vi "BIMS_Collector (2015_06).vi"() -> ()   [LabVIEW 2015]
doc: "This program is currently beta software. It is designed to address the data requirements defined primarily by the DHB Ballistic Test Report.\n\nThe general operation of this program is based on the Ballistics Version 2005 application developed internally by DuPont as a research tool for the Spruance Plant Ballistics Lab in Richmond, VA.\n\nPlease note that the original trigger control logic was modified and no longer depends on a safety interlock system to enable operation of a ballistic test.\n\nDuPont makes no warranties and assumes no liabilities in connection with any use of this program."
uses:
  DataSource.ctl
  shotsArr.ctl
  Shot Record.ctl
  Collector State.ctl
  <vilib>/Utility/error.llb/DialogType.ctl
  <vilib>/registry/registry.llb/Registry RtKey.ctl
  <vilib>/DAQmx/read.llb/DAQmx Read (Counter DBL 1Chan 1Samp).vi
  BIMS_Collector Globals.vi
  <vilib>/Utility/config.llb/Write Key (String).vi
  <vilib>/addons/database/Connection.llb/DB Tools Open Connec (Path).vi
  <vilib>/addons/database/Connection.llb/Conn Execute.vi
  <vilib>/addons/database/Recordset.llb/Rec Destroy - Connection.vi
  <vilib>/DAQmx/miscellaneous.llb/DAQmx Fill In Error Info.vi
  <vilib>/addons/database/NI_Database_API.lvlib
  <vilib>/Utility/config.llb/NI_LVConfig.lvlib
  <vilib>/Utility/file.llb/Write To Spreadsheet File (string).vi
panel:
  in  "diagPageVisible":bool
  in  "runtimeMenusVisible":bool=TRUE
  out "loadStatus":string
  out "Loading":u16(ring)
  in  "RESET All":bool
  out "ConfigName":string
  out "TimeNow":string
  in  "EXIT":bool
  in  "mainTabCntrl":enum32{"Setup", "Measure", "History", "System"}(tab)=enum."System"
  in  "SampleEntryTabCntrl":enum32{"Environment", "Sample"}(tab)
  in  "ThreatDetails":u16(ring) caption="Detail"
  in  "ThreatGroups":u16(ring) caption="Group"
  in  "PowderTypes":u16(ring) caption="Type"
  in  "Ballisticians":u16(ring) caption="Laboratorists"
  in  "Recorders":u16(ring) caption="Recorder"
  in  "Shooters":u16(ring) caption="Shooter"
  in  "Methods":u16(ring) caption="Method"
  in  "RoomT":sgl caption="Temperature (° C)" format="%.1f"
  in  "RoomHum":sgl caption="Humidity (%)" min=0 max=100 format="%.1f"
  in  "SampleBackings":u16(ring)=3 caption="Type"
  in  "clayCalArray":i16[](array[numeric])=[0, 0, 0, 0, 0] caption="Calibration (mm)" min=0 max=99 format="%02.0f"
  out "clayAverage":sgl caption="Clay Average (mm)" format="%#.1f"
  in  "clayTemp":sgl caption="Clay Temp (° F)" format="%.1f"
  out "threatDetails":T1 caption="Description"
  in  "SampleClamping":u16(ring) caption="Clamping"
  in  "Sample SubTabCntrl":T2(tab)
  in  "SampleID":string caption="Sample ID"
  in  "SampleDimensions":u16(ring) caption="Dimensions"
  in  "ModelMfrs":u16(ring) caption="Manufacturer"
  in  "SampleTypes":u16(ring) caption="Sample Type"
  in  "Submitters":u16(ring) caption="Submitter"
  in  "ProjectID":string caption="Project ID"
  in  "BackLayers":i32 caption="# of Layers" min=0 max=99 step=5
  in  "FrontLayers":i32 caption="# of Layers" min=0 max=99 step=5
  in  "BackLayer":u16(ring) caption="Back Layer"
  in  "FrontLayer":u16(ring) caption="Front Layer"
  out "totalNumLayers":i32 caption="Total # of Layers" min=0 max=100 step=5
  out "totalBAW":sgl caption="Total BAW (psf)" format="%.2f"
  in  "LayerTabControl":enum32{"1", "2", "3", "4", "5", "6"}(tab) caption="Inner Layers"
  out "fab1_totalWt":sgl caption="Fab1 Wt" min=0 max=99 step=5 format="%.2f"
  out "SampleAttribs_1":T3 caption="fabricAttribs_1"
  in  "Layer_1":T4 caption="Fabric #1" {"plyNum" min=0}
  in  "SampleStyle_1":u16(ring)
  in  "Mfr_1":u16(ring) caption="vendor" items=["", "3M", "A&P Technology", "Absecon Mills", "ABT Sciences", "Aermet", "ArmorStruxx", "Artec", "Axiom", "BAE Advanced Ceramics", "Barrday", "BGF", "Citterio", "Coors-Tek", "DSM", "DuPont", "DuPont (JPS-SUBC)", "FTC", "Gentex", "Gurit", "Hexcel", "Honeywell", "JD Lincoln", "JPS-Alexium", "JPS-Apjet", "JPS-DuPont", "JPS-Huntsman", "JPS-Old Hickory", "JPS-TSG", "Kamenskvolokno", "Loctite", "Lord", "LTC", "Marcus Materials", "McMaster-Carr", "Nanocomp", "Neva", "Nolax", "OConnell", "Patriot 3", "PATZ", "PBO", "Polystrand", "Pro-Systems", "ProTech", "Rusar", "Saati", "Saint Gobain", "S-Bond", "SEAL", "Sioux", "SPDW", "TechFiber", "Teijin", "Tencate", "Tensylon", "TexTech", "Toray", "TWARON", "UNKNOWN", "VonWeiss", "Xymid", "Z11"]
  in  "layerStitch_1":u16(ring) caption="Stitch"
  out "fab2_totalWt":sgl caption="Fab2 Wt" min=0 max=99 step=5 format="%.2f"
  out "SampleAttribs_2":T3 caption="fabricAttribs_2"
  in  "Layer_2":T4 caption="Fabric #2" {"plyNum" min=0}
  in  "SampleStyle_2":u16(ring)
  in  "Mfr_2":u16(ring) caption="vendor" items=["", "3M", "A&P Technology", "Absecon Mills", "ABT Sciences", "Aermet", "ArmorStruxx", "Artec", "Axiom", "BAE Advanced Ceramics", "Barrday", "BGF", "Citterio", "Coors-Tek", "DSM", "DuPont", "DuPont (JPS-SUBC)", "FTC", "Gentex", "Gurit", "Hexcel", "Honeywell", "JD Lincoln", "JPS-Alexium", "JPS-Apjet", "JPS-DuPont", "JPS-Huntsman", "JPS-Old Hickory", "JPS-TSG", "Kamenskvolokno", "Loctite", "Lord", "LTC", "Marcus Materials", "McMaster-Carr", "Nanocomp", "Neva", "Nolax", "OConnell", "Patriot 3", "PATZ", "PBO", "Polystrand", "Pro-Systems", "ProTech", "Rusar", "Saati", "Saint Gobain", "S-Bond", "SEAL", "Sioux", "SPDW", "TechFiber", "Teijin", "Tencate", "Tensylon", "TexTech", "Toray", "TWARON", "UNKNOWN", "VonWeiss", "Xymid", "Z11"]
  in  "layerStitch_2":u16(ring) caption="Stitch"
  out "fab3_totalWt":sgl caption="Fab3 Wt" min=0 max=99 step=5 format="%.2f"
  out "SampleAttribs_3":T3 caption="fabricAttribs_3"
  in  "Layer_3":T4 caption="Fabric #3" {"plyNum" min=0}
  in  "SampleStyle_3":u16(ring)
  in  "Mfr_3":u16(ring) caption="vendor" items=["", "3M", "A&P Technology", "Absecon Mills", "ABT Sciences", "Aermet", "ArmorStruxx", "Artec", "Axiom", "BAE Advanced Ceramics", "Barrday", "BGF", "Citterio", "Coors-Tek", "DSM", "DuPont", "DuPont (JPS-SUBC)", "FTC", "Gentex", "Gurit", "Hexcel", "Honeywell", "JD Lincoln", "JPS-Alexium", "JPS-Apjet", "JPS-DuPont", "JPS-Huntsman", "JPS-Old Hickory", "JPS-TSG", "Kamenskvolokno", "Loctite", "Lord", "LTC", "Marcus Materials", "McMaster-Carr", "Nanocomp", "Neva", "Nolax", "OConnell", "Patriot 3", "PATZ", "PBO", "Polystrand", "Pro-Systems", "ProTech", "Rusar", "Saati", "Saint Gobain", "S-Bond", "SEAL", "Sioux", "SPDW", "TechFiber", "Teijin", "Tencate", "Tensylon", "TexTech", "Toray", "TWARON", "UNKNOWN", "VonWeiss", "Xymid", "Z11"]
  in  "layerStitch_3":u16(ring) caption="Stitch"
  out "fab4_totalWt":sgl caption="Fab4 Wt" min=0 max=99 step=5 format="%.2f"
  out "SampleAttribs_4":T3 caption="fabricAttribs_4"
  in  "Layer_4":T4 caption="Fabric #4" {"plyNum" min=0}
  in  "SampleStyle_4":u16(ring)
  in  "Mfr_4":u16(ring) caption="vendor" items=["", "3M", "A&P Technology", "Absecon Mills", "ABT Sciences", "Aermet", "ArmorStruxx", "Artec", "Axiom", "BAE Advanced Ceramics", "Barrday", "BGF", "Citterio", "Coors-Tek", "DSM", "DuPont", "DuPont (JPS-SUBC)", "FTC", "Gentex", "Gurit", "Hexcel", "Honeywell", "JD Lincoln", "JPS-Alexium", "JPS-Apjet", "JPS-DuPont", "JPS-Huntsman", "JPS-Old Hickory", "JPS-TSG", "Kamenskvolokno", "Loctite", "Lord", "LTC", "Marcus Materials", "McMaster-Carr", "Nanocomp", "Neva", "Nolax", "OConnell", "Patriot 3", "PATZ", "PBO", "Polystrand", "Pro-Systems", "ProTech", "Rusar", "Saati", "Saint Gobain", "S-Bond", "SEAL", "Sioux", "SPDW", "TechFiber", "Teijin", "Tencate", "Tensylon", "TexTech", "Toray", "TWARON", "UNKNOWN", "VonWeiss", "Xymid", "Z11"]
  in  "layerStitch_4":u16(ring) caption="Stitch"
  out "fab5_totalWt":sgl caption="Fab5 Wt" min=0 max=99 step=5 format="%.2f"
  out "SampleAttribs_5":T3 caption="fabricAttribs_5"
  in  "Layer_5":T4 caption="Fabric #5" {"plyNum" min=0}
  in  "SampleStyle_5":u16(ring)
  in  "Mfr_5":u16(ring) caption="vendor" items=["", "3M", "A&P Technology", "Absecon Mills", "ABT Sciences", "Aermet", "ArmorStruxx", "Artec", "Axiom", "BAE Advanced Ceramics", "Barrday", "BGF", "Citterio", "Coors-Tek", "DSM", "DuPont", "DuPont (JPS-SUBC)", "FTC", "Gentex", "Gurit", "Hexcel", "Honeywell", "JD Lincoln", "JPS-Alexium", "JPS-Apjet", "JPS-DuPont", "JPS-Huntsman", "JPS-Old Hickory", "JPS-TSG", "Kamenskvolokno", "Loctite", "Lord", "LTC", "Marcus Materials", "McMaster-Carr", "Nanocomp", "Neva", "Nolax", "OConnell", "Patriot 3", "PATZ", "PBO", "Polystrand", "Pro-Systems", "ProTech", "Rusar", "Saati", "Saint Gobain", "S-Bond", "SEAL", "Sioux", "SPDW", "TechFiber", "Teijin", "Tencate", "Tensylon", "TexTech", "Toray", "TWARON", "UNKNOWN", "VonWeiss", "Xymid", "Z11"]
  in  "layerStitch_5":u16(ring) caption="Stitch"
  out "fab6_totalWt":sgl caption="Fab6 Wt" min=0 max=99 step=5 format="%.2f"
  out "SampleAttribs_6":T3 caption="fabricAttribs_6"
  in  "Layer_6":T4 caption="Fabric #6" {"plyNum" min=0}
  in  "SampleStyle_6":u16(ring)
  in  "Mfr_6":u16(ring) caption="vendor" items=["", "3M", "A&P Technology", "Absecon Mills", "ABT Sciences", "Aermet", "ArmorStruxx", "Artec", "Axiom", "BAE Advanced Ceramics", "Barrday", "BGF", "Citterio", "Coors-Tek", "DSM", "DuPont", "DuPont (JPS-SUBC)", "FTC", "Gentex", "Gurit", "Hexcel", "Honeywell", "JD Lincoln", "JPS-Alexium", "JPS-Apjet", "JPS-DuPont", "JPS-Huntsman", "JPS-Old Hickory", "JPS-TSG", "Kamenskvolokno", "Loctite", "Lord", "LTC", "Marcus Materials", "McMaster-Carr", "Nanocomp", "Neva", "Nolax", "OConnell", "Patriot 3", "PATZ", "PBO", "Polystrand", "Pro-Systems", "ProTech", "Rusar", "Saati", "Saint Gobain", "S-Bond", "SEAL", "Sioux", "SPDW", "TechFiber", "Teijin", "Tencate", "Tensylon", "TexTech", "Toray", "TWARON", "UNKNOWN", "VonWeiss", "Xymid", "Z11"]
  in  "layerStitch_6":u16(ring) caption="Stitch"
  in  "SampleCoverings":u16(ring) caption="Sample Covering" items=["None", "RipStop", "Plastic bag", "Other"]
  in  "Assemblers":u16(ring) caption="Technician"
  in  "Thickness":dbl caption="Thickness (mm)" format="%.3f"
  in  "totalSampleWt":sgl caption="Total Weight (g)" format="%.3f"
  in  "Comments":string caption="Remarks (optional):"
  in  "TestConditions":u16(ring) caption="Sample Condition"
  in  "shotsTabCntrl":T5(tab)
  in  "2ndScreen":bool=TRUE caption="Enabled"
  out "cntDn":i32
  in  "Frag Rod":sgl format="%.1f"
  in  "Drag Corrected":bool=TRUE
  out "Impact/speed":sgl caption="Chronograph 1" min=0 max=10000 step=0.1 format="%.1f"
  out "residual/speed":sgl caption="Residual" min=0 max=10000 step=0.1 format="%.1f"
  in  "MeasVelScrnSet1":sgl caption="Set #1" min=0 max=10000 step=0.1 format="%.1f"
  in  "Current/shotstatus":u16(ring) caption="Penetration" items=["Partial", "Complete"]
  in  "Current/residual/speed":sgl caption="Residual Set" min=0 max=10000 step=0.1 format="%.1f"
  in  "shotTimestamp":string caption="Date/Time"
  in  "MeasVelScrnSet2":sgl caption="Set #2" min=0 max=1000000 step=0.1 format="%.1f"
  out "%_Difference":sgl caption="% Vel Diff" format="%.3f"
  in  "backdepth":sgl caption="BF Depth"
  out "Redundant/speed":sgl caption="Chronograph 2" min=0 max=10000 step=0.1 format="%.1f"
  out "Current/avg/speed":sgl caption="Average" min=0 max=1000000 step=0.1 format="%.1f"
  out "Avg/speed":sgl caption="Average" min=0 max=10000 step=0.1 format="%.1f"
  out "DC_ factor":sgl=1.0 caption="DC Factor" format="%.4f"
  in  "Barrel Temp":sgl format="%.1f"
  in  "Shot Description":string caption="Description (optional)"
  in  "Powder Loading":sgl caption="Powder Load" min=0 max=100 step=0.1 format="%.3f"
  in  "Shot Angle":u16 max=90 step=1
  out "Projectile Mass":sgl caption="Projectile Mass (grains)" min=0 step=1
  in  "N.I.J":u16(ring) items=["n/a", "PASS", "FAIL"]
  in  "addShot":bool caption="RANGE SETUP must be selected before shots can be added."
  in  "loadingUnits":enum32{"grams", "grains"}(radio)
  out "instruct_addShot":string="RANGE SETUP and THREAT must be selected before shots can be added."
  out "Set#1 Separation":sgl=1.0 caption="Outer" format="%.2f"
  out "Set#2 Separation":sgl=1.0 caption="Inner" format="%.2f"
  out "ARMED":bool caption="Armed"
  out "velSTDEV":sgl caption="Standard Deviation" min=0 max=10000 step=1 format="%.1f"
  out "saveReq":string="Number of layers in sample ply specification and number of shots in shots table must be greater than 0 to enable saving."
  in  "VsVr Report":bool caption="Report"
  out "Table of Shots":string[][](table) caption="Shot Table"
  in  "MC Listbox of Shots":i32(listbox)
  in  "saveShots":bool
  in  "clearShots":bool
  out "highPartial":i32 caption="High Partial" min=0 max=10000 step=1
  out "lowComplete":i32 caption="Low Complete" min=0 max=10000 step=1
  out "rangeOfResults":i32 caption="Range of Results" min=0 max=10000 step=1
  out "zmr 2":sgl caption="Low C minus High P" format="%.1f"
  out "computed_V50":sgl caption="V50  (m/s)" format="%.1f"
  out "Pairs":i16 min=0 max=100 step=1
  in  "reportV50":bool caption="Report"
  in  "maxDev":sgl=10.0 caption="Max Deviation (m/s)" min=0 max=100 format="%.1f"
  in  "undoLastShot":bool
  in  "deleteShot":bool
  in  "nextShot":bool
  in  "shotsArr":T6 {"Frag Rod" format="%.1f"; "UncorrectedAvgVel_PB" format="%.1f"; "UncorrectedRed_PB" format="%.1f"; "strikeVel_PB" format="%.1f"; "velLoss_PB" format="%.1f"; "avgVel_PB" format="%.1f"; "Redundant_Velocity" format="%.1f"; "Energy Loss (J)" format="%.3e"; "Projectile Mass" min=0 step=1 format="%.4f"; "Corrected residual" format="%.2f"; "Uncorrected Residual" format="%.1f"; "Corrected Impact" format="%.2f"; "Uncorrected Impact" format="%.1f"; "Shot Angle" max=90 step=1; "SHOT STATUS" items=["Partial", "Complete"]; "IMPACT VELOCITY" min=0 max=10000 step=0.1 format="%.1f"; "Barrel Temperature" format="%.1f"; "Powder Loading" format="%.4f"; "RESIDUAL  VELOCITY" min=0 max=10000 step=0.1 format="%.1f"}
  out "velProfile":cluster{dbl, dbl}[](graph) caption="Shot Velocity Measurement Profile"
  out "velCompProf":cluster{"vStrike":dbl, "vA":dbl} caption="Velocity in fps\n(computed)"
  out "velMeasProf":T8 caption="Velocity in fps\n(measured)"
  out "relativeTime":cluster{"ts2":dbl, "ts3":dbl, "ts1":dbl} caption="Relative time\n(microsec)"
  out "displacement":T9={"ds_v2"=6.75, "ds2"=5.0833, "ds_vB"=4.9167, "ds3"=4.75, "ds_vAvg"=6.9167, "ds_v1"=7.0833, "ds1"=8.75, "ds_vA"=8.9167, "ds0"=9.0833} caption="Distance from\ntarget (ft)" {"ds0" format="%_4g"; "ds_vA" format="%_4g"; "ds1" format="%_4g"; "ds_v1" format="%_4g"; "ds_vAvg" format="%_4g"; "ds3" format="%_4g"; "ds_vB" format="%#_4g"; "ds2" format="%#_4g"; "ds_v2" format="%_4g"}
  out "arrIDC":dbl[](array[numeric]) caption="Instantaneous Drag Coefficient"
  in  "rangeSetup":u16(ring)=1 caption="Range Dimensions" items=["Short (small frag)", "Standard (handgun)", "Long (rifle)"]
  out "mid_to_targ_dist":sgl=5.0 caption="Mid To Target (ft)"
  in  "historyTabCntrl":enum32{"Powder Loading", "Panel Search"}(tab)=enum."Panel Search"
  in  "Threat.freeTxt":string caption="Threat"
  in  "Powder.freeTxt":string caption="Powder"
  in  "QueryLoad":bool
  in  "lkupEndDate":timestamp caption="End Date" format="%<%x>T"
  in  "lkupStartDate":timestamp caption="Begin Date" format="%<%x>T"
  out "Vel.vs.Loading":cluster{dbl[], dbl[]}(graph)
  out "v50_table":string[][](table)
  in  "maxRecs":u16=1001 caption="Max # of SHOT Records" min=1 max=10000 step=100
  out "ActualNumRecs":i32=1001 caption="Actual # Returned"
  in  "ThreatSize_0":u16(ring) caption="Threat Size" items=["", "2", "4", "16", "17", "44", "55", "62", "64", "85", "123", "124", "125", "148", "158", "166", "180", "207", "240"]
  in  "panelSearch":bool
  in  "Mfr_0":u16(ring) caption="Manufacturer" items=["", "3M", "A&P Technology", "Absecon Mills", "ABT Sciences", "Aermet", "ArmorStruxx", "Artec", "Axiom", "BAE Advanced Ceramics", "Barrday", "BGF", "Citterio", "Coors-Tek", "DSM", "DuPont", "DuPont (JPS-SUBC)", "FTC", "Gentex", "Gurit", "Hexcel", "Honeywell", "JD Lincoln", "JPS-Alexium", "JPS-Apjet", "JPS-DuPont", "JPS-Huntsman", "JPS-Old Hickory", "JPS-TSG", "Kamenskvolokno", "Loctite", "Lord", "LTC", "Marcus Materials", "McMaster-Carr", "Nanocomp", "Neva", "Nolax", "OConnell", "Patriot 3", "PATZ", "PBO", "Polystrand", "Pro-Systems", "ProTech", "Rusar", "Saati", "Saint Gobain", "S-Bond", "SEAL", "Sioux", "SPDW", "TechFiber", "Teijin", "Tencate", "Tensylon", "TexTech", "Toray", "TWARON", "UNKNOWN", "VonWeiss", "Xymid", "Z11"]
  in  "SampleStyle_0":u16(ring) caption="Sample Style"
  in  "srchParams":T10={"maxPanels"=1001, "lkupPanelStartDate"=timestamp(0 s since 1904-01-01), "lkupPanelEndDate"=timestamp(3376658114.0909824 s since 1904-01-01)} {"lkupPanelEndDate" format="%<%x>T"; "lkupPanelStartDate" format="%<%x>T"; "maxPanels" min=1 max=10000 step=100}
  out "actualNumPanels":i32 caption="Actual # Returned"
  out "pastPanels":string[][](table)
  in  "Record #":i32=1 min=0 max=60857
  in  "reportV50_History":bool
  out "SampleAttribs_0":T11 caption="fabricAttribs_1"
  in  "Requestors_0":u16(ring) caption="Submitter"
  in  "aboutTabCntrl":enum32{"About ", "Internal Use"}(tab)
  in  "RefreshMetadata":bool
  out "lastShot":i32 caption="Shot"
  out "lastSamp":i32 caption="Sample"
  in  "PublishNewRecords":bool
  in  "internal":enum32{"ctr", "deploy", "misc"}(tab)=enum."misc"
  out "taskCtr1":refnum<k21>
  in  "ctr1":tag="LightScreens/ctr1"
  in  "readyClock":bool caption="Clock"
  in  "ActiveDev":tag="LightScreens"
  in  "ctr0":tag="LightScreens/ctr0"
  in  "SampClk.Timebase.Src":tag="/LightScreens/80MHzTimebase"
  out "Device S/N":string
  in  "MeasSrc":T12=enum."Screens" caption="Source"
  in  "ARM":bool
  out "errCtr0":errorcluster
  out "errCtr1":errorcluster
  out "taskCtr0":refnum<k21>
  in  "Folder":string caption="Publish Folder"
  in  "useBMC":bool caption="Use Message Center?"
  in  "Server":string
  in  "Site":string
  in  "InterlockExists":bool=TRUE caption="Safety Interlock Hardware Exist?"
  in  "ScreenSetAvgg":bool=TRUE caption="Average Screen Sets?"
  in  "Sort by AVG":bool=TRUE caption="Sort shots by average velocity"
  in  "useBallisitican":bool=TRUE caption="Use Ballistician field in Setup?"
  in  "useRecorder":bool caption="Use Recorder field in Setup?"
  in  "useShooter":bool caption="Use Shooter field in Setup?"
  in  "close arming loop":bool
  out "progState":T13
  in  "clearErrors":bool
  in  "LayerStitchTypes":u16(ring) caption="Stitch"
  out "GrainSize":u16 caption="Grain"
  out "U/I EvErr":errorcluster
  out "SMErr":errorcluster
  in  "Models":u16(ring) caption="Model #" items=["n/a"]
  in  "serialNum":string caption="Serial #"
  in  "SampleDescrip":u16(ring) caption="Misc. Sample Description (legacy)"
  out "lengthUnits":string="FOOT" caption="Distance Units"
  out "massUnits":string="GRAMS" caption="Weight Units"
  in  "Threat":u16(ring) caption="Threat (long description)"
  in  "Type of work":string="QC"
  in  "minV50":i32=1500 caption="Minimum V50"
  out "configPath":path=path "P:/Private/My Projects/AFS/BIMS/2008/BIMS_Collector.ini" caption="Configuration Path (INI)"
  out "STOP (Shots MC LB)":bool=TRUE
  in  "lookupRec":bool caption="lookup"
  in  "clayCalib":string="##-##-##-##-##" caption="Calibration"
  in  "Fabric Description":string caption="Fabric Desc"
  in  "Areal density text":string
  in  "Areal Density":dbl format="%.2f"
  out "Residual factor":sgl=1.0 caption="Residual" min=0 max=1 format="%.5f"
  out "Impact factor":sgl=1.0 caption="Impact" min=0 max=1 format="%.5f"
  out "Partial":sgl[](array[numeric]) format="%.2f"
  out "factor array":sgl[](array[numeric]) format="%.4f"
  out "Complete":sgl[](array[numeric]) format="%.2f"
  in  "old threat":u16
  out "Z.M.R.":sgl min=0 step=0.1 format="%.1f"
  in  "Residual/Target Dist":sgl=7.083333 format="%.2f"
  out "Residual/Separation":sgl=4.0 format="%.2f"
  in  "Set#1_to_Target":sgl=7.083333 format="%.2f"
  out "Barrel to Screen":sgl=7.8333 format="%.2f"
  out "CorrectedVelScrnSet1":sgl=1503.981 format="%.2f"
  out "Corrected Residual":sgl=751.9905 format="%.2f"
  out "correction coefficient":sgl format="%.8f"
  in  "SoftwareVersion":dbl caption="Version" format="%.2f"
  in  "percent warning":sgl=1.0 format="%.2f"
  out "#_partials":i32
  out "#_completes":i32
  out "conversion factor":sgl=0.3048037 format="%.5f"
  out "CorrectedVelScrnSet2":sgl=1551.8816 caption="Corrected Redundant" format="%.2f"
  out "Corrected Average":sgl=1527.9313 format="%.2f"
  in  "processShots":bool caption="Proc Shots"
  in  "WeaponTypes":u16(ring) caption="Weapon" items=["", "Universal Receiver", "Other"]
  in  "TestStandards":u16(ring)=2 caption="Standard" items=["n/a", "NIJ 0101.04", "MIL-STD-662F"]
  out "SUBMIT DATE/TIME":string
  # "Effectively restarts the application from scratch, as if the user pressed the EXIT button and then restarted the application."
  # "Configured for"
  # "Threat"
  # "*"
  # "*"
  # "Test"
  # "Powder"
  # "*"
  # "Personnel"
  # "Room"
  # "*"
  # "Backing"
  # "*"
  # "*"
  # "*"
  # "Strike Face"
  # "Body Side"
  # "Layer"
  # "Mfr"
  # "Style"
  # "# of Plies"
  # "Lot"
  # "Roll"
  # "Stitch"
  # "Internal ID"
  # "Fiber"
  # "Denier"
  # "Construction"
  # "Weave"
  # "Finish"
  # "Basis weight (oz/yd²)"
  # "Yarn Merge"
  # "Total Weight"
  # "*"
  # "*"
  # "*"
  # "1"
  # "2"
  # "3"
  # "4"
  # "5"
  # "6"
  # "Required"
  # "*"
  # "Shot Parameters"
  # "cm"
  # "deg"
  # "° C"
  # "Screens\nSeparation"
  # "meters"
  # "Velocity Measurements"
  # "Observations"
  # "Table Functions"
  # "Summary"
  # "Reports"
  # "Test Record"
  # "Edit Shot Records"
  # "Corrected"
  # "Shot #"
  # "t0"
  # "0"
  # "S Strike"
  # "0"
  # "Internal ID#"
  # "Fiber"
  # "Denier"
  # "Pick"
  # "Weave"
  # "Finish"
  # "oz/yd²"
  # "Asset"
  # "DuPont Protection Technologies\nBallistics Information Management System\n\nBIMS\n\n\nSample Performance\nData Collector\n\nJune 21, 2015"
  # "DuET Measurement System Technologies\nDUCOM 8 695-2330 for technical support"
  # "Last Assigned\nRecord Numbers"
  # "Deployment Configuration"
  # "NI LabVIEW 2014 Ver 14.0.1 (32-bit)\nLast build on 06/22/2015"
  # "Correction Factors"
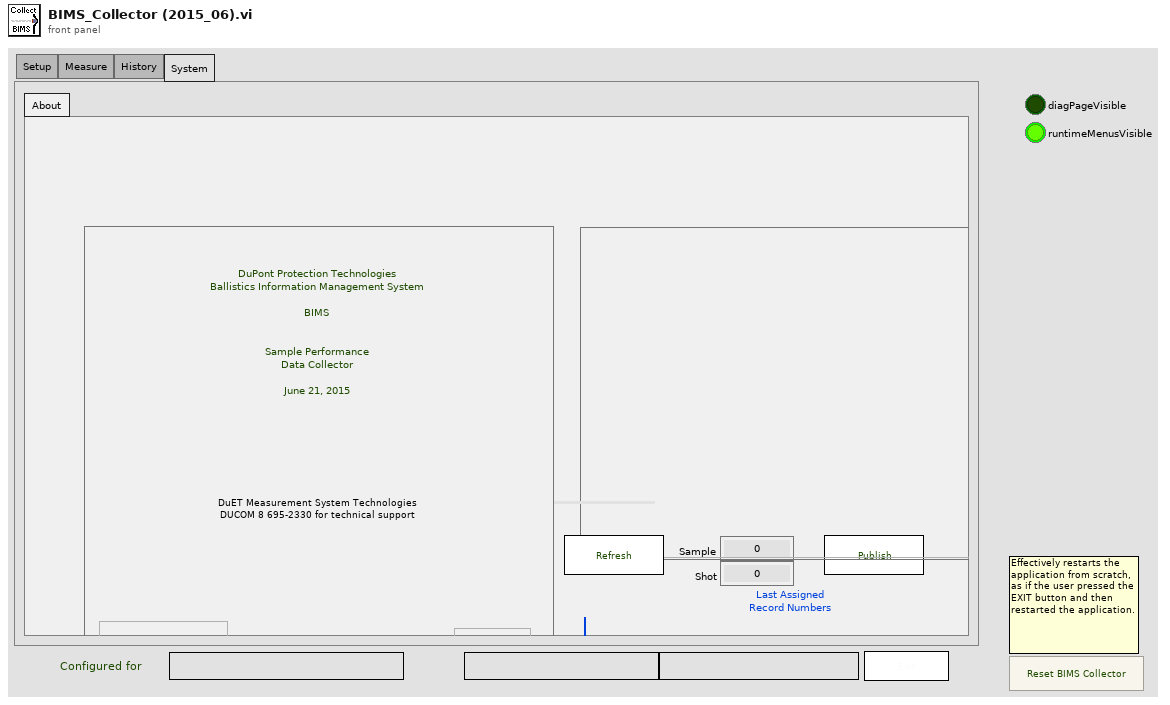
[diagram p1: front panel]
types:
  T1 = cluster{"barrelLength":string, "dragCorrection":string, "detailDescription":string, "barrelCaliber":string, "grainSize":string, "Make":string, "Model":string}
  T2 = enum32{"General Specification", "Ply Specification", "Preparation"}
  T3 = cluster{"Fabric.fiber":string, "Fabric.denier":string, "pick":string, "weave":string, "finish":string, "ozPerYd2":string, "fabricID_DHB":string, "yarnMerge":string}
  T4 = cluster{"plyNum":i32, "LotNum":string, "RollNum":string}
  T5 = enum32{"Ready-Aim-Fire", "Shots Table", "Edit", "Instantaneous DC"}
  T6 = typedef "shotsArr.ctl" = T7[]
  T7 = typedef "Shot Record.ctl" = cluster{"Uncorrected Impact":sgl, "Uncorrected Residual":sgl, "avgVel_PB":sgl, "IMPACT VELOCITY":sgl, "RESIDUAL  VELOCITY ":sgl, "Shot Description":string, "Powder Loading ":sgl, "Barrel Temperature":sgl, "TIME / DATE":string, "shot order":i32, "SHOT STATUS":u16, "Shot Angle":u16, "Corrected Impact":sgl, "Corrected residual":sgl, "Projectile Mass":sgl, "usedv50":bool, "Energy Loss (J)":sgl, "BackFace\nDepth":sgl, "BackFace\nDiameter":sgl, "Redundant_Velocity":sgl, "velLoss_PB":sgl, "strikeVel_PB":sgl, "UncorrectedRed_PB":sgl, "CorrectedRed_PB":sgl, "UncorrectedAvgVel_PB":sgl, "V50userExcl":bool, "Frag Rod":sgl}
  T8 = cluster{"v2":dbl, "vB":dbl, "vOuter":dbl, "v1":dbl, "vA":dbl, "vInner":dbl}
  T9 = cluster{"ds_v2":dbl, "ds2":dbl, "ds_vB":dbl, "ds3":dbl, "ds_vAvg":dbl, "ds_v1":dbl, "ds1":dbl, "ds_vA":dbl, "ds0":dbl}
  T10 = cluster{"maxPanels":u16, "lkupPanelStartDate":timestamp, "lkupPanelEndDate":timestamp}
  T11 = cluster{"Fabric.fiber":string, "Fabric.denier":string, "pick":string, "weave":string, "finish":string, "ozPerYd2":string, "fabricID_DHB":string, "asset":string}
  T12 = typedef "DataSource.ctl" = enum16{"Simulated", "Radar", "Screens"}
  T13 = typedef "Collector State.ctl" = enum16{"POLL", "INITIALIZE", "V50 Report or GET Record", "VsVr Report", "SAVE SHOTS", "ADD SHOT", "CLEAR SHOTS", "NEXT SHOT", "DELETE SHOT", "READY CLOCK", "PROC SHOTS", "CHECK DAQ"}
  T14 = typedef "DialogType.ctl" = u16
  T15 = enum8{"Enabled", "Disabled", "Disabled and Grayed Out"}
  T16 = enum32{"Page Enabled", "Page Disabled", "Page Disabled & Grayed"}
  T17 = enum32{"invalid app kind", "Development System", "Run Time System", "Student Edition", "Embedded LabVIEW", "Evaluation", "Custom"}
  T18 = typedef "LVRowAndColumnTypeDef.ctl" = cluster{"Row":i32, "Column":i32}
  T19 = cluster{"barrelLength":string, "dragCoefficient":string, "detailDescription":string, "barrelCaliber":string, "grainSize":string, "Make":string, "Model":string}
  T20 = cluster{"fiber":string, "denier":string, "construction":string, "weave":string, "finish":string, "ozPerYd2":string, "fabricStyle_DHB":string, "yarnMerge":string}
  T21 = cluster{"fiber":string, "denier":string, "pick":string, "weave":string, "finish":string, "ozPerYd2":string, "internal_ID":string, "asset":string}[]
  T22 = cluster{"plyNum":i32, "LotNum":string, "RollNum":string}[]
  T23 = typedef "NI_LVConfig.lvlib/Config Data RefNum.ctl" = refnum<k1>
  T24 = typedef "Registry RtKey.ctl" = enum32{"HKEY_CLASSES_ROOT", "HKEY_CURRENT_USER", "HKEY_LOCAL_MACHINE", "HKEY_USERS", "HKEY_PERFORMANCE_DATA", "HKEY_CURRENT_CONFIG", "HKEY_DYN_DATA"}
  T25 = cluster{"[0]":string, "[1]":string, "[2]":string, "[3]":string, "[4]":string, "[5]":string, "[6]":string, "[7]":string, "[8]":string, "[9]":string}[]
  T26 = cluster{"[0]":string, "[1]":string, "[2]":string, "[3]":string, "[4]":string, "[5]":string, "[6]":string, "[7]":string, "[8]":string}[]
  T27 = cluster{"Fabric.fiber":string, "Fabric.denier":string, "pick":string, "weave":string, "finish":string, "ozPerYd2":string, "fabricID_DHB":string, "yarnMerge":string}[]
  T28 = cluster{"Uncorrected Impact":bool, "Uncorrected Residual":bool, "avgVel_PB":bool, "IMPACT VELOCITY":bool, "RESIDUAL  VELOCITY ":bool, "Shot Description":bool, "Powder Loading ":bool, "Barrel Temperature":bool, "TIME / DATE":bool, "shot order":bool, "SHOT STATUS":bool, "Shot Angle":bool, "Corrected Impact":bool, "Corrected residual":bool, "Projectile Mass":bool, "usedv50":bool, "Energy Loss (J)":bool, "BackFace\nDepth":bool, "BackFace\nDiameter":bool, "Redundant_Velocity":bool, "velLoss_PB":bool, "strikeVel_PB":bool, "UncorrectedRed_PB":bool, "CorrectedRed_PB":bool, "UncorrectedAvgVel_PB":bool, "V50userExcl":bool, "Frag Rod":bool}
  T29 = cluster{"SampleTypes":refnum<vi>, "SampleDescrip":refnum<vi>}
  T30 = cluster{"max dev":sgl, "residual separation":sgl, "Set#1 Separation":sgl, "Set#2 Separation ":sgl, "impact target dist":sgl, "resid target dist":sgl, "barrel screen dist":sgl, "midpt_to_target_dist":sgl}
  T31 = cluster{"numOfPlies":i32, "LotNum":string, "RollNum":string}[]
  T32 = cluster{string, string, string, string, string, string, string, string, "clayCalib":string, string}
  T33 = cluster{string, string, string, string, string, string, string}
  T34 = cluster{"SampleID":string, "element":string, "Type of work":string, "serialNum":string, "element":string, string, string, string, "element":string, string}
  T35 = cluster{"SampleID":string, "element":string, string, string, string, "element":string}
  T36 = cluster{"[0]":string, "[1]":string, "[2]":string, "[3]":string, "[4]":string, "[5]":string, "[6]":string, "[7]":string, "[8]":string, "[9]":string}
  T37 = cluster{"[0]":string, "[1]":string, "[2]":string, "[3]":string, "[4]":string, "[5]":string, "[6]":string, "[7]":string, "[8]":string}
  T38 = cluster{"element":string, "element":string, "grainSize":string, "element":string, "barrelLength":string, string, "element":string, "element":string, "element":string}
  T39 = cluster{"element":string, "grainSize":string, "element":string, "barrelLength":string, string, "element":string}
  T40 = typedef "NI_Database_API.lvlib/Conn ObjectReference.ctl" = refnum<k1>
  T41 = typedef "NI_Database_API.lvlib/Rec ObjectReference.ctl" = refnum<k1>
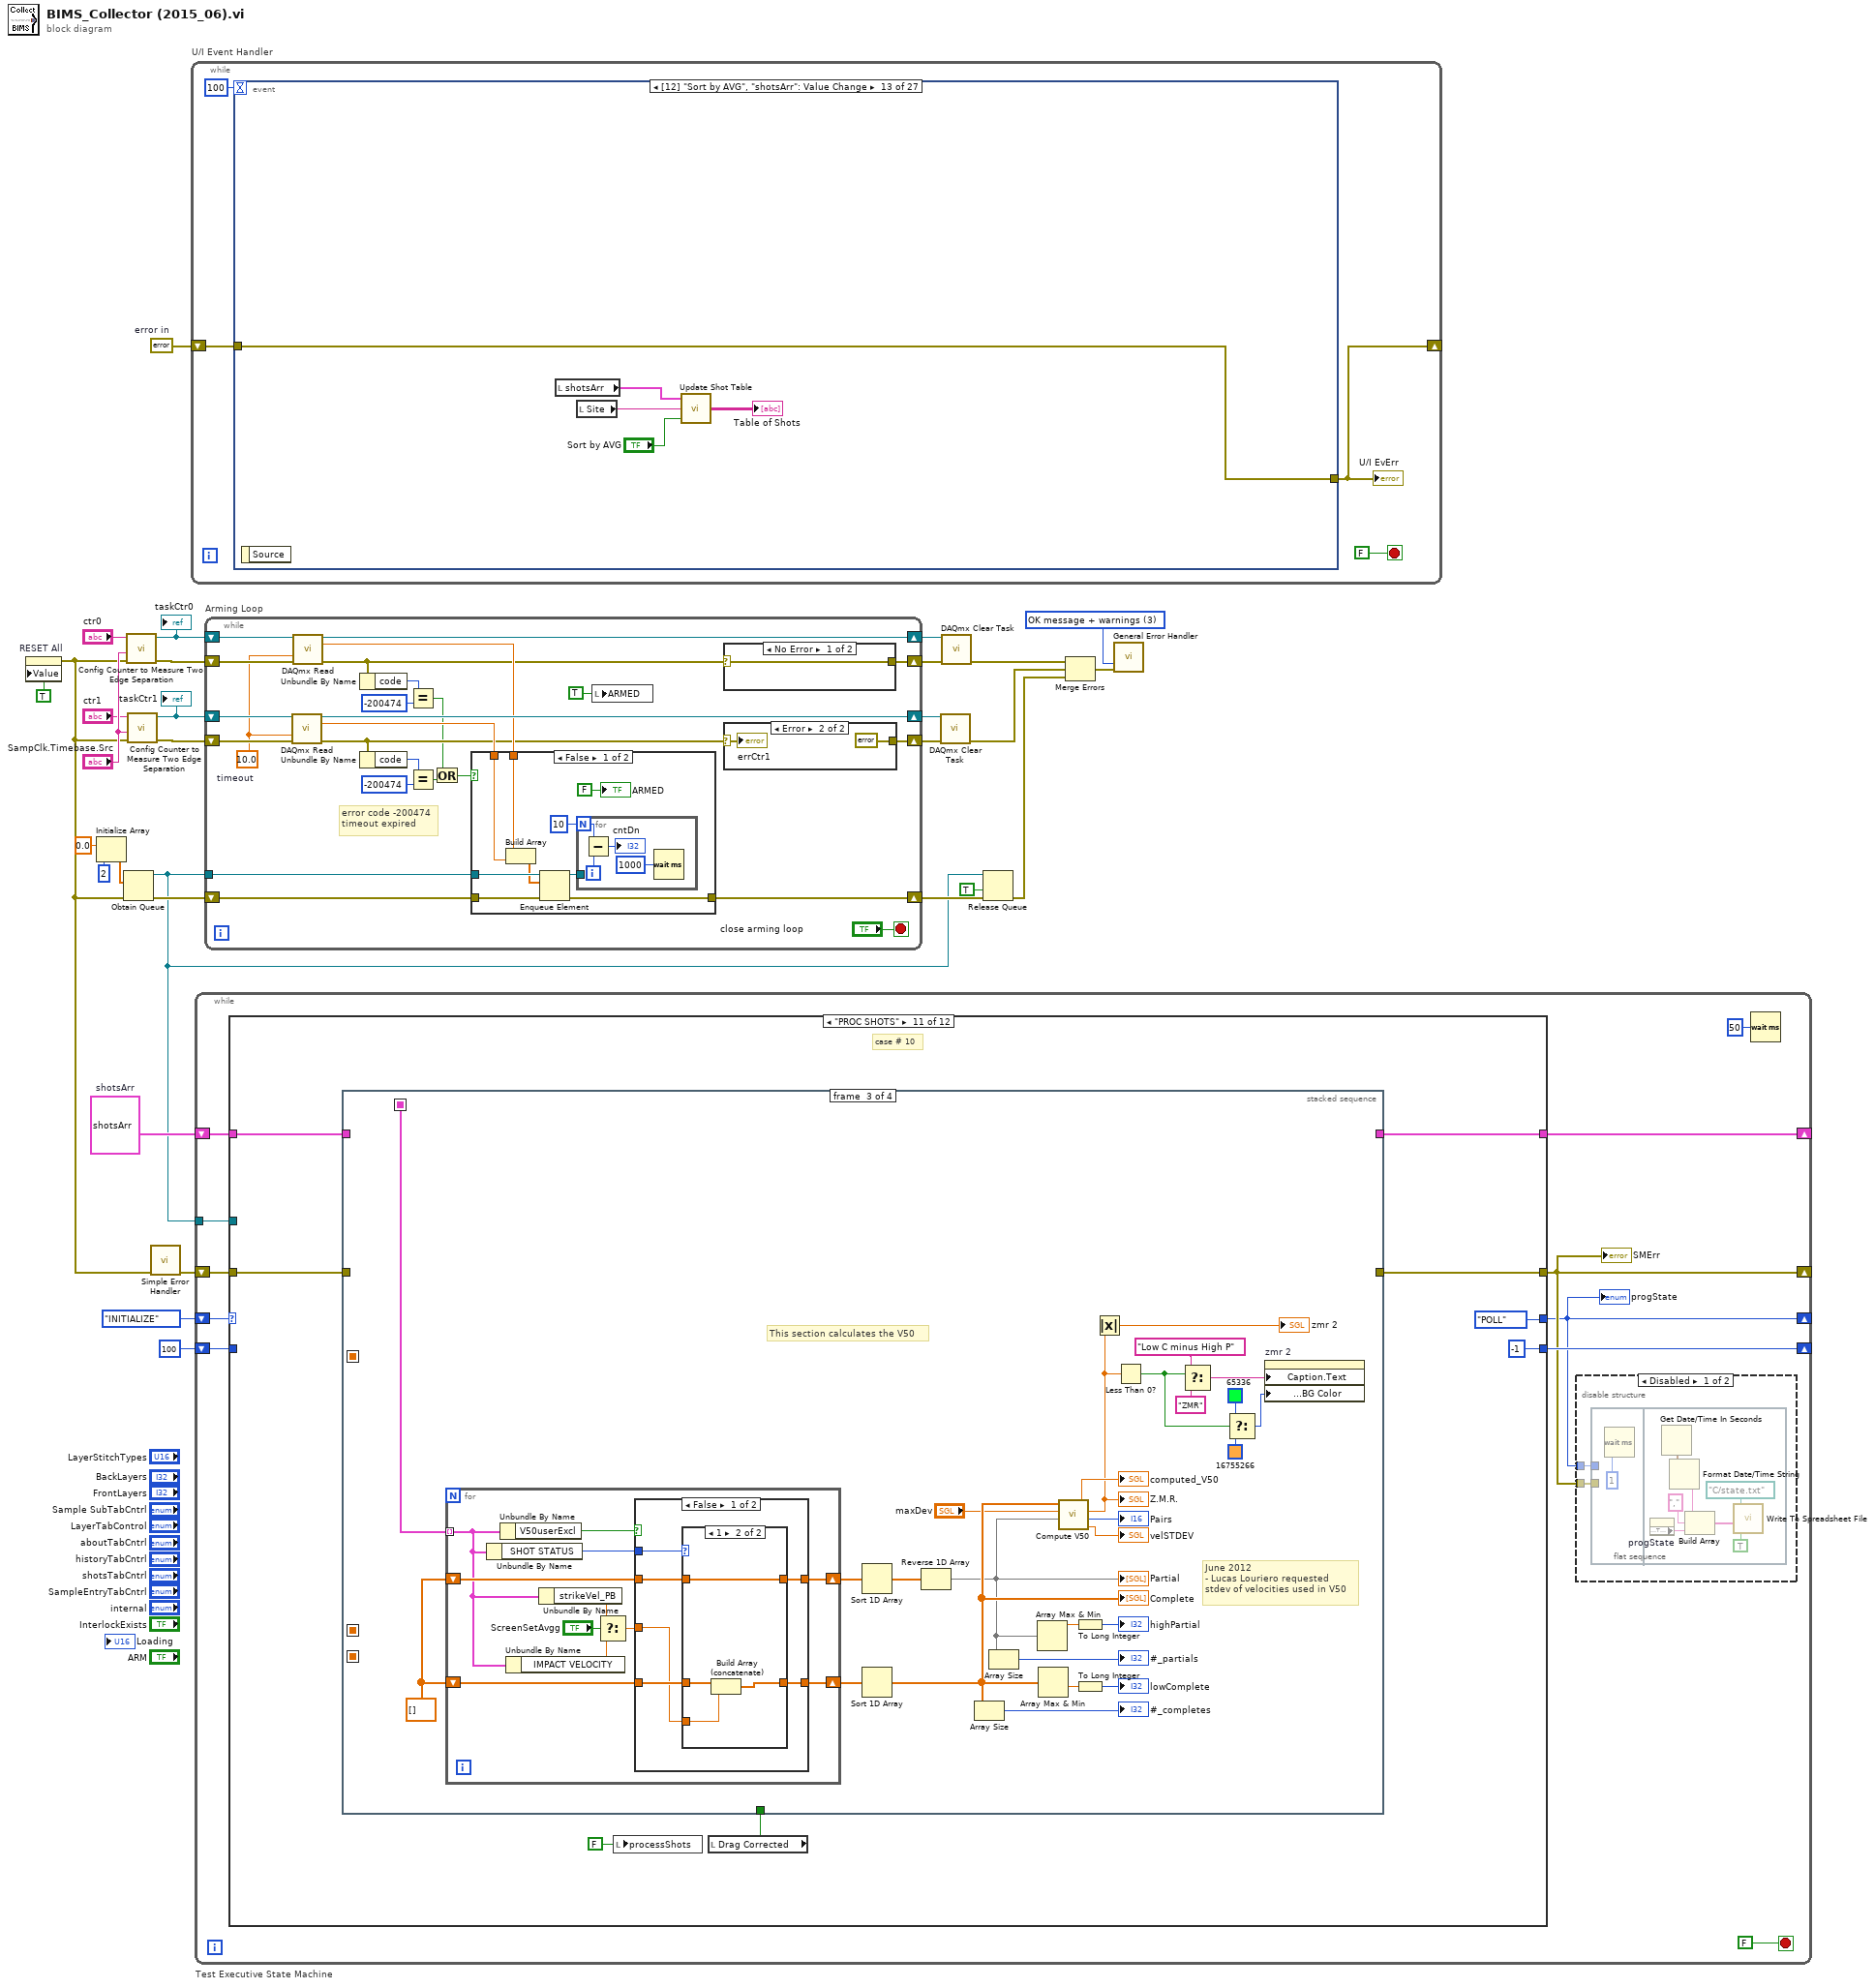
[diagram p0: block diagram]
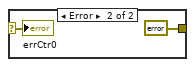
[diagram p4: hidden frame]
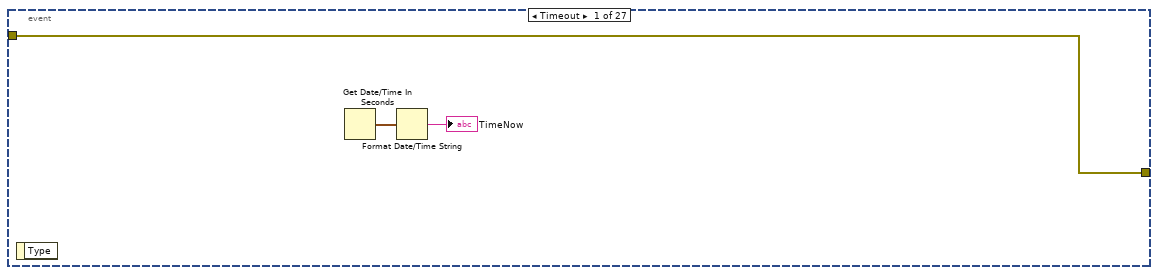
[diagram p5: hidden frame]
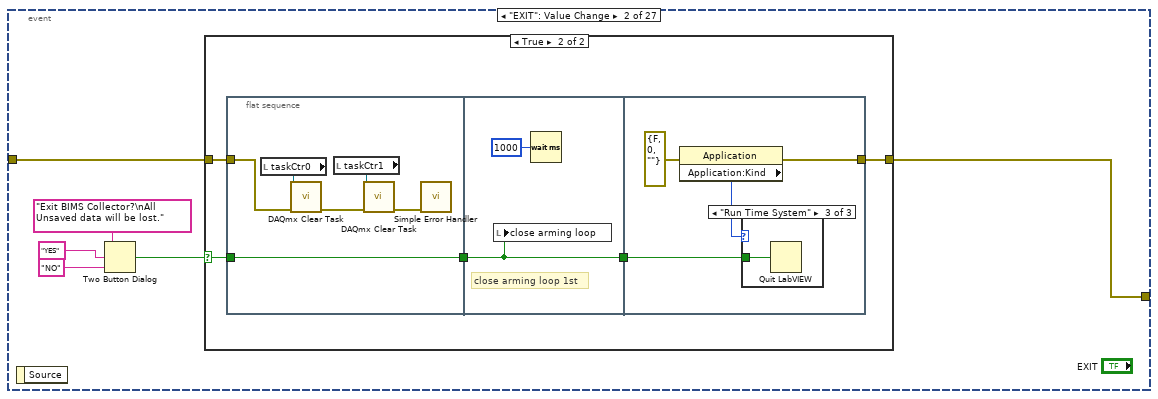
[diagram p6: hidden frame]
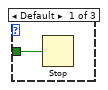
[diagram p8: hidden frame]
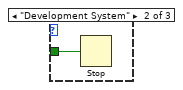
[diagram p9: hidden frame]
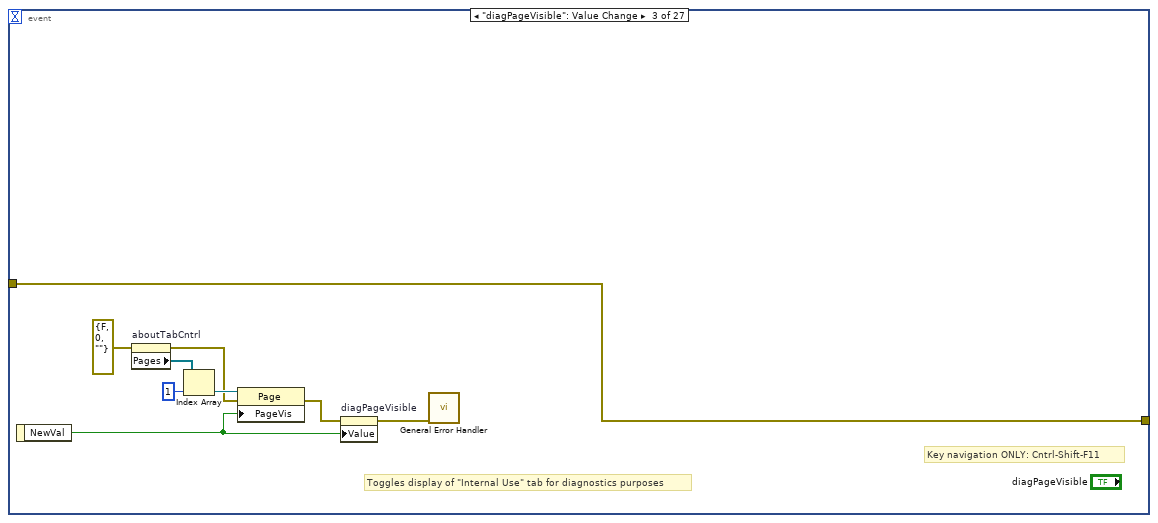
[diagram p10: hidden frame]
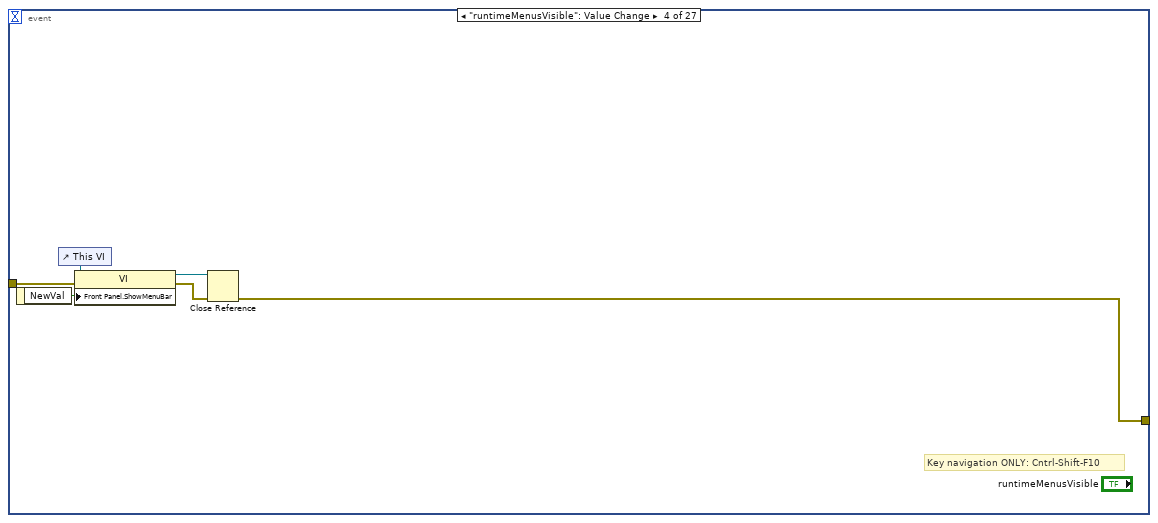
[diagram p11: hidden frame]
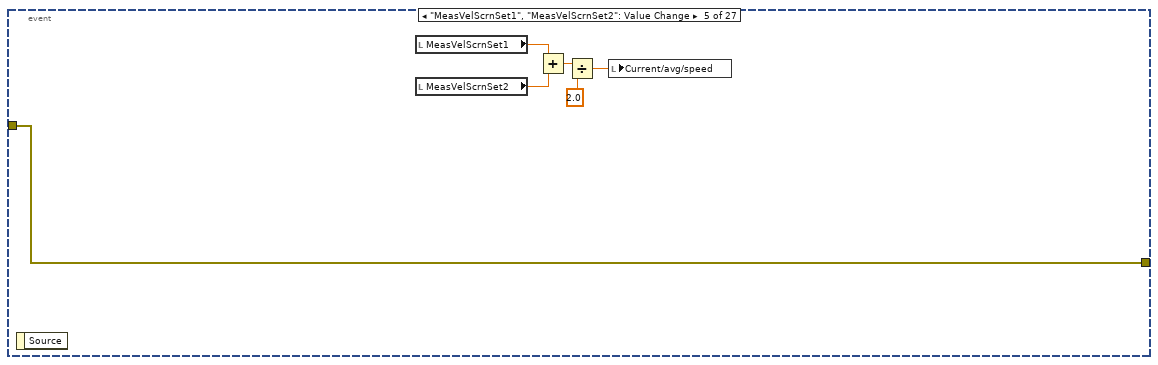
[diagram p12: hidden frame]
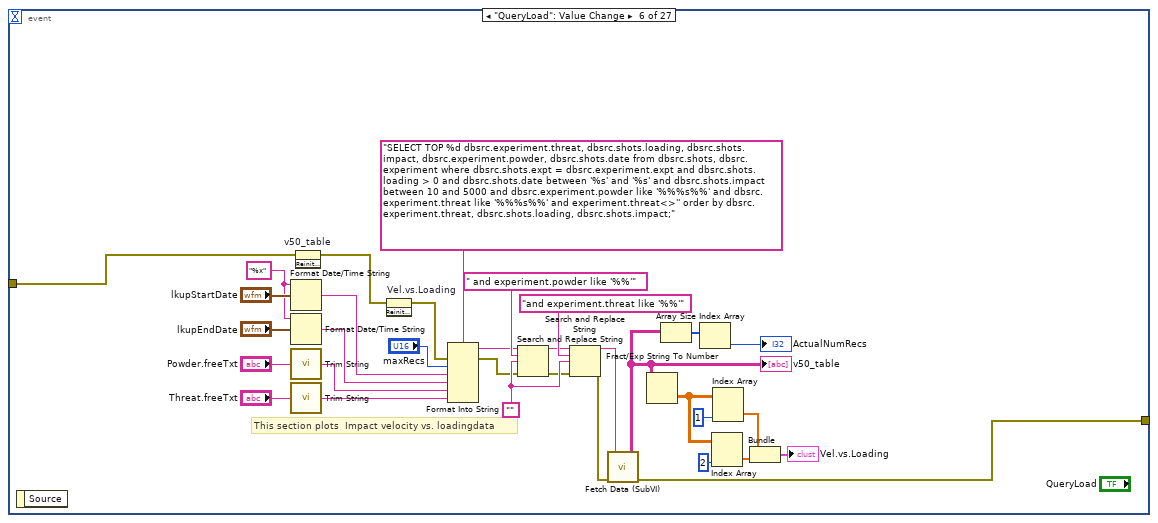
[diagram p13: hidden frame]
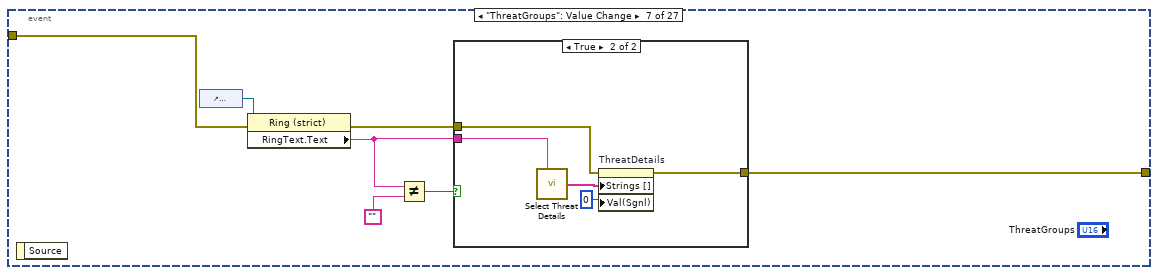
[diagram p14: hidden frame]
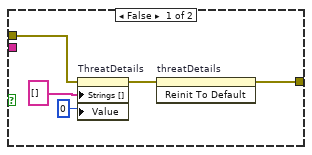
[diagram p15: hidden frame]
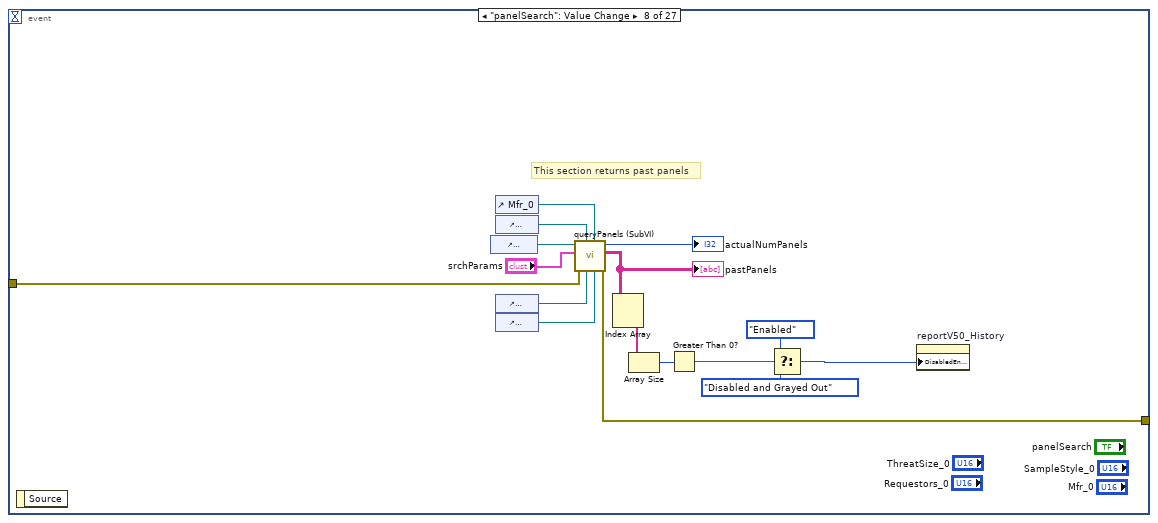
[diagram p16: hidden frame]
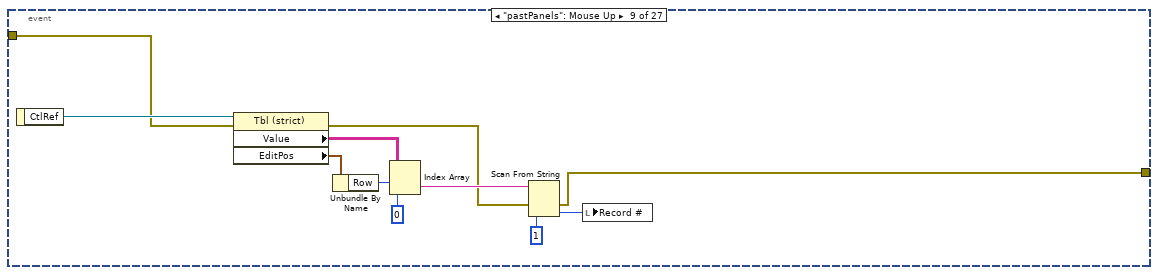
[diagram p17: hidden frame]
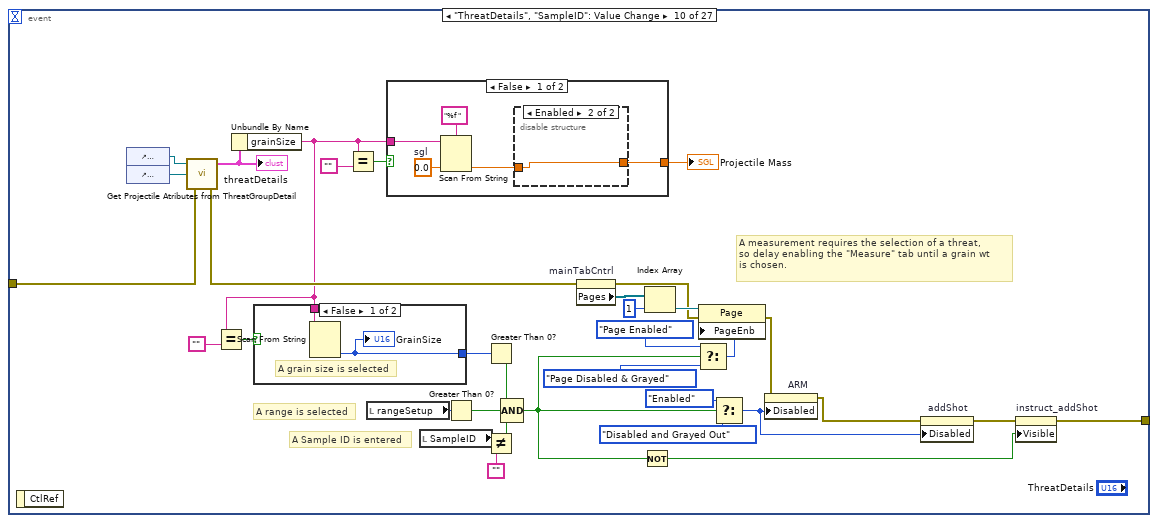
[diagram p18: hidden frame]
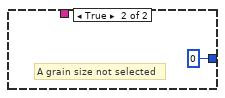
[diagram p19: hidden frame]
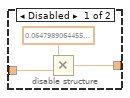
[diagram p20: hidden frame]
diagram:
  w16 = T14 3 items=["no dialog", "OK message", "continue or stop message", "OK message + warnings", "continue/stop + warnings"] ("type of dialog (OK msg:1)")
  w26 = T6 [{"Uncorrected Impact"=0.0, "Uncorrected Residual"=0.0, "avgVel_PB"=0.0, "IMPACT VELOCITY"=0.0, "RESIDUAL  VELOCITY "=0.0, "Shot Description"="", "Powder Loading "=0.0, "Barrel Temperature"=0.0, "TIME / DATE"="", "shot order"=1, "SHOT STATUS"=1, "Shot Angle"=0, "Corrected Impact"=0.0, "Corrected residual"=0.0, "Projectile Mass"=0.0, "usedv50"=FALSE, "Energy Loss (J)"=0.0, "BackFace\nDepth"=0.0, "BackFace\nDiameter"=0.0, "Redundant_Velocity"=0.0, "velLoss_PB"=0.0, "strikeVel_PB"=0.0, "UncorrectedRed_PB"=0.0, "CorrectedRed_PB"=0.0, "UncorrectedAvgVel_PB"=0.0, "V50userExcl"=FALSE, "Frag Rod"=0.0}]  # shotsArr
  w27 = errorcluster {"status"=FALSE, "code"=0, "source"=""}  # error in
  n1 = property on="RESET All" class="Bool (strict)"("Value"=TRUE ("RESET")) -> (error out=w5:errorcluster)  [unwired: 2 in, 1 out]
  n2 = Initialize Array(0.0, 2 ("dimension size")) -> (w6:dbl[])
  n3 = Obtain Queue(element data type=w6, error in (no error)=w5) -> (queue out=w3:refnum<queue>, error out=w21:errorcluster)  [unwired: 3 in, 1 out]
  n4 = call "Config Counter to Measure Two Edge Separation.vi"("errIN"=w5, "SampClk.Timebase.Src"="SampClk.Timebase.Src", "Counter"="ctr0") -> ("errOUT"=w10:errorcluster, "task out"=w2:refnum<k21>)  [unwired: 7 in]
  "taskCtr0" <- w2
  n5 = call "Config Counter to Measure Two Edge Separation.vi"("errIN"=w5, "SampClk.Timebase.Src"="SampClk.Timebase.Src", "Counter"="ctr1") -> ("errOUT"=w9:errorcluster, "task out"=w1:refnum<k21>)  [unwired: 7 in]
  "taskCtr1" <- w1
  n6 = call <vilib>:"Simple Error Handler.vi"("error in (no error)"=w5) -> ("error out"=w22:errorcluster)  [unwired: 4 in, 4 out]
  n7 = while "U/I Event Handler" {
    shift-right: [w31] -> _
    shift-left: w27 -> [w32]
    stop <- FALSE stop-if-true
    n8 = event shown="[12] \"Sort by AVG\", \"shotsArr\": Value Change" {
      selector: _ -> [_ _ _ _ _ _ _ _ _ _ _ _ _ _ _ _ _ _ _ _ _ _ _ _ _ _ _]
      dyn-events: _ -> [_ _ _ _ _ _ _ _ _ _ _ _ _ _ _ _ _ _ _ _ _ _ _ _ _ _ _]
      timeout: 100 -> [_ _ _ _ _ _ _ _ _ _ _ _ _ _ _ _ _ _ _ _ _ _ _ _ _ _ _]
      tunnel: w32 -> [w35 w38 w67 w77 w85 w87 w124 w148 w154 w180 w217 w259 w297 w299 w335 w371 w374 w383 w410 w412 w421 w447 w464 w466 w508 w539 _]
      tunnel: [w35 w40 w67 w74 w85 w86 w123 w147 w152 w188 w216 w256 w297 w299 w335 w371 w373 w379 w410 w412 w418 w444 w464 w466 w510 w539 w546] -> w31
      event Timeout {
        n9 = event-data() -> ()  [unwired: 2 out]
        n10 = Get Date/Time In Seconds() -> (seconds since 1Jan1904=w37:timestamp)
        n11 = Format Date/Time String(seconds (now)=w37) -> (date/time string=→"TimeNow":string)  [unwired: 2 out]
      }
      event "EXIT": Value Change {
        n12 = event-data() -> ()  [unwired: 2 out]
        n13 = Two Button Dialog(message="Exit BIMS Collector?\nAll Unsaved data will be lost.", 1:"NO" ("F button name (\"Cancel\")"), 2:"YES" ("T button name (\"OK\")")) -> (T button?=w39:bool)
        n14 = case shown="True" w39 {
          selector: w39 -> [_ w48]
          tunnel: [w44 w49] -> w40
          tunnel: w38 -> [w44 w45]
          frame False {
          }
          frame True {
            n15 = flat-sequence {
              tunnel: w48 -> [w55]
              tunnel: [w55] -> w46
              tunnel: w45 -> [w52]
              tunnel: [w57] -> w47
              tunnel: w46 -> [w57]
              tunnel: [w59] -> w49
              tunnel: w47 -> [w58]
              frame #0 {
                n16 = local read "taskCtr0"() -> (w53:refnum<k21>)
                n17 = call <vilib>:"DAQmx Clear Task.vi"("task in"=w53, "error in"=w52) -> ("error out"=w51:errorcluster)  [unwired: 13 in]
                n18 = local read "taskCtr1"() -> (w54:refnum<k21>)
                n19 = call <vilib>:"DAQmx Clear Task.vi"("task in"=w54, "error in"=w51) -> ("error out"=w50:errorcluster)  [unwired: 13 in]
                n20 = call <vilib>:"Simple Error Handler.vi"("error in (no error)"=w50) -> ()  [unwired: 4 in, 5 out]
              }
              frame #1 {
                # "close arming loop 1st"
                n21 = local write "close arming loop"(w57) -> ()
                n22 = Wait (ms)(milliseconds to wait=u32 1000) -> ()  [unwired: 1 out]
              }
              frame #2 {
                n23 = property on="Property Node" class="Application"(error in=errorcluster {"status"=FALSE, "code"=0, "source"=""} ("error in (no error)")) -> (error out=w59:errorcluster, "Application:Kind"=w61:T17)  [unwired: 1 in, 1 out]
                n24 = case shown="\"Run Time System\"" w61 {
                  tunnel: w58 -> [w62 w63 w64]
                  frame Default {
                    n25 = Stop(stop? (T)=w62) -> ()
                  }
                  frame "Development System" {
                    n26 = Stop(stop? (T)=w63) -> ()
                  }
                  frame "Run Time System" {
                    n27 = Quit LabVIEW(quit? (T)=w64) -> ()
                  }
                }
              }
            }
          }
        }
      }
      event "diagPageVisible": Value Change {
        # "Toggles display of \"Internal Use\" tab for diagnostics purposes"
        # "Key navigation ONLY: Cntrl-Shift-F11"
        n28 = event-data() -> ("NewVal"=w70:bool)  [unwired: 1 out]
        n29 = property on="aboutTabCntrl" class="TabCtl (strict)"(error in=errorcluster {"status"=FALSE, "code"=0, "source"=""} ("error in (no error)")) -> (error out=w69:errorcluster, "Pages"=w73:refnum<vi>[])  [unwired: 1 in, 1 out]
        n30 = Index Array(array=w73, index=1) -> (element=w71:refnum<vi>)
        n31 = property on="Property Node" class="Page"(reference=w71, error in=w69, "PageVis"=w70) -> (error out=w68:errorcluster)  [unwired: 1 out]
        n32 = property on="diagPageVisible" class="Bool (strict)"(error in=w68, "Value"=w70) -> (error out=w65:errorcluster)  [unwired: 1 in, 1 out]
        n33 = call <vilib>:"General Error Handler.vi"("error in (no error)"=w65) -> ()  [unwired: 2 in, 13 out]
      }
      event "runtimeMenusVisible": Value Change {
        # "Key navigation ONLY: Cntrl-Shift-F10"
        n34 = event-data() -> ("NewVal"=w79:bool)  [unwired: 1 out]
        n35 = control-ref of="This VI"() -> (w78:refnum<vi>)
        n36 = property class="VI"(reference=w78, error in=w77, "Front Panel.ShowMenuBar"=w79) -> (reference out=w76:refnum<vi>, error out=w75:errorcluster)
        n37 = Close Reference(reference=w76, error in (no error)=w75) -> (error out=w74:errorcluster)
      }
      event "MeasVelScrnSet1", "MeasVelScrnSet2": Value Change {
        n38 = event-data() -> ()  [unwired: 2 out]
        n39 = local read "MeasVelScrnSet1"() -> (w84:sgl)
        n40 = local read "MeasVelScrnSet2"() -> (w83:sgl)
        n41 = Add(x=w84, y=w83) -> (x+y=w82:sgl)
        n42 = Divide(x=w82, y=sgl 2.0) -> (x/y=w80:sgl)
        n43 = local write "Current/avg/speed"(w80) -> ()
      }
      event "QueryLoad": Value Change {
        w92 = "%x" ("time format string (%c)")
        w108 = "" ("replace string (\"\")")
        # "This section plots  Impact velocity vs. loadingdata"
        n44 = event-data() -> ()  [unwired: 2 out]
        n45 = Format Date/Time String(time format string (%c)=w92, seconds (now)="lkupStartDate") -> (date/time string=w91:string)  [unwired: 1 out]
        n46 = Format Date/Time String(time format string (%c)=w92, seconds (now)="lkupEndDate") -> (date/time string=w90:string)  [unwired: 1 out]
        n47 = call "Trim String.vi"("inStr"="Powder.freeTxt") -> ("outStr"=w106:string)
        n48 = call "Trim String.vi"("inStr"="Threat.freeTxt") -> ("outStr"=w107:string)
        n49 = invoke on="v50_table" class="Tbl" method="Reinit To Default"(error in=w87) -> (error out=w99:errorcluster)  [unwired: 2 in, 2 out]
        n50 = invoke on="Vel.vs.Loading" class="WFGraph (strict)" method="Reinit To Default"(error in=w99) -> (error out=w94:errorcluster)  [unwired: 2 in, 2 out]
        n51 = Format Into String(format string="SELECT TOP %d dbsrc.experiment.threat, dbsrc.shots.loading, dbsrc.shots.impact, dbsrc.experiment.powder, dbsrc.shots.date from dbsrc.shots, dbsrc.experiment where dbsrc.shots.expt = dbsrc.experiment.expt and dbsrc.shots.loading > 0 and dbsrc.shots.date between '%s' and '%s' and dbsrc.shots.impact between 10 and 5000 and dbsrc.experiment.powder like '%%%s%%' and dbsrc.experiment.threat like '%%%s%%' and experiment.threat<>'' order by dbsrc.experiment.threat, dbsrc.shots.loading, dbsrc.shots.impact;" ("Format String"), error in=w94, "maxRecs", w91, w90, w106, w107) -> (resulting string=w112:string, error out=w97:errorcluster)  [unwired: 1 in]
        n52 = Search and Replace String(input string=w112, search string=" and experiment.powder like '%%'", replace string=w108, error in=w97) -> (result string=w110:string, error out=w98:errorcluster)  [unwired: 6 out]
        n53 = Search and Replace String(input string=w110, search string="and experiment.threat like '%%'", replace string=w108, error in=w98) -> (result string=w101:string, error out=w96:errorcluster)  [unwired: 6 out]
        n54 = call "Fetch Data (SubVI).vi"("error IN"=w96, "query string"=w101) -> ("error OUT"=w86:errorcluster, "recordset data"=w102:string[][])  [unwired: 4 out]
        "v50_table" <- w102
        n55 = Fract/Exp String To Number(string=w102) -> (number=w116:dbl[][])  [unwired: 4 out]
        n56 = Array Size(array=w102) -> (size(s)=w104:i32[])
        n57 = Index Array(array=w104) -> (element=→"ActualNumRecs":i32)  [unwired: 1 in]
        n58 = Index Array(array=w116, index (col)=2 ("Disabled Index (col)")) -> (element=w115:dbl[])  [unwired: 1 in]
        n59 = Index Array(array=w116, index (col)=1 ("Disabled Index (col)")) -> (element=w114:dbl[])  [unwired: 1 in]
        n60 = Bundle(w114, w115) -> (→"Vel.vs.Loading":cluster{dbl[], dbl[]})  [unwired: 1 out]
      }
      event "ThreatGroups": Value Change {
        n61 = event-data() -> ()  [unwired: 2 out]
        n62 = control-ref of="ThreatGroups"() -> (w125:refnum<vi>)
        n63 = property on="Property Node" class="Ring (strict)"(reference=w125, error in=w124) -> (error out=w122:errorcluster, "RingText.Text"=w120:string)  [unwired: 1 out]
        n64 = Not Equal?(x=w120, y="") -> (x != y?=w119:bool)
        n65 = case shown="True" w119 {
          tunnel: w120 -> [_ w134]
          tunnel: [w126 w132] -> w123
          tunnel: w122 -> [w129 w131]
          frame False {
            n66 = property on="ThreatDetails" class="Ring (strict)"(error in=w129, "Strings []"=string[] [], "Value"=u16 0 ("Value (Signaling)")) -> (error out=w127:errorcluster)  [unwired: 1 in, 1 out]
            n67 = invoke on="threatDetails" class="Clust (strict)" method="Reinit To Default"(error in=w127) -> (error out=w126:errorcluster)  [unwired: 2 in, 2 out]
          }
          frame True {
            n68 = call "Select Threat Details.vi"("threatGroup"=w134) -> ("threatDetails"=w133:string[])  [unwired: 1 out]
            n69 = property on="ThreatDetails" class="Ring (strict)"(error in=w131, "Strings []"=w133, "Val(Sgnl)"=u16 0 ("Value (Signaling)")) -> (error out=w132:errorcluster)  [unwired: 1 in, 1 out]
          }
        }
      }
      event "panelSearch": Value Change {
        # "This section returns past panels"
        n70 = event-data() -> ()  [unwired: 2 out]
        n71 = control-ref of="pastPanels"() -> (w150:refnum<vi>)
        n72 = control-ref of="Mfr_0"() -> (w145:refnum<vi>)
        n73 = control-ref of="SampleStyle_0"() -> (w146:refnum<vi>)
        n74 = control-ref of="Requestors_0"() -> (w144:refnum<vi>)
        n75 = control-ref of="ThreatSize_0"() -> (w143:refnum<vi>)
        n76 = call "queryPanels (SubVI).vi"("ThreatSize_0"=w143, "Mfr_0"=w145, "Requestors_0"=w144, "Style_0"=w146, "error in"=w148, "srchParams"="srchParams", "pastPanels"=w150) -> ("error out"=w147:errorcluster, "recordset data"=w142:string[][], "actualNumPanels"=→"actualNumPanels":i32)  [unwired: 2 in]
        "pastPanels" <- w142
        n77 = Index Array(array=w142) -> (element=w136:string[])  [unwired: 2 in]
        n78 = Array Size(array=w136) -> (size(s)=w141:i32)
        n79 = Greater Than 0?(x=w141) -> (x > 0?=w140:bool)
        n80 = Select(t=T15."Enabled" ("Disabled"), s=w140, f=T15."Disabled and Grayed Out" ("Disabled")) -> (s? t:f=w139:T15)
        n81 = property on="reportV50_History" class="Bool"("DisabledEnum"=w139) -> ()  [unwired: 2 in, 2 out]
      }
      event "pastPanels": Mouse Up {
        n82 = event-data() -> ("CtlRef"=w162:refnum<vi>)  [unwired: 1 out]
        n83 = property on="Property Node" class="Tbl (strict)"(reference=w162, error in=w154) -> (error out=w153:errorcluster, "Value"=w161:string[][], "EditPos"=w160:T18)  [unwired: 1 out]
        n84 = Unbundle By Name(w160) -> ("Row"=w159:i32)
        n85 = Index Array(array=w161, index (row)=w159, index (col)=0 ("disabled index (col)")) -> (element=w158:string)
        n86 = Scan From String(input string=w158, error in=w153, default 1=1 ("Record #")) -> (error out=w152:errorcluster, output 1=w156:i32)  [unwired: 2 in, 2 out]
        n87 = local write "Record #"(w156) -> ()
      }
      event "ThreatDetails", "SampleID": Value Change {
        # "A Sample ID is entered"
        # "A range is selected"
        # "A measurement requires the selection of a threat,\nso delay enabling the \"Measure\" tab until a grain wt\nis chosen."
        n88 = event-data() -> ()  [unwired: 2 out]
        n89 = control-ref of="ThreatGroups"() -> (w181:refnum<vi>)
        n90 = control-ref of="ThreatDetails"() -> (w178:refnum<vi>)
        n91 = call "Get Projectile Atributes from ThreatGroupDetail.vi"("error IN"=w180, "ThreatDetail"=w178, "ThreatGroup"=w181) -> ("error out"=w179:errorcluster, "projectileAttribs"=w177:T19)  [unwired: 1 out]
        "threatDetails" <- w177
        n92 = Unbundle By Name(w177) -> ("grainSize"=w170:string)
        n93 = Equal?(x=w170, y="") -> (x = y?=w171:bool)
        n94 = case shown="False" w171 {
          tunnel: w170 -> [w198 _]
          tunnel: [w197 u16 0 ("GrainSize")] -> w176
          frame False {
            # "A grain size is selected"
            n95 = Scan From String(input string=w198) -> (output 1=w197:u16)  [unwired: 3 in, 4 out]
            "GrainSize" <- w197
          }
          frame True {
            # "A grain size not selected"
          }
        }
        n96 = Equal?(x=w170, y="") -> (x = y?=w195:bool)
        n97 = local read "rangeSetup"() -> (w192:u16)
        n98 = case shown="False" w195 {
          tunnel: [w202 sgl 0.0] -> w191
          tunnel: w170 -> [w200 _]
          frame False {
            w204 = sgl 0.0  # sgl
            n99 = Scan From String(format string="%f " ("Format String"), input string=w200, default 1=w204) -> (output 1=w203:sgl)  [unwired: 2 in, 3 out]
            n100 = disable-structure shown="Enabled" {
              disable-tunnel: w203 -> [w207 w208]
              disable-tunnel: [w206 w208] -> w202
              frame Disabled {
                n101 = Multiply(x=sgl 0.06479891, y=w207) -> (x*y=w206:sgl)
              }
              frame Enabled {
              }
            }
          }
          frame True {
          }
        }
        "Projectile Mass" <- w191
        n102 = local read "SampleID"() -> (w175:string)
        n103 = Greater Than 0?(x=w192) -> (x > 0?=w193:bool)
        n104 = Greater Than 0?(x=w176) -> (x > 0?=w194:bool)
        n105 = Not Equal?(x=w175, y="") -> (x != y?=w173:bool)
        n106 = Compound Arithmetic op=AND(w194, w193, w173) -> (w168:bool)
        n107 = property on="mainTabCntrl" class="TabCtl (strict)"(error in=w179) -> (error out=w184:errorcluster, "Pages"=w187:refnum<vi>[])  [unwired: 1 in, 1 out]
        n108 = Not(x=w168) -> (.not. x?=w183:bool)
        n109 = Index Array(array=w187, index=1) -> (element=w185:refnum<vi>)
        n110 = Select(t=T16."Page Enabled" ("Page Enabled State"), s=w168, f=T16."Page Disabled & Grayed" ("Page Enabled State")) -> (s? t:f=w167:T16)
        n111 = property on="Property Node" class="Page"(reference=w185, error in=w184, "PageEnb"=w167) -> (error out=w182:errorcluster)  [unwired: 1 out]
        n112 = Select(t=T15."Enabled" ("Disabled"), s=w168, f=T15."Disabled and Grayed Out" ("Disabled")) -> (s? t:f=w165:T15)
        n113 = property on="ARM" class="Bool"(error in=w182, "Disabled"=w165) -> (error out=w190:errorcluster)  [unwired: 1 in, 1 out]
        n114 = property on="addShot" class="Bool"(error in=w190, "Disabled"=w165) -> (error out=w189:errorcluster)  [unwired: 1 in, 1 out]
        n115 = property on="instruct_addShot" class="Str"(error in=w189, "Visible"=w183) -> (error out=w188:errorcluster)  [unwired: 1 in, 1 out]
      }
      event "Mfr_1", "Mfr_2", "Mfr_3", "Mfr_4", "Mfr_5", "Mfr_6", "Mfr_0": Value Change {
        n116 = event-data() -> ("CtlRef"=w225:refnum<vi>)  [unwired: 1 out]
        n117 = property on="Property Node" class="Ring (strict)"(reference=w225, error in=w217) -> (error out=w215:errorcluster, "Label.Text"=w221:string, "RingText.Text"=w222:string)  [unwired: 1 out]
        n118 = flat-sequence {
          tunnel: ["Mfr_1"] -> _
          tunnel: ["Mfr_2"] -> _
          tunnel: ["Mfr_3"] -> _
          tunnel: ["Mfr_4"] -> _
          tunnel: ["Mfr_5"] -> _
          tunnel: ["Mfr_6"] -> _
          frame #0 {
          }
        }
        n119 = call "Select Sample Style.vi"("error IN"=w215, "Mfr"=w222) -> ("error Out"=w214:errorcluster, "SampleStyles"=w211:string[])  [unwired: 4 out]
        n120 = Scan From String(format string="Mfr_%d", input string=w221, error in=w214, default 1=0 ("Mfr#")) -> (error out=w212:errorcluster, output 1=w220:i32)  [unwired: 1 in, 2 out]
        n121 = case shown="1" w220 {
          tunnel: [w237 w240 w243 w246 w249 w252 w255] -> w219
          tunnel: [w236 w239 w242 w245 w248 w251 w254] -> w213
          tunnel: w212 -> [w236 w239 w242 w245 w248 w251 w254]
          tunnel: w211 -> [w235 w238 w241 w244 w247 w250 w253]
          tunnel: [w234 w238 w241 w244 w247 w250 w253] -> w210
          frame 0, Default {
            n122 = Delete From Array(array=w235, length=1, index=0) -> (array with subset deleted=w234:string[])  [unwired: 1 out]
            n123 = control-ref of="SampleStyle_0"() -> (w237:refnum<vi>)
          }
          frame 1 {
            n124 = control-ref of="SampleStyle_1"() -> (w240:refnum<vi>)
          }
          frame 2 {
            n125 = control-ref of="SampleStyle_2"() -> (w243:refnum<vi>)
          }
          frame 3 {
            n126 = control-ref of="SampleStyle_3"() -> (w246:refnum<vi>)
          }
          frame 4 {
            n127 = control-ref of="SampleStyle_4"() -> (w249:refnum<vi>)
          }
          frame 5 {
            n128 = control-ref of="SampleStyle_5"() -> (w252:refnum<vi>)
          }
          frame 6 {
            n129 = control-ref of="SampleStyle_6"() -> (w255:refnum<vi>)
          }
        }
        n130 = property on="Property Node" class="Ring (strict)"(reference=w219, error in=w213, "Strings []"=w210, "Val(Sgnl)"=u16 0 ("Value (Signaling)")) -> (error out=w216:errorcluster)  [unwired: 1 out]
      }
      event "SampleStyle_1", "SampleStyle_2", "SampleStyle_3", "SampleStyle_4", "SampleStyle_5", "SampleStyle_6", "SampleStyle_0": Value Change {
        n131 = event-data() -> ("CtlRef"=w265:refnum<vi>)  [unwired: 1 out]
        n132 = call "Get Sample Style Atributes.vi"("StyleNumRef"=w265) -> ("SampleSpecs"=w260:T20)  [unwired: 1 in]
        n133 = flat-sequence {
          tunnel: ["SampleStyle_1"] -> _
          tunnel: ["SampleStyle_2"] -> _
          tunnel: ["SampleStyle_3"] -> _
          tunnel: ["SampleStyle_4"] -> _
          tunnel: ["SampleStyle_5"] -> _
          tunnel: ["SampleStyle_6"] -> _
          frame #0 {
          }
        }
        n134 = property on="Property Node" class="Ring (strict)"(reference=w265, error in=w259) -> (error out=w258:errorcluster, "Label.Text"=w264:string)  [unwired: 1 out]
        n135 = Scan From String(format string="SampleStyle_%d", input string=w264, error in=w258, default 1=0 ("default value 1")) -> (error out=w257:errorcluster, output 1=w262:i32)  [unwired: 1 in, 2 out]
        n136 = case shown="1" w262 {
          tunnel: w260 -> [w274 w277 w280 w283 w286 w289 w292]
          tunnel: w257 -> [w273 w276 w279 w282 w285 w288 w291]
          tunnel: [w272 w275 w278 w281 w284 w287 w290] -> w256
          frame 0, Default {
            n137 = property on="SampleAttribs_0" class="Clust (strict)"(error in=w273, "Val(Sgnl)"=w274) -> (error out=w272:errorcluster)  [unwired: 1 in, 1 out]
            "SampleAttribs_0" <- w274
          }
          frame 1 {
            n138 = property on="SampleAttribs_1" class="Clust (strict)"(error in=w276, "Val(Sgnl)"=w277) -> (error out=w275:errorcluster)  [unwired: 1 in, 1 out]
            "SampleAttribs_1" <- w277
          }
          frame 2 {
            n139 = property on="SampleAttribs_2" class="Clust (strict)"(error in=w279, "Val(Sgnl)"=w280) -> (error out=w278:errorcluster)  [unwired: 1 in, 1 out]
            "SampleAttribs_2" <- w280
          }
          frame 3 {
            n140 = property on="SampleAttribs_3" class="Clust (strict)"(error in=w282, "Val(Sgnl)"=w283) -> (error out=w281:errorcluster)  [unwired: 1 in, 1 out]
            "SampleAttribs_3" <- w283
          }
          frame 4 {
            n141 = property on="SampleAttribs_4" class="Clust (strict)"(error in=w285, "Val(Sgnl)"=w286) -> (error out=w284:errorcluster)  [unwired: 1 in, 1 out]
            "SampleAttribs_4" <- w286
          }
          frame 5 {
            n142 = property on="SampleAttribs_5" class="Clust (strict)"(error in=w288, "Val(Sgnl)"=w289) -> (error out=w287:errorcluster)  [unwired: 1 in, 1 out]
            "SampleAttribs_5" <- w289
          }
          frame 6 {
            n143 = property on="SampleAttribs_6" class="Clust (strict)"(error in=w291, "Val(Sgnl)"=w292) -> (error out=w290:errorcluster)  [unwired: 1 in, 1 out]
            "SampleAttribs_6" <- w292
          }
        }
      }
      event "Sort by AVG": Value Change {
        n144 = event-data() -> ()  [unwired: 2 out]
        n145 = local read "shotsArr"() -> (w295:T6)
        n146 = local read "Site"() -> (w293:string)
        n147 = call "Update Shot Table.vi"("Sort by AVG"="Sort by AVG", "Site"=w293, "shotsArr"=w295) -> ("shotTable OUT"=→"Table of Shots":string[][])
      }
      event "Layer_1", "Layer_2", "Layer_3", "Layer_4", "Layer_5", "Layer_6", "SampleAttribs_1.ozPerYd2", "SampleAttribs_2.ozPerYd2", "SampleAttribs_3.ozPerYd2", "SampleAttribs_4.ozPerYd2", "SampleAttribs_5.ozPerYd2", "SampleAttribs_6.ozPerYd2": Value Change {
        n148 = event-data() -> ()  [unwired: 2 out]
        n149 = global read "BIMS_Collector Globals.vi" "SampleAttribs"() -> (w298:T21)
        n150 = Build Array("Layer_1", "Layer_2", "Layer_3", "Layer_4", "Layer_5", "Layer_6") -> (w300:T22)
        n151 = global write "BIMS_Collector Globals.vi" "LayerSpecs"(w300) -> ()
        n152 = for {
          tunnel: w300 -> [w327] mode=indexing
          shift-right: [w329] -> w308
          shift-left: 0 -> [w328]
          tunnel: [w326] -> w318 mode=indexing
          tunnel: w298 -> [w324] mode=indexing
          n153 = Unbundle By Name(w324) -> ("ozPerYd2"=w320:string)
          n154 = Equal?(x=w320, y="" ("Empty String Constant")) -> (x = y?=w319:bool)
          n155 = case shown="False" w319 {
            tunnel: [w333 sgl 0.0 ("default value 1")] -> w323
            tunnel: w320 -> [w330 _]
            frame False {
              n156 = Scan From String(format string="%f", input string=w330, default 1=sgl 0.0 ("default value 1")) -> (output 1=w333:sgl)  [unwired: 2 in, 3 out]
            }
            frame True {
            }
          }
          n157 = Unbundle By Name(w327) -> ("plyNum"=w325:i32)
          n158 = Add(x=w328, y=w325) -> (x+y=w329:i32)
          n159 = To Single Precision Float(number=w325) -> (single precision float=w322:sgl)
          n160 = Multiply(x=w322, y=w323) -> (x*y=w326:sgl)
        }
        "totalNumLayers" <- w308
        n161 = Divide(x=w318, y=sgl 144.0) -> (x/y=w316:sgl[])
        n162 = Index Array(array=w316) -> (element #1=→"fab1_totalWt":sgl, element #2=→"fab2_totalWt":sgl, element #3=→"fab3_totalWt":sgl, element #4=→"fab4_totalWt":sgl, element #5=→"fab5_totalWt":sgl, element #6=→"fab6_totalWt":sgl)  [unwired: 6 in]
        n163 = Add Array Elements(numeric array=w316) -> (sum=→"totalBAW":sgl)
      }
      event "clayCalArray": Value Change {
        n164 = event-data() -> ()  [unwired: 2 out]
        n165 = for {
          tunnel: "clayCalArray" -> [w361] mode=indexing
          shift-right: [w360] -> w343
          shift-left: "" ("Empty String Constant") -> [w358]
          shift-right: [w355] -> w339
          shift-left: i16[] [] -> [w354]
          n166 = Greater Than 0?(x=w361) -> (x > 0?=w362:bool)
          n167 = case shown="False" w362 {
            tunnel: w361 -> [_ w368]
            tunnel: ["##" ("clayCalib") w370] -> w359
            tunnel: w358 -> [w365 w369]
            tunnel: [w365 w369] -> w357
            tunnel: [w363 w367] -> w355
            tunnel: w354 -> [w363 w366]
            frame False {
            }
            frame True {
              n168 = Format Into String(w368) -> (resulting string=w370:string)  [unwired: 3 in, 1 out]
              n169 = Build Array (concatenate)(w366, w368) -> (w367:i16[])
            }
          }
          n170 = Concatenate Strings(w357, w359, "-" ("string")) -> (w360:string)
        }
        n171 = String Length(string=w343) -> (length=w344:i32)
        n172 = Add Array Elements(numeric array=w339) -> (sum=w348:i16)
        n173 = Array Size(array=w339) -> (size(s)=w349:i32)
        n174 = Decrement(x=w344) -> (x-1=w341:i32)
        n175 = To Single Precision Float(number=w348) -> (single precision float=w347:sgl)
        n176 = To Single Precision Float(number=w349) -> (single precision float=w337:sgl)
        n177 = String Subset(string=w343, length (rest)=w341) -> (substring=w342:string)  [unwired: 1 out]
        n178 = Equal To 0?(x=w337) -> (x = 0?=w336:bool)
        n179 = local write "clayCalib"(w342) -> ()
        n180 = case shown="True" w336 {
          tunnel: w347 -> [w352 w353]
          tunnel: w337 -> [w351 _]
          tunnel: [w350 w353] -> w346
          frame False {
            n181 = Divide(x=w352, y=w351) -> (x/y=w350:sgl)
          }
          frame True {
          }
        }
        "clayAverage" <- w346
      }
      event "reportV50_History": Value Change {
        n182 = event-data() -> ()  [unwired: 2 out]
        n183 = local write "lookupRec"(TRUE ("lookupRec")) -> ()
      }
      event "Methods": Value Change {
        n184 = event-data() -> ("CtlRef"=w378:refnum<vi>)  [unwired: 1 out]
        n185 = call "Dropdown Selection (SubVI).vi"("reference"=w378) -> ("element"=w377:string)
        n186 = Equal?(x=w377, y="V50") -> (x = y?=w375:bool)
        n187 = property on="minV50" class="DigNum (strict)"(error in=w374, "Visible"=w375) -> (error out=w373:errorcluster)  [unwired: 1 in, 1 out]
      }
      event "rangeSetup": Value Change {
        n188 = event-data() -> ("NewVal"=w387:u16)  [unwired: 1 out]
        n189 = case shown="2" w387 {
          tunnel: ["0" ("section") "5.0" ("section") "7.5" ("section") "45.0" ("section")] -> w393
          frame 0, Default {
          }
          frame 1 {
          }
          frame 2 {
          }
          frame 3 {
          }
        }
        n190 = local read "configPath"() -> (w395:path)
        n191 = local read "GrainSize"() -> (w386:u16)
        n192 = Greater Than 0?(x=w387) -> (x > 0?=w390:bool)
        n193 = Greater Than 0?(x=w386) -> (x > 0?=w388:bool)
        n194 = call <vilib>:"Open Config Data (compatibility).vi"("error in (no error)"=w383, "configuration file path"=w395) -> ("error out"=w403:errorcluster, "refnum"=w405:T23)  [unwired: 7 in, 1 out]
        n195 = And(x=w390, y=w388) -> (x .and. y?=w389:bool)
        n196 = call-poly <vilib>:"Write Key.vi"("write raw string? (F)"=TRUE, "section"="Ballistic Parameters", "error in (no error)"=w403, "value"=w393, "key"="MidPoint To Target Distance", "refnum"=w405) -> ("error out"=w402:errorcluster, "refnum out"=w401:T23)  [unwired: 4 out]
        n197 = call <vilib>:"Close Config Data.vi"("error in (no error)"=w402, "refnum"=w401) -> ("error out"=w394:errorcluster)  [unwired: 1 in, 8 out]
        n198 = Not(x=w389) -> (.not. x?=w399:bool)
        n199 = Select(t=u8 0 ("y"), s=w389, f=u8 2 ("y")) -> (s? t:f=w385:u8)
        n200 = Scan From String(input string=w393, error in=w394, default 1=sgl 0.0 ("default value 1")) -> (error out=w382:errorcluster, output 1=w392:sgl)  [unwired: 2 in, 2 out]
        n201 = local write "mid_to_targ_dist"(w392) -> ()
        n202 = property on="ARM" class="Bool"(error in=w382, "Disabled"=w385) -> (error out=w381:errorcluster)  [unwired: 1 in, 1 out]
        n203 = property on="addShot" class="Bool"(error in=w381, "Disabled"=w385) -> (error out=w380:errorcluster)  [unwired: 1 in, 1 out]
        n204 = property on="instruct_addShot" class="Str"(error in=w380, "Visible"=w399) -> (error out=w379:errorcluster)  [unwired: 1 in, 1 out]
        "instruct_addShot" <- "RANGE SETUP and THREAT must be selected before shots can be added." ("instruct_addShot")
      }
      event "Drag Corrected", "maxDev": Value Change {
        n205 = event-data() -> ()  [unwired: 2 out]
        n206 = local write "processShots"(TRUE ("ProcessShots")) -> ()
      }
      event "2ndScreen": Value Change {
        n207 = event-data() -> ()  [unwired: 7 out]
        n208 = Select(t=T15."Enabled" ("Disabled"), s="2ndScreen", f=T15."Disabled and Grayed Out" ("Disabled")) -> (s? t:f=w413:T15)
        n209 = property on="Redundant/speed" class="DigNum (strict)"("DisabledEnum"=w413) -> ()  [unwired: 2 in, 2 out]
        n210 = property on="MeasVelScrnSet2" class="DigNum (strict)"("DisabledEnum"=w413) -> ()  [unwired: 2 in, 2 out]
      }
      event "MC Listbox of Shots": Mouse Up {
        n211 = event-data() -> ()  [unwired: 2 out]
        n212 = flat-sequence {
          tunnel: w421 -> [w425]
          tunnel: [w423] -> w420
          tunnel: ["MC Listbox of Shots"] -> w417
          tunnel: w420 -> [w429]
          tunnel: [w428] -> w419
          tunnel: w417 -> [_]
          tunnel: w419 -> [w434]
          tunnel: [w432] -> w418
          frame #0 {
            n213 = property on="Table of Shots" class="Tbl (strict)"(error in=w425) -> (error out=w424:errorcluster, "Value"=w426:string[][])  [unwired: 1 in, 1 out]
            n214 = local write "STOP (Shots MC LB)"(FALSE ("STOP (Shots MC LB)")) -> ()
            n215 = property on="MC Listbox of Shots" class="MCListbox (strict)"(error in=w424, "ItemNames"=w426) -> (error out=w423:errorcluster)  [unwired: 1 in, 1 out]
          }
          frame #1 {
            n216 = control-ref of="MC Listbox of Shots"() -> (w431:refnum<vi>)
            n217 = control-ref of="STOP (Shots MC LB)"() -> (w430:refnum<vi>)
            n218 = call "multicolumn listbox sort.vi"("error IN"=w429, "Bool Refnum"=w430, "MCListbox Refnum"=w431) -> ("error out"=w428:errorcluster)  [unwired: 4 in]
          }
          frame #2 {
            n219 = property on="MC Listbox of Shots" class="MCListbox (strict)"(error in=w434) -> (error out=w433:errorcluster, "ItemNames"=w435:string[][])  [unwired: 1 in, 1 out]
            n220 = property on="Table of Shots" class="Tbl (strict)"(error in=w433, "Val(Sgnl)"=w435) -> (error out=w432:errorcluster)  [unwired: 1 in, 1 out]
          }
        }
      }
      event "PublishNewRecords": Value Change {
        w441 = "\\" ("string")
        w451 = TRUE  # overwrite (F)
        # "2. INSERT new records to Experiments and  \n      Shots tables in local Export.mdb file."
        # "1. SELECT new records from local MDB \n     by comparing against last record numbers \n     found in IMPORT table on BIMS server."
        # "Pushes latest ballistics performance data up to BIMS Server\n\n - Attempts connection with server (reports connection success in msgbox)\n - If successful:\n   - Exports all experiment/shot records since last table marker to [site].mdb file\n   - Sends export.mdb file to drop location on BIMS File Server\n   - Executes SSIS package to import records from export.mdb file\n - Otherwise provides option to try again or cancel"
        # "3. Copy Export.mdb file to [sitename].mdb in [sitename] \n      FileDrop folder on BIMS server."
        n221 = event-data() -> ()  [unwired: 2 out]
        n222 = property on="Loading" class="Ring (strict)"(error in=w447, "Visible"=TRUE) -> (error out=w446:errorcluster)  [unwired: 1 in, 1 out]
        n223 = local read "Site"() -> (w436:string)
        n224 = call "Export New Records.vi"("error IN"=w446, "Site"=w436) -> ("error out"=w453:errorcluster)  [unwired: 3 in, 6 out]
        n225 = Concatenate Strings("\\\\" ("string"), "Server", w441, "Folder", w441, w436, ".mdb" ("string")) -> (w437:string)
        n226 = String To Path(string=w437) -> (path=w449:path)
        n227 = Copy(8:w453, 9:w451, 10:w449, 11:path "C:/Ballistics/Export.mdb" ("source path")) -> (0:w450:errorcluster)  [unwired: 3 out]
        n228 = case shown="No Error" w450 {
          selector: w450 -> [w455 w457]
          tunnel: [w455 w456] -> w445
          frame No Error {
            n229 = One Button Dialog(message="New sample performance records submitted \nto BIMS Warehouse successfully.\n\nPublishing will occur in under five minutes.") -> ()  [unwired: 2 out]
          }
          frame Error {
            n230 = call <vilib>:"General Error Handler.vi"("error in (no error)"=w457) -> ("error out"=w456:errorcluster)  [unwired: 2 in, 12 out]
          }
        }
        n231 = property on="Loading" class="Ring (strict)"(error in=w445, "Visible"=FALSE) -> (error out=w444:errorcluster)  [unwired: 1 in, 1 out]
      }
      event "arrIDC": Mouse Up {
        n232 = event-data() -> ()  [unwired: 2 out]
        "velProfile" <- cluster{dbl, dbl}[] [] ("velProfile")
        "arrIDC" <- dbl[] [] ("arrIDC")
        "relativeTime" <- cluster{"ts2":dbl, "ts3":dbl, "ts1":dbl} {"ts2"=0.0, "ts3"=0.0, "ts1"=0.0} ("relativeTime")
        "velMeasProf" <- T8 {"v2"=0.0, "vB"=0.0, "vOuter"=0.0, "v1"=0.0, "vA"=0.0, "vInner"=0.0} ("velMeasProf")
        "velCompProf" <- cluster{"vStrike":dbl, "vA":dbl} {"vStrike"=0.0, "vA"=0.0} ("velCompProf")
        "displacement" <- T9 {"ds_v2"=6.75, "ds2"=5.0833, "ds_vB"=4.9167, "ds3"=4.75, "ds_vAvg"=6.9167, "ds_v1"=7.0833, "ds1"=8.75, "ds_vA"=8.9167, "ds0"=9.0833} ("displacement")
      }
      event "SampleBackings": Value Change {
        # "Clay is the default sample backing material.\n\n  If another selection is made, then grey out and disable all controls relating to clay."
        n233 = event-data() -> ()  [unwired: 2 out]
        n234 = case shown="2.." "SampleBackings" {
          tunnel: [T15."Disabled and Grayed Out" ("Disabled") T15."Enabled" ("Disabled") T15."Disabled and Grayed Out" ("Disabled")] -> w465
          frame 0, Default {
          }
          frame 1 {
          }
          frame 2.. {
          }
        }
        n235 = property on="clayCalArray" class="Arr (strict)"("DisabledEnum"=w465) -> ()  [unwired: 2 in, 2 out]
        n236 = property on="clayAverage" class="DigNum (strict)"("DisabledEnum"=w465) -> ()  [unwired: 2 in, 2 out]
        n237 = property on="clayTemp" class="DigNum (strict)"("DisabledEnum"=w465) -> ()  [unwired: 2 in, 2 out]
      }
      event "RefreshMetadata": Value Change {
        # "Pulls latest metadata down from BIMS Database Server\n - Attempts connection with server \n        (reports failure if connection is unsuccessful)\n - If successful:\n   - Updates local database records from server\n   - Updates dropdown listboxes from local database"
        n238 = event-data() -> ()  [unwired: 2 out]
        n239 = Initialize Array(T4 {"plyNum"=0, "LotNum"="-", "RollNum"="-"} ("Layer_1"), 6 ("dimension size")) -> (w480:T22)
        n240 = property on="Loading" class="Ring (strict)"(error in=w508, "Visible"=TRUE) -> (error out=w507:errorcluster)  [unwired: 1 in, 1 out]
        n241 = control-ref of="LayerStitchTypes"() -> (w493:refnum<vi>)
        n242 = control-ref of="BackLayer"() -> (w503:refnum<vi>)
        n243 = control-ref of="FrontLayer"() -> (w504:refnum<vi>)
        n244 = control-ref of="ThreatGroups"() -> (w505:refnum<vi>)
        n245 = control-ref of="SampleClamping"() -> (w512:refnum<vi>)
        n246 = control-ref of="SampleTypes"() -> (w529:refnum<vi>)
        n247 = control-ref of="SampleDimensions"() -> (w528:refnum<vi>)
        n248 = control-ref of="ModelMfrs"() -> (w527:refnum<vi>)
        n249 = control-ref of="Assemblers"() -> (w526:refnum<vi>)
        n250 = control-ref of="Submitters"() -> (w525:refnum<vi>)
        n251 = control-ref of="PowderTypes"() -> (w524:refnum<vi>)
        n252 = control-ref of="Methods"() -> (w521:refnum<vi>)
        n253 = control-ref of="TestConditions"() -> (w520:refnum<vi>)
        n254 = control-ref of="SampleBackings"() -> (w519:refnum<vi>)
        n255 = control-ref of="Ballisticians"() -> (w518:refnum<vi>)
        n256 = control-ref of="Shooters"() -> (w517:refnum<vi>)
        n257 = control-ref of="Recorders"() -> (w516:refnum<vi>)
        n258 = global write "BIMS_Collector Globals.vi" "LayerSpecs"(w480) -> ()
        n259 = control-ref of="SampleCoverings"() -> ()  [unwired: 1 out]
        n260 = Build Array(w493, w503, w504, w505, w512, w529, w528, w527, w526, w525, w524, w521, w520, w519, w518, w517, w516) -> (w523:refnum<vi>[])
        n261 = Index Array(array=w480) -> (element #1=w481:T4, element #2=w479:T4, element #3=w478:T4, element #4=w477:T4, element #5=w476:T4, element #6=w475:T4)  [unwired: 8 in, 2 out]
        n262 = control-ref of="loadStatus"() -> (w487:refnum<vi>)
        n263 = local write "Layer_1"(w481) -> ()
        n264 = local write "Layer_2"(w479) -> ()
        n265 = local write "Layer_3"(w478) -> ()
        n266 = local write "Layer_4"(w477) -> ()
        n267 = local write "Layer_5"(w476) -> ()
        n268 = local write "Layer_6"(w475) -> ()
        n269 = call "Update Metadata using listbox names.vi"("loadStatus Refnum"=w487, "error in"=w507, "Site"="Site", "RefNumArrIn"=w523) -> ("error out"=w485:errorcluster, "RefNumArrOut"=w522:refnum<vi>[])  [unwired: 6 out]
        n270 = control-ref of="ThreatSize_0"() -> (w489:refnum<vi>)
        n271 = control-ref of="Requestors_0"() -> (w492:refnum<vi>)
        n272 = call "Fill Lists from DB (1st Pass).vi"("error in"=w485, "RefNumArray"=w522) -> ("error out"=w474:errorcluster)  [unwired: 1 in, 4 out]
        n273 = flat-sequence {
          frame #0 {
            n274 = local write "RefreshMetadata"(FALSE ("UpdateMetadata")) -> ()
            n275 = local write "TimeNow"("Loading from BIMS Server . . ." ("TimeNow")) -> ()
          }
        }
        n276 = call "Fill Stitch Lists.vi"("error IN"=w474) -> ("error OUT"=w473:errorcluster)  [unwired: 6 in]
        n277 = Build Array(w489, w492) -> (w491:refnum<vi>[])
        n278 = call "Fill Lists from DB (2nd Pass).vi"("errorIN"=w473, "colNames"=string[] ["GrainSize", "requestor"] ("lkupTableNames"), "lkupTableNames"=string[] ["ThreatDetails", "Submitters"], "RefNumArray"=w491) -> ("error OUT"=w471:errorcluster)  [unwired: 3 in]
        n279 = property class="Str"(reference=w487, error in=w485, "Value"="filling dropdown lists") -> (reference out=w486:refnum<vi>)  [unwired: 1 out]
        n280 = property on="LayerStitchTypes" class="Ring (strict)"(error in=w471) -> ("Strings []"=w472:string[])  [unwired: 1 in, 2 out]
        n281 = call "Create local tables from Server DB.vi"("loadStatus Refnum"=w486, "error in"=w471, "Site"="Site", "tableNames"=string[] ["Threats", "ThreatDetails", "ThreatCalibers", "Mfrs", "SampleStyles", "SampleSpecs", "FiberTypes"]) -> ("error out"=w514:errorcluster)  [unwired: 7 out]
        n282 = call "Fill Lists From DB (3rd Pass).vi"("error IN"=w514) -> ("error OUT"=w495:errorcluster)  [unwired: 3 in, 3 out]
        n283 = property on="layerStitch_1" class="Ring (strict)"("Strings []"=w472) -> ()  [unwired: 2 in, 2 out]
        n284 = property on="layerStitch_2" class="Ring (strict)"("Strings []"=w472) -> ()  [unwired: 2 in, 2 out]
        n285 = property on="layerStitch_3" class="Ring (strict)"("Strings []"=w472) -> ()  [unwired: 2 in, 2 out]
        n286 = property on="layerStitch_4" class="Ring (strict)"("Strings []"=w472) -> ()  [unwired: 2 in, 2 out]
        n287 = property on="layerStitch_5" class="Ring (strict)"("Strings []"=w472) -> ()  [unwired: 2 in, 2 out]
        n288 = property on="layerStitch_6" class="Ring (strict)"("Strings []"=w472) -> ()  [unwired: 2 in, 2 out]
        n289 = control-ref of="ModelMfrs"() -> (w502:refnum<vi>)
        n290 = property class="Ring (strict)"(reference=w502, error in=w495) -> (reference out=w501:refnum<vi>, error out=w500:errorcluster, "Strings []"=w499:string[])
        n291 = Delete From Array(array=w499, length=1, index=0) -> (array with subset deleted=w498:string[])  [unwired: 1 out]
        n292 = property class="Ring (strict)"(reference=w501, error in=w500, "Strings []"=w498) -> (error out=w494:errorcluster)  [unwired: 1 out]
        n293 = case shown="No Error" w494 {
          selector: w494 -> [w531 w534]
          tunnel: [w531 w534] -> w511
          frame No Error {
            n294 = local write "TimeNow"("Collector Metadata is READY!" ("TimeNow")) -> ()
            n295 = Wait (ms)(milliseconds to wait=u32 2000) -> ()  [unwired: 1 out]
            "loadStatus" <- ""
          }
          frame Error {
            n296 = call <vilib>:"General Error Handler.vi"("error in (no error)"=w534) -> ()  [unwired: 2 in, 13 out]
          }
        }
        n297 = property on="Loading" class="Ring (strict)"(error in=w511, "Visible"=FALSE) -> (error out=w510:errorcluster)  [unwired: 1 in, 1 out]
      }
      event "loadingUnits": Value Change {
        n298 = local read "Powder Loading"() -> (w538:sgl)
        n299 = event-data() -> ("NewVal"=w537:enum32{"grams", "grains"})  [unwired: 6 out]
        n300 = case shown="\"grams\", Default" w537 {
          tunnel: w538 -> [w542 w543]
          frame "grams", Default {
            n301 = Multiply(x=w542, y=sgl 0.06479891) -> (x*y=w540:sgl)
            n302 = local write "Powder Loading"(w540) -> ()
          }
          frame "grains" {
            n303 = Multiply(x=w543, y=sgl 15.432359) -> (x*y=w544:sgl)
            n304 = local write "Powder Loading"(w544) -> ()
          }
        }
      }
      event "clearErrors": Value Change {
        w546 = errorcluster {"status"=FALSE, "code"=0, "source"=""} ("error in")
        n305 = event-data() -> ()  [unwired: 7 out]
        n306 = local write "SMErr"(w546) -> ()
      }
    }
    "U/I EvErr" <- w31
  }
  n307 = while "Test Executive State Machine" {
    shift-left: 100 -> [w555]
    shift-right: [w556] -> _
    shift-left: Collector_State."INITIALIZE" ("progState") -> [w552]
    shift-right: [w549] -> _
    shift-right: [w553] -> _
    shift-left: w26 -> [w554]
    shift-right: [w550] -> _
    shift-left: w22 -> [w551]
    tunnel: w3 -> [w547]
    stop <- FALSE stop-if-true
    n308 = case shown="\"PROC SHOTS\"" w552 {
      tunnel: [w576 w688 Collector_State."POLL" ("progState") Collector_State."POLL" ("progState") w1725 Collector_State."PROC SHOTS" ("progState") Collector_State."POLL" ("progState") Collector_State."PROC SHOTS" ("progState") Collector_State."PROC SHOTS" ("progState") Collector_State."POLL" ("progState") Collector_State."POLL" ("progState") w2326] -> w549
      tunnel: [-1 -1 ("index of element") -1 ("index of element") -1 ("index of element") w1724 -1 ("index of element") -1 -1 ("index of element") -1 ("index of element") -1 -1 ("index of element") w2325] -> w556
      tunnel: w555 -> [_ w689 _ _ _ _ _ _ _ _ _ _]
      tunnel: w554 -> [w579 w687 w840 w1473 w1719 w1954 w1996 w2006 w2024 w2075 w2089 w2327]
      tunnel: [w571 w686 w840 w1473 w1718 w1940 w2000 w2006 w2021 w2075 w2093 w2327] -> w553
      tunnel: w551 -> [_ w682 w837 w1471 w1721 w1950 w1992 w2009 w2020 w2072 w2088 w2319]
      tunnel: [w582 w683 w836 w1470 w1720 w1948 w1992 w2007 w2019 w2071 w2087 w2324] -> w550
      tunnel: w547 -> [_ _ _ _ _ _ _ _ _ _ _ w2318]
      frame "POLL", Default {
        w580 = Collector_State."POLL"  # progStateType
        w592 = TRUE  # element
        w595 = 4  # SAVE
        # "case # 0"
        # "This section checks for any buttons, maintains routine check of the parameters"
        n309 = case shown="\"Setup\", Default" "mainTabCntrl" {
          frame "Setup", Default {
            n310 = control-ref of="layerStitch_1"() -> (w612:refnum<vi>)
            n311 = control-ref of="layerStitch_2"() -> (w611:refnum<vi>)
            n312 = control-ref of="layerStitch_3"() -> (w610:refnum<vi>)
            n313 = control-ref of="layerStitch_4"() -> (w609:refnum<vi>)
            n314 = control-ref of="layerStitch_5"() -> (w608:refnum<vi>)
            n315 = control-ref of="layerStitch_6"() -> (w607:refnum<vi>)
            n316 = control-ref of="SampleStyle_0"() -> (w605:refnum<vi>)
            n317 = control-ref of="SampleStyle_1"() -> (w626:refnum<vi>)
            n318 = control-ref of="SampleStyle_2"() -> (w627:refnum<vi>)
            n319 = control-ref of="SampleStyle_3"() -> (w628:refnum<vi>)
            n320 = control-ref of="SampleStyle_4"() -> (w629:refnum<vi>)
            n321 = control-ref of="SampleStyle_5"() -> (w630:refnum<vi>)
            n322 = control-ref of="SampleStyle_6"() -> (w631:refnum<vi>)
            n323 = Build Array(w612, w611, w610, w609, w608, w607) -> (w613:refnum<vi>[])
            n324 = global write "BIMS_Collector Globals.vi" "LayerStitchTypeRefs"(w613) -> ()
            n325 = Build Array(w605, w626, w627, w628, w629, w630, w631) -> (w624:refnum<vi>[])
            n326 = global write "BIMS_Collector Globals.vi" "SampleStyles"(w624) -> ()
            n327 = local read "Fabric Description"() -> (w616:string)
            n328 = control-ref of="Mfr_0"() -> (w606:refnum<vi>)
            n329 = control-ref of="Mfr_1"() -> (w637:refnum<vi>)
            n330 = control-ref of="Mfr_2"() -> (w636:refnum<vi>)
            n331 = control-ref of="Mfr_3"() -> (w635:refnum<vi>)
            n332 = control-ref of="Mfr_4"() -> (w634:refnum<vi>)
            n333 = control-ref of="Mfr_5"() -> (w633:refnum<vi>)
            n334 = control-ref of="Mfr_6"() -> (w632:refnum<vi>)
            n335 = String Subset(string=w616, length (rest)=75 ("length (rest)")) -> (substring=w615:string)  [unwired: 1 out]
            n336 = Build Array(w606, w637, w636, w635, w634, w633, w632) -> (w625:refnum<vi>[])
            n337 = local write "Fabric Description"(w615) -> ()
            n338 = global write "BIMS_Collector Globals.vi" "Mfrs"(w625) -> ()
            n339 = local read "SampleAttribs_1"() -> (w618:T3)
            n340 = local read "SampleAttribs_2"() -> (w620:T3)
            n341 = local read "SampleAttribs_3"() -> (w621:T3)
            n342 = local read "SampleAttribs_4"() -> (w622:T3)
            n343 = local read "SampleAttribs_5"() -> (w623:T3)
            n344 = local read "SampleAttribs_6"() -> (w619:T3)
            n345 = Build Array(w618, w620, w621, w622, w623, w619) -> (w617:T27)
            n346 = global write "BIMS_Collector Globals.vi" "SampleAttribs"(w617) -> ()
          }
          frame "Measure" {
            # "Disable and gray out the \"Save\" button\nIF the shot table has no shots, \nOR if there are no plies; otherwise, enable it."
            # "Disable and gray out the \"Clear Shots\" button\nIF the shot table has no shots; otherwise, enable it."
            n347 = local read "shotsArr"() -> (w642:T6)
            n348 = local read "totalNumLayers"() -> (w640:i32)
            n349 = Equal To 0?(x=w640) -> (x = 0?=w641:bool)
            n350 = Array Size(array=w642) -> (size(s)=w652:i32)
            n351 = Equal To 0?(x=w652) -> (x = 0?=w639:bool)
            n352 = Or(x=w639, y=w641) -> (x .or. y?=w638:bool)
            n353 = property on="saveReq" class="Str"("Visible"=w638) -> ()  [unwired: 2 in, 2 out]
            n354 = Select(t=T15."Disabled and Grayed Out" ("Disabled"), s=w638, f=T15."Enabled" ("Disabled")) -> (s? t:f=w643:T15)
            n355 = Select(t=T15."Disabled and Grayed Out" ("Disabled"), s=w639, f=T15."Enabled" ("Disabled")) -> (s? t:f=w651:T15)
            n356 = property on="reportV50" class="Bool"("Disabled"=w643) -> ()  [unwired: 2 in, 2 out]
            n357 = property on="saveShots" class="Bool"("Disabled"=w643) -> ()  [unwired: 2 in, 2 out]
            n358 = property on="clearShots" class="Bool"("Disabled"=w651) -> ()  [unwired: 2 in, 2 out]
            n359 = local read "Shot Description"() -> (w650:string)
            n360 = String Subset(string=w650, length (rest)=30 ("length (rest)")) -> (substring=w648:string)  [unwired: 1 out]
            n361 = local write "Shot Description"(w648) -> ()
          }
          frame "History" {
          }
          frame "System" {
          }
        }
        n362 = Format Date/Time String(time format string (%c)="%x   %H:%M:%S") -> (date/time string=w568:string)  [unwired: 2 out]
        n363 = local write "shotTimestamp"(w568) -> ()
        n364 = Or(x="undoLastShot", y="deleteShot") -> (x .or. y?=w590:bool)
        n365 = Or(x="reportV50", y="reportV50_History") -> (x .or. y?=w598:bool)
        n366 = flat-sequence {
          tunnel: [w659] -> w581
          frame #0 {
            n367 = Wait (ms)(milliseconds to wait=u32 10 ("millisecond timer value")) -> ()  [unwired: 1 out]
          }
          frame #1 {
            n368 = local read "SMErr"() -> (w659:errorcluster)
          }
        }
        n369 = Build Array("RESET All", w598, "VsVr Report", "saveShots", "addShot", "clearShots", "nextShot", w590, "readyClock", "processShots") -> (w593:bool[])
        n370 = Search 1D Array(1D array=w593, element=w592) -> (index of element=w603:i32)  [unwired: 1 out]
        n371 = Increment(x=w603) -> (x+1=w604:i32)
        n372 = Equal?(x=w604, y=w595) -> (x = y?=w596:bool)
        n373 = case shown="False" w596 {
          tunnel: w604 -> [w661 w673]
          tunnel: [w662 w678] -> w602
          tunnel: w581 -> [w660 w669]
          tunnel: [w660 w667] -> w582
          frame False {
            w664 = 0  # Not Found
            n374 = Equal?(x=w661, y=w664) -> (x = y?=w663:bool)
            n375 = case shown="True" w663 {
              tunnel: w661 -> [w665 _]
              tunnel: [w665 w666] -> w662
              frame False {
              }
              frame True {
                w666 = 11  # CheckDAQ
                # "USUAL SCENARIO"
              }
            }
          }
          frame True {
            # "Before allowing data record to be saved,\nprompt user to validate."
            n376 = call "Get Last Record (SubVI).vi"("error in"=w669) -> ("error out"=w668:errorcluster, "experiment record"=w670:i32, "shot record"=w671:i32)  [unwired: 2 out]
            n377 = local write "lastSamp"(w670) -> ()
            n378 = local write "lastShot"(w671) -> ()
            n379 = To Double Precision Float(number=w670) -> (double precision float=w672:dbl)
            n380 = Two Button Dialog(message="Are ALL Data Valid?", 1:"NO" ("F button name (\"Cancel\")"), 2:"YES" ("T button name (\"OK\")")) -> (T button?=w677:bool)
            n381 = property on="Record #" class="DigNum (strict)"(error in=w668, "Maximum"=w672) -> (error out=w667:errorcluster)  [unwired: 1 in, 1 out]
            n382 = case shown="False" w677 {
              tunnel: [0 ("index of element") w680] -> w678
              tunnel: w673 -> [_ w680]
              frame False {
                # "POLL"
              }
              frame True {
              }
            }
          }
        }
        n383 = local read "shotsArr"() -> (w571:T6)
        n384 = for {
          tunnel: w579 -> [w656] mode=indexing
          tunnel: w571 -> [w657] mode=indexing
          tunnel: [w653] -> w578 mode=indexing
          n385 = Not Equal?(x=w657, y=w656) -> (x != y?=w655:T28)
          n386 = Cluster To Array(cluster=w655) -> (array=w654:bool[])
          n387 = Or Array Elements(Boolean array=w654) -> (logical OR=w653:bool)
        }
        n388 = Or Array Elements(Boolean array=w578) -> (logical OR=w574:bool)
        n389 = To Variant(anything=w602) -> (Variant=w601:variant)
        n390 = Variant To Data(type=w580, Variant=w601) -> (data=w577:T13)  [unwired: 1 in, 1 out]
        n391 = Select(t=Collector_State."PROC SHOTS" ("progStateType"), s=w574, f=w577) -> (s? t:f=w576:T13)
        "STOP (Shots MC LB)" <- TRUE ("STOP (Shots MC LB)")
      }
      frame "INITIALIZE" {
        # "case # 1"
        # "This section reads the ini file"
        n392 = case shown="100" w689 {
          tunnel: [w695 w714] -> w690
          tunnel: [w693 w714] -> w685
          tunnel: w682 -> [w692 w706]
          tunnel: [w691 w706] -> w681
          frame 0, Default {
            n393 = local read "RESET All"() -> (w694:bool)
            n394 = case shown="False" w694 {
              tunnel: [TRUE w702] -> w695
              tunnel: [FALSE w702] -> w693
              tunnel: w692 -> [w696 w699]
              tunnel: [w696 w699] -> w691
              frame False {
                # "Refresh"
              }
              frame True {
                n395 = Two Button Dialog(message="Resetting will remove all unsaved data.\n\nDo you really  want to reset? ", 1:"NO" ("F button name (\"Cancel\")"), 2:"YES" ("T button name (\"OK\")")) -> (T button?=w702:bool)
              }
            }
          }
          frame 100 {
            w714 = TRUE  # Reset ALL
            n396 = control-ref of="Mfr_0"() -> (w704:refnum<vi>)
            n397 = control-ref of="Mfr_1"() -> (w713:refnum<vi>)
            n398 = control-ref of="Mfr_2"() -> (w712:refnum<vi>)
            n399 = control-ref of="Mfr_3"() -> (w711:refnum<vi>)
            n400 = control-ref of="Mfr_4"() -> (w710:refnum<vi>)
            n401 = control-ref of="Mfr_5"() -> (w709:refnum<vi>)
            n402 = control-ref of="Mfr_6"() -> (w708:refnum<vi>)
            n403 = property on="Loading" class="Ring (strict)"("Visible"=FALSE) -> ()  [unwired: 2 in, 2 out]
            n404 = Build Array(w704, w713, w712, w711, w710, w709, w708) -> (w707:refnum<vi>[])
            n405 = global write "BIMS_Collector Globals.vi" "Mfrs"(w707) -> ()
          }
        }
        n406 = case shown="True" w690 {
          tunnel: [Collector_State."POLL" ("progState") w756] -> w688
          tunnel: w687 -> [w717 _]
          tunnel: [w717 "shotsArr"] -> w686
          tunnel: w685 -> [_ w757]
          tunnel: [w715 w724] -> w683
          tunnel: w681 -> [w715 w755]
          frame False {
            n407 = local write "RESET All"(FALSE ("RESET")) -> ()
          }
          frame True {
            n408 = case shown="True" w757 {
              selector: w757 -> [_ w783]
              tunnel: [w766 w783] -> w738
              tunnel: [w765 w798] -> w720
              tunnel: w755 -> [w765 w785]
              tunnel: [w764 w782] -> w726
              frame False {
                w766 = FALSE  # Reset All
                # "Refresh"
                n409 = local read "configPath"() -> (w764:path)
              }
              frame True {
                # "This section resets\nentire program"
                # "Reset ALL"
                n410 = control-ref of="This VI"() -> (w775:refnum<vi>)
                n411 = invoke on="Invoke Node" class="VI" method="Default Vals.Reinit All"(reference=w775, error in=w785) -> (reference out=w774:refnum<vi>, error out=w773:errorcluster)  [unwired: 1 in, 1 out]
                n412 = property class="VI"(reference=w774, error in=w773, "Front Panel.ShowMenuBar"=FALSE ("Front Panel Window:Show Menu Bar")) -> (reference out=w771:refnum<vi>, error out=w769:errorcluster)
                n413 = control-ref of="ScreenSetAvgg"() -> (w793:refnum<vi>)
                n414 = control-ref of="InterlockExists"() -> (w794:refnum<vi>)
                n415 = control-ref of="useBallisitican"() -> (w795:refnum<vi>)
                n416 = control-ref of="useRecorder"() -> (w796:refnum<vi>)
                n417 = control-ref of="useShooter"() -> (w797:refnum<vi>)
                n418 = control-ref of="useBMC"() -> (w768:refnum<vi>)
                n419 = property on="mainTabCntrl" class="TabCtl (strict)"() -> (error out=w777:errorcluster, "Pages"=w779:refnum<vi>[])  [unwired: 2 in, 1 out]
                n420 = Close Reference(reference=w771, error in (no error)=w769) -> (error out=w770:errorcluster)
                n421 = call "RegReadParams.vi"("ScreenSetAveraging_Ref"=w793, "useBMC_Ref"=w768, "InterlockExist_Ref"=w794, "errorIN"=w770, "useShooter_Ref"=w797, "useRecorder_Ref"=w796, "useBallistician_Ref"=w795) -> ("error out"=w792:errorcluster)  [unwired: 4 out]
                n422 = Index Array(array=w779, index=1) -> (element=w781:refnum<vi>)
                n423 = control-ref of="Server"() -> (w784:refnum<vi>)
                n424 = control-ref of="ConfigName"() -> (w788:refnum<vi>)
                n425 = control-ref of="Site"() -> (w786:refnum<vi>)
                n426 = control-ref of="Folder"() -> (w767:refnum<vi>)
                n427 = property on="Property Node" class="Page"(reference=w781, error in=w777, "PageEnb"=T16."Page Disabled & Grayed" ("Page Enabled State")) -> (error out=w776:errorcluster)  [unwired: 1 out]
                n428 = Build Array(w788, w786, w784, w767) -> (w789:refnum<vi>[])
                n429 = property on="minV50" class="DigNum (strict)"(error in=w776, "Visible"=w783) -> ()  [unwired: 1 in, 2 out]
                n430 = call "InitStringValuesFromRegistry(SubVI).vi"("error in"=w792, "String References"=w789, "subkey"="SOFTWARE\\DuPont\\BIMS-14\\Collector", "root key (HKEY_LOCAL_MACHINE)"=Registry_RtKey."HKEY_LOCAL_MACHINE") -> ("error out"=w791:errorcluster)  [unwired: 3 out]
                n431 = Current VI's Path() -> (path=w801:path)
                n432 = call "Initialize (SubVI).vi"("path"=w801, "error IN"=w791) -> ("pathConfigOUT"=w782:path, "lengthUnits"=→"lengthUnits":string, "massUnits"=→"massUnits":string, "error out"=w798:errorcluster)  [unwired: 1 out]
                "configPath" <- w782
              }
            }
            n433 = control-ref of="MeasSrc"() -> (w722:refnum<vi>)
            n434 = call "check timing board (SubVI).vi"("errIN"=w720, "ActiveDev"="ActiveDev", "measSrc_ref"=w722) -> ("error out"=w719:errorcluster, "deviceID"=→"Device S/N":string)  [unwired: 7 in]
            n435 = property on="Ballisticians" class="Ring (strict)"("Visible"="useBallisitican") -> ()  [unwired: 2 in, 2 out]
            n436 = property on="Shooters" class="Ring (strict)"("Visible"="useShooter") -> ()  [unwired: 2 in, 2 out]
            n437 = property on="Recorders" class="Ring (strict)"("Visible"="useRecorder") -> ()  [unwired: 2 in, 2 out]
            n438 = control-ref of="Threat"() -> (w741:refnum<vi>)
            n439 = control-ref of="SampleTypes"() -> (w743:refnum<vi>)
            n440 = control-ref of="SampleDescrip"() -> (w750:refnum<vi>)
            n441 = call "Get Threats (SubVI).vi"("pathConfigIN"=w726, "refThreat"=w741, "error in"=w719) -> ("pathConfigOUT"=w745:path, "factorOut"=→"factor array":sgl[], "error out"=w748:errorcluster)  [unwired: 4 out]
            n442 = Bundle("SampleTypes"=w743, "SampleDescrip"=w750) -> (w749:T29)  [unwired: 1 out]
            n443 = call "Fill Lists from INI (SubVI).vi"("clusterListboxes"=w749, "error in"=w748, "pathConfigIN"=w745) -> ("error out"=w747:errorcluster, "pathConfigOUT"=w746:path)  [unwired: 4 out]
            n444 = call "Read Parameters.vi"("error in (no error)"=w747, "appended path"=w746) -> ("error out"=w740:errorcluster, "rangeParams"=w742:T30)  [unwired: 4 out]
            n445 = Unbundle(w742) -> ("max dev"=w727:sgl, "residual separation"=→"Residual/Separation":sgl, "Set#1 Separation"=→"Set#1 Separation":sgl, "Set#2 Separation"=→"Set#2 Separation":sgl, "impact target dist"=w731:sgl, "resid target dist"=w732:sgl, "barrel screen dist"=→"Barrel to Screen":sgl, "midpt_to_target_dist"=→"mid_to_targ_dist":sgl)
            n446 = local write "maxDev"(w727) -> ()
            n447 = local write "Set#1_to_Target"(w731) -> ()
            n448 = local write "Residual/Target Dist"(w732) -> ()
            n449 = property on="RefreshMetadata" class="Bool (strict)"(error in=w740, "Val(Sgnl)"=TRUE) -> (error out=w735:errorcluster)  [unwired: 1 in, 1 out]
            n450 = case shown="True" w738 {
              tunnel: [Collector_State."POLL" ("progState") w824] -> w756
              tunnel: [w802 w804] -> w754
              tunnel: w735 -> [w802 w821]
              tunnel: w726 -> [_ w812]
              tunnel: "useBMC" -> [_ w811]
              frame False {
                # "Refresh"
              }
              frame True {
                w805 = T15."Disabled and Grayed Out" ("Disabled")
                # "Reset ALL"
                n451 = global read "BIMS_Collector Globals.vi" "SampleStyles"() -> (w814:refnum<vi>[])
                n452 = local read "InterlockExists"() -> (w823:bool)
                n453 = case shown="True" w811 {
                  tunnel: w812 -> [_ w826]
                  frame False {
                  }
                  frame True {
                    n454 = Path To String(path=w826) -> (string=w827:string)
                    n455 = call "Ballistics Message Center.vi"("INI File Name"=w827) -> ()
                  }
                }
                n456 = local read "MeasSrc"() -> (w825:T12)
                n457 = call "Get Last Record (SubVI).vi"("error in"=w821) -> ("error out"=w813:errorcluster, "experiment record"=w819:i32, "shot record"=→"lastShot":i32)  [unwired: 2 out]
                "lastSamp" <- w819
                n458 = control-ref of="ThreatDetails"() -> (w810:refnum<vi>)
                n459 = control-ref of="SampleStyle_0"() -> (w816:refnum<vi>)
                n460 = control-ref of="ThreatGroups"() -> (w815:refnum<vi>)
                n461 = To Double Precision Float(number=w819) -> (double precision float=w818:dbl)
                n462 = case shown="\"Screens\"" w825 {
                  tunnel: [Collector_State."POLL" ("progState") Collector_State."POLL" ("progState") Collector_State."READY CLOCK" ("progState")] -> w824
                  frame "Simulated", Default {
                  }
                  frame "Radar" {
                  }
                  frame "Screens" {
                    # "check for PCI 6602"
                  }
                }
                n463 = Build Array (concatenate)(w810, w816, w815, w814) -> (w817:refnum<vi>[])
                n464 = property on="Record #" class="DigNum (strict)"(error in=w813, "Maximum"=w818) -> (error out=w804:errorcluster)  [unwired: 1 in, 1 out]
                n465 = Select(t=T15."Enabled" ("Disabled"), s=w823, f=T15."Disabled and Grayed Out" ("Disabled")) -> (s? t:f=w822:T15)
                n466 = for {
                  tunnel: w817 -> [w828] mode=indexing
                  n467 = property on="Property Node" class="Ring (strict)"(reference=w828, "Strings []"=string[] []) -> ()  [unwired: 1 in, 2 out]
                }
                n468 = property on="addShot" class="Bool"("Disabled"=T15."Enabled") -> ()  [unwired: 2 in, 2 out]
                n469 = property on="undoLastShot" class="Bool"("Disabled"=w805) -> ()  [unwired: 2 in, 2 out]
                n470 = property on="saveShots" class="Bool"("Disabled"=w805) -> ()  [unwired: 2 in, 2 out]
                n471 = property on="clearShots" class="Bool"("Disabled"=w805) -> ()  [unwired: 2 in, 2 out]
                n472 = property on="ARM" class="Bool"("Disabled"=w822) -> ()  [unwired: 2 in, 2 out]
                n473 = property on="saveReq" class="Str"("Visible"=TRUE) -> ()  [unwired: 2 in, 2 out]
              }
            }
            n474 = call <vilib>:"General Error Handler.vi"("error in (no error)"=w754) -> ("error out"=w724:errorcluster)  [unwired: 2 in, 12 out]
            n475 = flat-sequence {
              tunnel: w724 -> [w758]
              frame #0 {
                n476 = local read "ConfigName"() -> (w759:string)
                n477 = case shown="No Error" w758 {
                  tunnel: [w762 "NOT READY!" ("ConfigName")] -> w760
                  tunnel: w759 -> [w762 _]
                  frame No Error {
                    n478 = Wait (ms)(milliseconds to wait=u32 1000) -> ()  [unwired: 1 out]
                  }
                  frame Error {
                  }
                }
                "ConfigName" <- w760
              }
            }
            "saveReq" <- "Number of layers in sample ply specification and number of shots in shots table must be greater than 0 to enable saving." ("saveReq")
          }
        }
      }
      frame "V50 Report or GET Record" {
        # "case # 2"
        # "The custom Excel template file is \nexpected in the C:\\Ballistics folder."
        n479 = case shown="False" "lookupRec" {
          selector: "lookupRec" -> [_ w1452]
          tunnel: [w884 w1442] -> w864
          tunnel: [w883 w1428] -> w863
          tunnel: [w882 w1445] -> w862
          tunnel: [w881 w1385] -> w861
          tunnel: [w880 w1443] -> w860
          tunnel: [w879 w1405] -> w859
          tunnel: [w878 w1392] -> w846
          tunnel: [w877 w1394] -> w845
          tunnel: [w876 w1395] -> w844
          tunnel: [w875 "Record #"] -> w843
          tunnel: [w874 w1444] -> w842
          tunnel: [w873 w1394] -> w835
          tunnel: w840 -> [w872 _]
          tunnel: [w871 w1417] -> w838
          tunnel: w837 -> [w871 w1418]
          tunnel: [w870 w1390] -> w833
          frame False {
            n480 = local read "Site"() -> (w869:string)
            n481 = stacked-sequence {
              tunnel: [_ _ _ _ _ w1285] -> w879
              tunnel: [_ w953 _ _ _ _] -> w883
              tunnel: [_ _ _ _ w1077 _] -> w880
              tunnel: [_ _ _ w1010 _ _] -> w881
              tunnel: [_ _ w976 _ _ _] -> w882
              tunnel: [w896 _ _ _ _ _] -> w884
              tunnel: [_ _ _ _ _ w1291] -> w878
              tunnel: [_ _ _ _ _ w1287] -> w877
              tunnel: [_ _ _ _ _ w1286] -> w876
              tunnel: [_ _ _ _ _ w1290] -> w875
              tunnel: [_ _ _ _ _ w1289] -> w874
              tunnel: [_ _ _ _ _ w1288] -> w873
              tunnel: w872 -> [_ _ w975 _ w1076 _]
              tunnel: w869 -> [_ _ w964 w1009 w1075 w1284]
              frame #0 {
                # "Need to remove first element\nsince it's associated with the \nhistory page."
                # "FABRIC"
                n482 = global read "BIMS_Collector Globals.vi" "SampleStyles"() -> (w887:refnum<vi>[])
                n483 = global read "BIMS_Collector Globals.vi" "Mfrs"() -> (w892:refnum<vi>[])
                n484 = global read "BIMS_Collector Globals.vi" "LayerStitchTypeRefs"() -> (w894:refnum<vi>[])
                n485 = local read "fab1_totalWt"() -> (w899:sgl)
                n486 = local read "fab2_totalWt"() -> (w900:sgl)
                n487 = local read "fab3_totalWt"() -> (w901:sgl)
                n488 = local read "fab4_totalWt"() -> (w902:sgl)
                n489 = local read "fab5_totalWt"() -> (w903:sgl)
                n490 = local read "fab6_totalWt"() -> (w904:sgl)
                n491 = global read "BIMS_Collector Globals.vi" "SampleAttribs"() -> (w885:T21)
                n492 = global read "BIMS_Collector Globals.vi" "LayerSpecs"() -> (w895:T31)
                n493 = Delete From Array(array=w887, length=1, index=0) -> (array with subset deleted=w886:refnum<vi>[])  [unwired: 1 out]
                n494 = Delete From Array "Delete From Array"(array=w892, length=1, index=0) -> (array with subset deleted=w893:refnum<vi>[])  [unwired: 1 out]
                n495 = Build Array(w899, w900, w901, w902, w903, w904) -> (w898:sgl[])
                n496 = for {
                  tunnel: w898 -> [w908] mode=indexing
                  tunnel: [w916] -> w897 mode=indexing
                  tunnel: w885 -> [w915] mode=indexing
                  tunnel: w895 -> [w914] mode=indexing
                  tunnel: w893 -> [w913] mode=indexing
                  tunnel: w886 -> [w912] mode=indexing
                  tunnel: w894 -> [w911] mode=indexing
                  n497 = call "Dropdown Selection (SubVI).vi"("reference"=w913) -> ("element"=w906:string)
                  n498 = call "Dropdown Selection (SubVI).vi"("reference"=w912) -> ("element"=w910:string)
                  n499 = Equal?(x="", y=w906) -> (x = y?=w905:bool)
                  n500 = call "Dropdown Selection (SubVI).vi"("reference"=w911) -> ("element"=w909:string)
                  n501 = case shown="False" w905 {
                    tunnel: [w935 w937] -> w916
                    tunnel: w915 -> [w934 _]
                    tunnel: w914 -> [w933 _]
                    tunnel: w910 -> [w927 _]
                    tunnel: w909 -> [w922 _]
                    tunnel: w908 -> [w920 _]
                    tunnel: w906 -> [w919 _]
                    frame False {
                      n502 = Unbundle By Name(w933) -> ("numOfPlies"=w921:i32, "LotNum"=w930:string, "RollNum"=w931:string)
                      n503 = Unbundle By Name(w934) -> ("internal_ID"=w925:string, "fiber"=w926:string, "denier"=w929:string, "pick"=w928:string, "weave"=w923:string, "finish"=w924:string, "ozPerYd2"=w932:string)
                      n504 = Format Into String(w921) -> (resulting string=w918:string)  [unwired: 3 in, 1 out]
                      n505 = Format Into String(w920) -> (resulting string=w917:string)  [unwired: 3 in, 1 out]
                      n506 = Build Array(w918, w919, w927, w925, w926, w929, w928, w923, w924, w930, w931, w932, w917, w922) -> (w935:string[])
                    }
                    frame True {
                      n507 = Initialize Array("", 14 ("dimension size")) -> (w937:string[])
                    }
                  }
                }
                n508 = Transpose 2D Array(2D array=w897) -> (transposed array=w896:string[][])
              }
              frame #1 {
                w939 = "%.1f" ("format string")
                # "muzzel / midpoint"
                # "muzzle / scr#1"
                # "muzzle / target"
                # "scr#2 / target"
                # "RANGE"
                n509 = local read "Set#1 Separation"() -> (w946:sgl)
                n510 = local read "mid_to_targ_dist"() -> (w943:sgl)
                n511 = local read "Barrel to Screen"() -> (w940:sgl)
                n512 = local read "clayAverage"() -> (w961:sgl)
                n513 = Divide(x=w946, y=sgl 2.0) -> (x/y=w941:sgl)
                n514 = local read "RoomHum"() -> (w956:sgl)
                n515 = local read "clayTemp"() -> (w959:sgl)
                n516 = local read "clayCalib"() -> (w962:string)
                n517 = local read "RoomT"() -> (w957:sgl)
                n518 = Add(x=w940, y=w943) -> (x+y=w947:sgl)
                n519 = Subtract(x=w940, y=w941) -> (x-y=w942:sgl)
                n520 = Subtract(x=w943, y=w941) -> (x-y=w944:sgl)
                n521 = Format Into String(w947) -> (resulting string=w948:string)  [unwired: 3 in, 1 out]
                n522 = Format Into String(w942) -> (resulting string=w949:string)  [unwired: 3 in, 1 out]
                n523 = Format Into String(w946) -> (resulting string=w950:string)  [unwired: 3 in, 1 out]
                n524 = Format Into String(w944) -> (resulting string=w951:string)  [unwired: 3 in, 1 out]
                n525 = Format Into String(w943) -> (resulting string=w952:string)  [unwired: 3 in, 1 out]
                n526 = Format Into String(w956) -> (resulting string=w954:string)  [unwired: 3 in, 1 out]
                n527 = Format Into String(format string=w939, w957) -> (resulting string=w955:string)  [unwired: 2 in, 1 out]
                n528 = Format Into String(format string=w939, w959) -> (resulting string=w958:string)  [unwired: 2 in, 1 out]
                n529 = Format Into String(format string=w939, w961) -> (resulting string=w960:string)  [unwired: 2 in, 1 out]
                n530 = Bundle(w948, w949, w950, w951, w952, w954, w955, w958, "clayCalib"=w962, w960) -> (w963:T32)  [unwired: 1 out]
                n531 = Cluster To Array(cluster=w963) -> (array=w953:string[])
              }
              frame #2 {
                # "RESULTS"
                n532 = for {
                  tunnel: w975 -> [w1008] mode=indexing
                  tunnel: [w1007] -> w974 mode=indexing
                  tunnel: [w1006] -> w973
                  i -> [w1006]
                  n533 = Unbundle By Name(w1008) -> ("BackFace\nDepth"=w1007:sgl)
                }
                n534 = Increment(x=w973) -> (x+1=w971:i32)
                n535 = Add Array Elements(numeric array=w974) -> (sum=w972:sgl)
                n536 = To Single Precision Float(number=w971) -> (single precision float=w970:sgl)
                n537 = control-ref of="Methods"() -> (w965:refnum<vi>)
                n538 = Divide(x=w972, y=w970) -> (x/y=w969:sgl)
                n539 = call "Dropdown Selection (SubVI).vi"("reference"=w965) -> ("element"=w966:string)
                n540 = Format Into String(format string="%1.1f", w969) -> (resulting string=w968:string)  [unwired: 2 in, 1 out]
                n541 = case shown="\"V50\"" w966 {
                  tunnel: [w994 w1005] -> w978
                  tunnel: w968 -> [w984 w1004]
                  tunnel: w964 -> [w983 _]
                  frame "V50" {
                    w988 = "%1d" ("format string")
                    n542 = local read "Z.M.R."() -> (w980:sgl)
                    n543 = local read "rangeOfResults"() -> (w990:i32)
                    n544 = local read "computed_V50"() -> (w993:sgl)
                    n545 = local read "lowComplete"() -> (w991:i32)
                    n546 = local read "highPartial"() -> (w992:i32)
                    n547 = Less Than 0?(x=w980) -> (x < 0?=w981:bool)
                    n548 = Select(t=sgl 0.0 ("Z.M.R."), s=w981, f=w980) -> (s? t:f=w979:sgl)
                    n549 = case shown="\"BRZ\"" w983 {
                      tunnel: [w999 w1001] -> w985
                      tunnel: w984 -> [w999 _]
                      frame Default {
                      }
                      frame "BRZ" {
                        n550 = local read "velSTDEV"() -> (w1002:sgl)
                        n551 = Format Into String(format string="%1.1f", w1002) -> (resulting string=w1001:string)  [unwired: 2 in, 1 out]
                      }
                    }
                    n552 = Format Into String(format string="%1.1f", w993) -> (resulting string=w997:string)  [unwired: 2 in, 1 out]
                    n553 = Format Into String(format string=w988, w992) -> (resulting string=w996:string)  [unwired: 2 in, 1 out]
                    n554 = Format Into String(format string=w988, w991) -> (resulting string=w995:string)  [unwired: 2 in, 1 out]
                    n555 = Format Into String(format string=w988, w990) -> (resulting string=w998:string)  [unwired: 2 in, 1 out]
                    n556 = Format Into String(format string="%1.1f", w979) -> (resulting string=w987:string)  [unwired: 2 in, 1 out]
                    n557 = Bundle(w997, w996, w995, w998, w987, w985, w984) -> (w994:T33)  [unwired: 1 out]
                  }
                  frame Default {
                    w1003 = "" ("Empty String Constant")
                    n558 = Bundle(w1003, w1003, w1003, w1003, w1003, w1004, w1004) -> (w1005:T33)  [unwired: 1 out]
                  }
                }
                n559 = Cluster To Array(cluster=w978) -> (array=w977:string[])
                n560 = Build Array(w977) -> (w976:string[][])
              }
              frame #3 {
                # "SAMPLE"
                n561 = case shown="\"ICE1\", Default" w1009 {
                  tunnel: [w1012 w1036 w1049 w1062] -> w1010
                  frame "ICE1", Default {
                    # "PB Req"
                    n562 = control-ref of="Methods"() -> (w1013:refnum<vi>)
                    n563 = call "Dropdown Selection (SubVI).vi"("reference"=w1013) -> ("element"=w1015:string)
                    n564 = Equal?(x=w1015, y="V50") -> (x = y?=w1014:bool)
                    n565 = local read "totalSampleWt"() -> (w1025:sgl)
                    n566 = case shown="True" w1014 {
                      tunnel: ["n/a" w1035] -> w1019
                      frame False {
                      }
                      frame True {
                        n567 = local read "minV50"() -> (w1034:i32)
                        n568 = Format Into String(w1034) -> (resulting string=w1035:string)  [unwired: 3 in, 1 out]
                      }
                    }
                    n569 = control-ref of="SampleDimensions"() -> (w1031:refnum<vi>)
                    n570 = control-ref of="SampleCoverings"() -> (w1032:refnum<vi>)
                    n571 = control-ref of="Models"() -> (w1018:refnum<vi>)
                    n572 = local read "serialNum"() -> (w1027:string)
                    n573 = local read "SampleID"() -> (w1029:string)
                    n574 = local read "Thickness"() -> (w1022:dbl)
                    n575 = local read "totalBAW"() -> (w1021:sgl)
                    n576 = call "Dropdown Selection (SubVI).vi"("reference"=w1031) -> ("element"=w1028:string)
                    n577 = call "Dropdown Selection (SubVI).vi"("reference"=w1018) -> ("element"=w1017:string)
                    n578 = call "Dropdown Selection (SubVI).vi"("reference"=w1032) -> ("element"=w1026:string)
                    n579 = Format Into String(w1025) -> (resulting string=w1024:string)  [unwired: 3 in, 1 out]
                    n580 = Format Into String(w1022) -> (resulting string=w1023:string)  [unwired: 3 in, 1 out]
                    n581 = Format Into String(w1021) -> (resulting string=w1020:string)  [unwired: 3 in, 1 out]
                    n582 = Bundle("SampleID"=w1029, "element"=w1028, "Type of work"="Type of work", "serialNum"=w1027, "element"=w1017, w1024, w1023, w1020, "element"=w1026, w1019) -> (w1030:T34)  [unwired: 1 out]
                    n583 = Cluster To Array(cluster=w1030) -> (array=w1012:string[])
                  }
                  frame "SPR0" {
                    n584 = local read "totalSampleWt"() -> (w1042:sgl)
                    n585 = control-ref of="SampleDimensions"() -> (w1047:refnum<vi>)
                    n586 = control-ref of="SampleCoverings"() -> (w1048:refnum<vi>)
                    n587 = local read "SampleID"() -> (w1045:string)
                    n588 = local read "Thickness"() -> (w1039:dbl)
                    n589 = local read "totalBAW"() -> (w1038:sgl)
                    n590 = call "Dropdown Selection (SubVI).vi"("reference"=w1047) -> ("element"=w1044:string)
                    n591 = call "Dropdown Selection (SubVI).vi"("reference"=w1048) -> ("element"=w1043:string)
                    n592 = Format Into String(w1042) -> (resulting string=w1041:string)  [unwired: 3 in, 1 out]
                    n593 = Format Into String(w1039) -> (resulting string=w1040:string)  [unwired: 3 in, 1 out]
                    n594 = Format Into String(w1038) -> (resulting string=w1037:string)  [unwired: 3 in, 1 out]
                    n595 = Bundle("SampleID"=w1045, "element"=w1044, w1041, w1040, w1037, "element"=w1043) -> (w1046:T35)  [unwired: 1 out]
                    n596 = Cluster To Array(cluster=w1046) -> (array=w1036:string[])
                  }
                  frame "SPR1" {
                    n597 = local read "totalSampleWt"() -> (w1055:sgl)
                    n598 = control-ref of="SampleDimensions"() -> (w1060:refnum<vi>)
                    n599 = control-ref of="SampleCoverings"() -> (w1061:refnum<vi>)
                    n600 = local read "Thickness"() -> (w1052:dbl)
                    n601 = local read "totalBAW"() -> (w1051:sgl)
                    n602 = local read "SampleID"() -> (w1058:string)
                    n603 = call "Dropdown Selection (SubVI).vi"("reference"=w1060) -> ("element"=w1057:string)
                    n604 = call "Dropdown Selection (SubVI).vi"("reference"=w1061) -> ("element"=w1056:string)
                    n605 = Format Into String(w1055) -> (resulting string=w1054:string)  [unwired: 3 in, 1 out]
                    n606 = Format Into String(w1052) -> (resulting string=w1053:string)  [unwired: 3 in, 1 out]
                    n607 = Format Into String(w1051) -> (resulting string=w1050:string)  [unwired: 3 in, 1 out]
                    n608 = Bundle("SampleID"=w1058, "element"=w1057, w1054, w1053, w1050, "element"=w1056) -> (w1059:T35)  [unwired: 1 out]
                    n609 = Cluster To Array(cluster=w1059) -> (array=w1049:string[])
                  }
                  frame "BRZ" {
                    n610 = local read "totalSampleWt"() -> (w1068:sgl)
                    n611 = control-ref of="SampleDimensions"() -> (w1073:refnum<vi>)
                    n612 = control-ref of="SampleCoverings"() -> (w1074:refnum<vi>)
                    n613 = local read "SampleID"() -> (w1071:string)
                    n614 = local read "Thickness"() -> (w1065:dbl)
                    n615 = local read "totalBAW"() -> (w1064:sgl)
                    n616 = call "Dropdown Selection (SubVI).vi"("reference"=w1073) -> ("element"=w1070:string)
                    n617 = call "Dropdown Selection (SubVI).vi"("reference"=w1074) -> ("element"=w1069:string)
                    n618 = Format Into String(w1068) -> (resulting string=w1067:string)  [unwired: 3 in, 1 out]
                    n619 = Format Into String(w1065) -> (resulting string=w1066:string)  [unwired: 3 in, 1 out]
                    n620 = Format Into String(w1064) -> (resulting string=w1063:string)  [unwired: 3 in, 1 out]
                    n621 = Bundle("SampleID"=w1071, "element"=w1070, w1067, w1066, w1063, "element"=w1069) -> (w1072:T35)  [unwired: 1 out]
                    n622 = Cluster To Array(cluster=w1072) -> (array=w1062:string[])
                  }
                }
              }
              frame #4 {
                n623 = case shown="\"SPR0\"" w1075 {
                  tunnel: [w1087 w1137 w1189 w1241] -> w1077
                  tunnel: w1076 -> [w1080 w1130 w1182 w1234]
                  frame "ICE1", Default {
                    # "SHOT TABLE"
                    n624 = control-ref of="Methods"() -> (w1079:refnum<vi>)
                    n625 = call "Dropdown Selection (SubVI).vi"("reference"=w1079) -> ("element"=w1078:string)
                    n626 = for {
                      tunnel: w1080 -> [w1119] mode=indexing
                      shift-right: [w1096] -> _
                      shift-left: T25 [] -> [w1098]
                      tunnel: [w1096] -> w1083
                      tunnel: w1078 -> [w1092]
                      n627 = Unbundle By Name(w1119) -> ("shot order"=w1118:i32, "Powder Loading"=w1117:sgl, "Uncorrected Impact"=w1116:sgl, "UncorrectedRed_PB"=w1115:sgl, "UncorrectedAvgVel_PB"=w1114:sgl, "velLoss_PB"=w1113:sgl, "strikeVel_PB"=w1112:sgl, "SHOT STATUS"=w1101:u16, "usedv50"=w1111:bool, "Shot Angle"=w1093:u16, "BackFace\nDepth"=w1094:sgl)
                      n628 = case shown="\"V50\"" w1092 {
                        tunnel: w1111 -> [w1121 _]
                        tunnel: [w1120 w1125] -> w1110
                        tunnel: w1093 -> [_ w1124]
                        frame "V50" {
                          n629 = case shown="True" w1121 {
                            tunnel: ["" ("Empty String Constant") "*"] -> w1120
                            frame False {
                            }
                            frame True {
                            }
                          }
                        }
                        frame Default {
                          n630 = Format Into String(w1124) -> (resulting string=w1125:string)  [unwired: 3 in, 1 out]
                        }
                      }
                      n631 = case shown="1" w1101 {
                        tunnel: ["P" "C"] -> w1100
                        frame 0, Default {
                        }
                        frame 1 {
                        }
                      }
                      n632 = Format Into String(format string="%2d", w1118) -> (resulting string=w1103:string)  [unwired: 2 in, 1 out]
                      n633 = Format Into String(w1117) -> (resulting string=w1104:string)  [unwired: 3 in, 1 out]
                      n634 = Format Into String(w1116) -> (resulting string=w1105:string)  [unwired: 3 in, 1 out]
                      n635 = Format Into String(w1115) -> (resulting string=w1106:string)  [unwired: 3 in, 1 out]
                      n636 = Format Into String(w1114) -> (resulting string=w1107:string)  [unwired: 3 in, 1 out]
                      n637 = Format Into String(w1113) -> (resulting string=w1108:string)  [unwired: 3 in, 1 out]
                      n638 = Format Into String(w1112) -> (resulting string=w1109:string)  [unwired: 3 in, 1 out]
                      n639 = Format Into String(w1094) -> (resulting string=w1102:string)  [unwired: 3 in, 1 out]
                      n640 = Build Array(w1103, w1104, w1105, w1106, w1107, w1108, w1109, w1100, w1110, w1102) -> (w1097:string[])
                      n641 = Array To Cluster(array=w1097) -> (cluster=w1099:T36)
                      n642 = Build Array (concatenate)(w1098, w1099) -> (w1096:T25)
                    }
                    n643 = Array Size(array=w1083) -> (size(s)=w1085:i32)
                    n644 = Equal To 0?(x=w1085) -> (x = 0?=w1081:bool)
                    n645 = case shown="True" w1081 {
                      tunnel: [w1088 T25 [{"[0]"="", "[1]"="", "[2]"="", "[3]"="", "[4]"="", "[5]"="", "[6]"="", "[7]"="", "[8]"="", "[9]"=""}]] -> w1082
                      tunnel: w1083 -> [w1088 _]
                      frame False {
                      }
                      frame True {
                      }
                    }
                    n646 = Sort 1D Array(array=w1082) -> (sorted array=w1084:T25)
                    n647 = for {
                      tunnel: w1084 -> [w1091] mode=indexing
                      tunnel: [w1090] -> w1087 mode=indexing
                      n648 = Cluster To Array(cluster=w1091) -> (array=w1090:string[])
                    }
                  }
                  frame "SPR0" {
                    # "SHOT TABLE"
                    n649 = control-ref of="Methods"() -> (w1129:refnum<vi>)
                    n650 = call "Dropdown Selection (SubVI).vi"("reference"=w1129) -> ("element"=w1128:string)
                    n651 = for {
                      tunnel: w1130 -> [w1167] mode=indexing
                      shift-right: [w1148] -> _
                      shift-left: T26 [] -> [w1150]
                      tunnel: [w1148] -> w1133
                      tunnel: w1128 -> [w1144]
                      n652 = Unbundle By Name(w1167) -> ("shot order"=w1166:i32, "Powder Loading"=w1165:sgl, "Uncorrected Impact"=w1164:sgl, "UncorrectedRed_PB"=w1163:sgl, "strikeVel_PB"=w1162:sgl, "SHOT STATUS"=w1153:u16, "usedv50"=w1161:bool, "Shot Angle"=w1145:u16, "BackFace\nDepth"=w1146:sgl, "V50userExcl"=w1143:bool, "Shot Description"=w1142:string)
                      n653 = case shown="\"V50\"" w1144 {
                        tunnel: w1161 -> [w1170 _]
                        tunnel: [w1169 w1177] -> w1160
                        tunnel: w1145 -> [_ w1176]
                        tunnel: w1143 -> [w1168 _]
                        frame "V50" {
                          n654 = case shown="True" w1168 {
                            tunnel: w1170 -> [w1172 _]
                            tunnel: [w1171 "!"] -> w1169
                            frame False {
                              n655 = case shown="False" w1172 {
                                tunnel: ["" ("Empty String Constant") "*"] -> w1171
                                frame False {
                                }
                                frame True {
                                }
                              }
                            }
                            frame True {
                            }
                          }
                        }
                        frame Default {
                          n656 = Format Into String(w1176) -> (resulting string=w1177:string)  [unwired: 3 in, 1 out]
                        }
                      }
                      n657 = case shown="1" w1153 {
                        tunnel: ["P" "C"] -> w1152
                        frame 0, Default {
                        }
                        frame 1 {
                        }
                      }
                      n658 = Format Into String(format string="%2d", w1166) -> (resulting string=w1155:string)  [unwired: 2 in, 1 out]
                      n659 = Format Into String(w1165) -> (resulting string=w1156:string)  [unwired: 3 in, 1 out]
                      n660 = Format Into String(w1164) -> (resulting string=w1157:string)  [unwired: 3 in, 1 out]
                      n661 = Format Into String(w1163) -> (resulting string=w1158:string)  [unwired: 3 in, 1 out]
                      n662 = Format Into String(w1162) -> (resulting string=w1159:string)  [unwired: 3 in, 1 out]
                      n663 = Format Into String(w1146) -> (resulting string=w1154:string)  [unwired: 3 in, 1 out]
                      n664 = Build Array(w1155, w1156, w1157, w1158, w1159, w1152, w1160, w1154, w1142) -> (w1149:string[])
                      n665 = Array To Cluster(array=w1149) -> (cluster=w1151:T37)
                      n666 = Build Array (concatenate)(w1150, w1151) -> (w1148:T26)
                    }
                    n667 = Array Size(array=w1133) -> (size(s)=w1135:i32)
                    n668 = Equal To 0?(x=w1135) -> (x = 0?=w1131:bool)
                    n669 = case shown="True" w1131 {
                      tunnel: [w1138 T26 [{"[0]"="", "[1]"="", "[2]"="", "[3]"="", "[4]"="", "[5]"="", "[6]"="", "[7]"="", "[8]"=""}]] -> w1132
                      tunnel: w1133 -> [w1138 _]
                      frame False {
                      }
                      frame True {
                      }
                    }
                    n670 = Sort 1D Array(array=w1132) -> (sorted array=w1134:T26)
                    n671 = for {
                      tunnel: w1134 -> [w1141] mode=indexing
                      tunnel: [w1140] -> w1137 mode=indexing
                      n672 = Cluster To Array(cluster=w1141) -> (array=w1140:string[])
                    }
                  }
                  frame "SPR1" {
                    # "SHOT TABLE"
                    n673 = control-ref of="Methods"() -> (w1181:refnum<vi>)
                    n674 = call "Dropdown Selection (SubVI).vi"("reference"=w1181) -> ("element"=w1180:string)
                    n675 = for {
                      tunnel: w1182 -> [w1219] mode=indexing
                      shift-right: [w1200] -> _
                      shift-left: T26 [] -> [w1202]
                      tunnel: [w1200] -> w1185
                      tunnel: w1180 -> [w1196]
                      n676 = Unbundle By Name(w1219) -> ("shot order"=w1218:i32, "Powder Loading"=w1217:sgl, "Uncorrected Impact"=w1216:sgl, "UncorrectedRed_PB"=w1215:sgl, "strikeVel_PB"=w1214:sgl, "SHOT STATUS"=w1205:u16, "usedv50"=w1213:bool, "Shot Angle"=w1197:u16, "BackFace\nDepth"=w1198:sgl, "V50userExcl"=w1195:bool, "Shot Description"=w1194:string)
                      n677 = case shown="\"V50\"" w1196 {
                        tunnel: w1213 -> [w1222 _]
                        tunnel: [w1221 w1229] -> w1212
                        tunnel: w1197 -> [_ w1228]
                        tunnel: w1195 -> [w1220 _]
                        frame "V50" {
                          n678 = case shown="True" w1220 {
                            tunnel: w1222 -> [w1224 _]
                            tunnel: [w1223 "!"] -> w1221
                            frame False {
                              n679 = case shown="False" w1224 {
                                tunnel: ["" ("Empty String Constant") "*"] -> w1223
                                frame False {
                                }
                                frame True {
                                }
                              }
                            }
                            frame True {
                            }
                          }
                        }
                        frame Default {
                          n680 = Format Into String(w1228) -> (resulting string=w1229:string)  [unwired: 3 in, 1 out]
                        }
                      }
                      n681 = case shown="1" w1205 {
                        tunnel: ["P" "C"] -> w1204
                        frame 0, Default {
                        }
                        frame 1 {
                        }
                      }
                      n682 = Format Into String(format string="%2d", w1218) -> (resulting string=w1207:string)  [unwired: 2 in, 1 out]
                      n683 = Format Into String(w1217) -> (resulting string=w1208:string)  [unwired: 3 in, 1 out]
                      n684 = Format Into String(w1216) -> (resulting string=w1209:string)  [unwired: 3 in, 1 out]
                      n685 = Format Into String(w1215) -> (resulting string=w1210:string)  [unwired: 3 in, 1 out]
                      n686 = Format Into String(w1214) -> (resulting string=w1211:string)  [unwired: 3 in, 1 out]
                      n687 = Format Into String(w1198) -> (resulting string=w1206:string)  [unwired: 3 in, 1 out]
                      n688 = Build Array(w1207, w1208, w1209, w1210, w1211, w1204, w1212, w1206, w1194) -> (w1201:string[])
                      n689 = Array To Cluster(array=w1201) -> (cluster=w1203:T37)
                      n690 = Build Array (concatenate)(w1202, w1203) -> (w1200:T26)
                    }
                    n691 = Array Size(array=w1185) -> (size(s)=w1187:i32)
                    n692 = Equal To 0?(x=w1187) -> (x = 0?=w1183:bool)
                    n693 = case shown="True" w1183 {
                      tunnel: [w1190 T26 [{"[0]"="", "[1]"="", "[2]"="", "[3]"="", "[4]"="", "[5]"="", "[6]"="", "[7]"="", "[8]"=""}]] -> w1184
                      tunnel: w1185 -> [w1190 _]
                      frame False {
                      }
                      frame True {
                      }
                    }
                    n694 = Sort 1D Array(array=w1184) -> (sorted array=w1186:T26)
                    n695 = for {
                      tunnel: w1186 -> [w1193] mode=indexing
                      tunnel: [w1192] -> w1189 mode=indexing
                      n696 = Cluster To Array(cluster=w1193) -> (array=w1192:string[])
                    }
                  }
                  frame "BRZ" {
                    # "SHOT TABLE"
                    n697 = control-ref of="Methods"() -> (w1233:refnum<vi>)
                    n698 = call "Dropdown Selection (SubVI).vi"("reference"=w1233) -> ("element"=w1232:string)
                    n699 = for {
                      tunnel: w1234 -> [w1271] mode=indexing
                      shift-right: [w1252] -> _
                      shift-left: T26 [] -> [w1254]
                      tunnel: [w1252] -> w1237
                      tunnel: w1232 -> [w1248]
                      n700 = Unbundle By Name(w1271) -> ("shot order"=w1270:i32, "Powder Loading"=w1269:sgl, "Uncorrected Impact"=w1268:sgl, "UncorrectedRed_PB"=w1267:sgl, "strikeVel_PB"=w1266:sgl, "SHOT STATUS"=w1257:u16, "usedv50"=w1265:bool, "Shot Angle"=w1249:u16, "BackFace\nDepth"=w1250:sgl, "V50userExcl"=w1247:bool, "Shot Description"=w1246:string)
                      n701 = case shown="\"V50\"" w1248 {
                        tunnel: w1265 -> [w1274 _]
                        tunnel: [w1273 w1281] -> w1264
                        tunnel: w1249 -> [_ w1280]
                        tunnel: w1247 -> [w1272 _]
                        frame "V50" {
                          n702 = case shown="True" w1272 {
                            tunnel: w1274 -> [w1276 _]
                            tunnel: [w1275 "!"] -> w1273
                            frame False {
                              n703 = case shown="False" w1276 {
                                tunnel: ["" ("Empty String Constant") "*"] -> w1275
                                frame False {
                                }
                                frame True {
                                }
                              }
                            }
                            frame True {
                            }
                          }
                        }
                        frame Default {
                          n704 = Format Into String(w1280) -> (resulting string=w1281:string)  [unwired: 3 in, 1 out]
                        }
                      }
                      n705 = case shown="1" w1257 {
                        tunnel: ["P" "C"] -> w1256
                        frame 0, Default {
                        }
                        frame 1 {
                        }
                      }
                      n706 = Format Into String(format string="%2d", w1270) -> (resulting string=w1259:string)  [unwired: 2 in, 1 out]
                      n707 = Format Into String(w1269) -> (resulting string=w1260:string)  [unwired: 3 in, 1 out]
                      n708 = Format Into String(w1268) -> (resulting string=w1261:string)  [unwired: 3 in, 1 out]
                      n709 = Format Into String(w1267) -> (resulting string=w1262:string)  [unwired: 3 in, 1 out]
                      n710 = Format Into String(w1266) -> (resulting string=w1263:string)  [unwired: 3 in, 1 out]
                      n711 = Format Into String(w1250) -> (resulting string=w1258:string)  [unwired: 3 in, 1 out]
                      n712 = Build Array(w1259, w1260, w1261, w1262, w1263, w1256, w1264, w1258, w1246) -> (w1253:string[])
                      n713 = Array To Cluster(array=w1253) -> (cluster=w1255:T37)
                      n714 = Build Array (concatenate)(w1254, w1255) -> (w1252:T26)
                    }
                    n715 = Array Size(array=w1237) -> (size(s)=w1239:i32)
                    n716 = Equal To 0?(x=w1239) -> (x = 0?=w1235:bool)
                    n717 = case shown="True" w1235 {
                      tunnel: [w1242 T26 [{"[0]"="", "[1]"="", "[2]"="", "[3]"="", "[4]"="", "[5]"="", "[6]"="", "[7]"="", "[8]"=""}]] -> w1236
                      tunnel: w1237 -> [w1242 _]
                      frame False {
                      }
                      frame True {
                      }
                    }
                    n718 = Sort 1D Array(array=w1236) -> (sorted array=w1238:T26)
                    n719 = for {
                      tunnel: w1238 -> [w1245] mode=indexing
                      tunnel: [w1244] -> w1241 mode=indexing
                      n720 = Cluster To Array(cluster=w1245) -> (array=w1244:string[])
                    }
                  }
                }
              }
              frame #5 {
                n721 = case shown="\"ICE1\", Default" w1284 {
                  tunnel: [w1315 w1336 w1356 w1376] -> w1291
                  tunnel: [w1314 w1335 w1355 w1375] -> w1290
                  tunnel: [w1313 w1334 w1354 w1374] -> w1289
                  tunnel: [w1312 w1319 w1339 w1359] -> w1288
                  tunnel: ["" ("projNum") w1319 w1339 w1359] -> w1287
                  tunnel: [w1310 w1333 w1353 w1373] -> w1286
                  tunnel: [w1294 w1322 w1342 w1362] -> w1285
                  frame "ICE1", Default {
                    # "THREAT"
                    # "Range # (supports a PB reporting requirement)"
                    # "Project Name goes here.\nSupports a PB reporting requirement."
                    # "GENERAL"
                    n722 = local read "threatDetails"() -> (w1293:T1)
                    n723 = Unbundle By Name(w1293) -> ("barrelLength"=w1297:string)
                    n724 = Unbundle By Name(w1293) -> ("grainSize"=w1292:string)
                    n725 = local read "Shot Angle"() -> (w1298:u16)
                    n726 = control-ref of="WeaponTypes"() -> (w1307:refnum<vi>)
                    n727 = control-ref of="ThreatGroups"() -> (w1306:refnum<vi>)
                    n728 = control-ref of="PowderTypes"() -> (w1305:refnum<vi>)
                    n729 = control-ref of="Recorders"() -> (w1308:refnum<vi>)
                    n730 = control-ref of="Shooters"() -> (w1309:refnum<vi>)
                    n731 = Format Into String(w1298) -> (resulting string=w1299:string)  [unwired: 3 in, 1 out]
                    n732 = call "Dropdown Selection (SubVI).vi"("reference"=w1307) -> ("element"=w1303:string)
                    n733 = call "Dropdown Selection (SubVI).vi"("reference"=w1306) -> ("element"=w1302:string)
                    n734 = call "Dropdown Selection (SubVI).vi"("reference"=w1305) -> ("element"=w1301:string)
                    n735 = call "Dropdown Selection (SubVI).vi"("reference"=w1308) -> ("element"=w1300:string)
                    n736 = call "Dropdown Selection (SubVI).vi"("reference"=w1309) -> ("element"=w1296:string)
                    n737 = local read "Comments"() -> (w1313:string)
                    n738 = local read "ProjectID"() -> (w1310:string)
                    n739 = Bundle("element"=w1303, "element"=w1302, "grainSize"=w1292, "element"=w1301, "barrelLength"=w1297, w1299, "element"="1", "element"=w1296, "element"=w1300) -> (w1304:T38)  [unwired: 1 out]
                    n740 = local read "lastSamp"() -> (w1318:i32)
                    n741 = control-ref of="TestStandards"() -> (w1317:refnum<vi>)
                    n742 = control-ref of="Methods"() -> (w1316:refnum<vi>)
                    n743 = Cluster To Array(cluster=w1304) -> (array=w1294:string[])
                    n744 = call "Dropdown Selection (SubVI).vi"("reference"=w1317) -> ("element"=w1312:string)
                    n745 = call "Dropdown Selection (SubVI).vi"("reference"=w1316) -> ("element"=w1315:string)
                    n746 = Increment(x=w1318) -> (x+1=w1314:i32)
                  }
                  frame "SPR0" {
                    w1319 = "" ("projNum")
                    # "THREAT"
                    # "Project Name goes here.\nSupports a PB reporting requirement."
                    # "GENERAL"
                    n747 = local read "threatDetails"() -> (w1321:T1)
                    n748 = Unbundle By Name(w1321) -> ("barrelLength"=w1324:string)
                    n749 = Unbundle By Name(w1321) -> ("grainSize"=w1320:string)
                    n750 = local read "Shot Angle"() -> (w1325:u16)
                    n751 = control-ref of="ThreatGroups"() -> (w1331:refnum<vi>)
                    n752 = control-ref of="PowderTypes"() -> (w1330:refnum<vi>)
                    n753 = control-ref of="Ballisticians"() -> (w1332:refnum<vi>)
                    n754 = Format Into String(w1325) -> (resulting string=w1326:string)  [unwired: 3 in, 1 out]
                    n755 = call "Dropdown Selection (SubVI).vi"("reference"=w1331) -> ("element"=w1328:string)
                    n756 = call "Dropdown Selection (SubVI).vi"("reference"=w1330) -> ("element"=w1327:string)
                    n757 = call "Dropdown Selection (SubVI).vi"("reference"=w1332) -> ("element"=w1323:string)
                    n758 = local read "Comments"() -> (w1334:string)
                    n759 = local read "ProjectID"() -> (w1333:string)
                    n760 = Bundle("element"=w1328, "grainSize"=w1320, "element"=w1327, "barrelLength"=w1324, w1326, "element"=w1323) -> (w1329:T39)  [unwired: 1 out]
                    n761 = local read "lastSamp"() -> (w1338:i32)
                    n762 = control-ref of="Methods"() -> (w1337:refnum<vi>)
                    n763 = Cluster To Array(cluster=w1329) -> (array=w1322:string[])
                    n764 = call "Dropdown Selection (SubVI).vi"("reference"=w1337) -> ("element"=w1336:string)
                    n765 = Increment(x=w1338) -> (x+1=w1335:i32)
                  }
                  frame "SPR1" {
                    w1339 = "" ("projNum")
                    # "THREAT"
                    # "Project Name goes here.\nSupports a PB reporting requirement."
                    # "GENERAL"
                    n766 = local read "threatDetails"() -> (w1341:T1)
                    n767 = Unbundle By Name(w1341) -> ("barrelLength"=w1344:string)
                    n768 = Unbundle By Name(w1341) -> ("grainSize"=w1340:string)
                    n769 = local read "Shot Angle"() -> (w1345:u16)
                    n770 = control-ref of="Ballisticians"() -> (w1352:refnum<vi>)
                    n771 = control-ref of="ThreatGroups"() -> (w1351:refnum<vi>)
                    n772 = control-ref of="PowderTypes"() -> (w1350:refnum<vi>)
                    n773 = call "Dropdown Selection (SubVI).vi"("reference"=w1352) -> ("element"=w1343:string)
                    n774 = call "Dropdown Selection (SubVI).vi"("reference"=w1351) -> ("element"=w1348:string)
                    n775 = call "Dropdown Selection (SubVI).vi"("reference"=w1350) -> ("element"=w1347:string)
                    n776 = Format Into String(w1345) -> (resulting string=w1346:string)  [unwired: 3 in, 1 out]
                    n777 = control-ref of="Methods"() -> (w1357:refnum<vi>)
                    n778 = local read "Comments"() -> (w1354:string)
                    n779 = local read "lastSamp"() -> (w1358:i32)
                    n780 = local read "ProjectID"() -> (w1353:string)
                    n781 = Bundle("element"=w1348, "grainSize"=w1340, "element"=w1347, "barrelLength"=w1344, w1346, "element"=w1343) -> (w1349:T39)  [unwired: 1 out]
                    n782 = call "Dropdown Selection (SubVI).vi"("reference"=w1357) -> ("element"=w1356:string)
                    n783 = Cluster To Array(cluster=w1349) -> (array=w1342:string[])
                    n784 = Increment(x=w1358) -> (x+1=w1355:i32)
                  }
                  frame "BRZ" {
                    w1359 = "" ("projNum")
                    # "THREAT"
                    # "Project Name goes here.\nSupports a PB reporting requirement."
                    # "GENERAL"
                    n785 = local read "threatDetails"() -> (w1361:T1)
                    n786 = Unbundle By Name(w1361) -> ("barrelLength"=w1364:string)
                    n787 = Unbundle By Name(w1361) -> ("grainSize"=w1360:string)
                    n788 = local read "Shot Angle"() -> (w1365:u16)
                    n789 = control-ref of="Ballisticians"() -> (w1372:refnum<vi>)
                    n790 = control-ref of="ThreatGroups"() -> (w1371:refnum<vi>)
                    n791 = control-ref of="PowderTypes"() -> (w1370:refnum<vi>)
                    n792 = call "Dropdown Selection (SubVI).vi"("reference"=w1372) -> ("element"=w1363:string)
                    n793 = call "Dropdown Selection (SubVI).vi"("reference"=w1371) -> ("element"=w1368:string)
                    n794 = call "Dropdown Selection (SubVI).vi"("reference"=w1370) -> ("element"=w1367:string)
                    n795 = Format Into String(w1365) -> (resulting string=w1366:string)  [unwired: 3 in, 1 out]
                    n796 = control-ref of="Methods"() -> (w1377:refnum<vi>)
                    n797 = local read "Comments"() -> (w1374:string)
                    n798 = local read "lastSamp"() -> (w1378:i32)
                    n799 = local read "ProjectID"() -> (w1373:string)
                    n800 = Bundle("element"=w1368, "grainSize"=w1360, "element"=w1367, "barrelLength"=w1364, w1366, "element"=w1363) -> (w1369:T39)  [unwired: 1 out]
                    n801 = call "Dropdown Selection (SubVI).vi"("reference"=w1377) -> ("element"=w1376:string)
                    n802 = Cluster To Array(cluster=w1369) -> (array=w1362:string[])
                    n803 = Increment(x=w1378) -> (x+1=w1375:i32)
                  }
                }
              }
            }
            n804 = Get Date/Time String() -> (date string=w870:string)  [unwired: 3 in, 1 out]
          }
          frame True {
            w1394 = ""
            w1386 = 16  # dimensions
            w1389 = 5  # SampleID
            # "date"
            # "method"
            # "general"
            # "remark"
            # "threat"
            # "shots"
            # "sample"
            # "results"
            # "range"
            # "fabric"
            # "query db with the entered record number and use result to populate the xlt"
            n805 = Not(x=w1452) -> (.not. x?=w1451:bool)
            n806 = local write "lookupRec"(w1451) -> ()
            n807 = Format Into String(format string="SELECT * FROM Experiments\nWHERE expt=%d;" ("query string"), error in=w1418, "Record #") -> (resulting string=w1448:string, error out=w1419:errorcluster)  [unwired: 1 in]
            n808 = call "Fetch Data (SubVI).vi"("error IN"=w1419, "query string"=w1448) -> ("error OUT"=w1417:errorcluster, "recordset data"=w1450:string[][])  [unwired: 4 out]
            n809 = Index Array(array=w1450) -> (element=w1388:string[])  [unwired: 2 in]
            n810 = Index Array(array=w1388, index=111) -> (element=w1421:string)
            n811 = local read "Set#1 Separation"() -> (w1435:sgl)
            n812 = call "Load Shots (SubVI).vi"("Record #"="Record #", "Method"=w1421) -> ("Shot Array"=w1443:string[][], "AvgDef"=w1426:dbl)  [unwired: 1 in]
            n813 = local read "mid_to_targ_dist"() -> (w1438:sgl)
            n814 = local read "Barrel to Screen"() -> (w1441:sgl)
            n815 = Format Into String(w1426) -> (resulting string=w1424:string)  [unwired: 3 in, 1 out]
            n816 = Match Pattern(string=w1421, regular expression="N.I.J.") -> (offset past match=w1423:i32)  [unwired: 4 out]
            n817 = Greater Or Equal To 0?(x=w1423) -> (x >= 0?=w1420:bool)
            n818 = case shown="False" w1420 {
              tunnel: [w1463 w1464] -> w1425
              tunnel: w1424 -> [w1460 w1466]
              tunnel: w1388 -> [w1462 _]
              frame False {
                n819 = Index Array(array=w1462, index #1=124 ("index"), index #2=149 ("index"), index #5=145 ("index")) -> (element #1=w1461:string, element #2=w1459:string, element #3=w1458:string, element #4=w1454:string, element #5=w1455:string)  [unwired: 2 in]
                n820 = Build Array(w1461, w1459, w1458, w1454, w1455, w1460) -> (w1463:string[])
              }
              frame True {
                w1465 = "" ("Empty String Constant")
                n821 = Build Array(w1465, w1465, w1465, w1465, w1465, w1466, w1466) -> (w1464:string[])
              }
            }
            n822 = Divide(x=w1435, y=sgl 2.0) -> (x/y=w1440:sgl)
            n823 = Add(x=w1441, y=w1438) -> (x+y=w1434:sgl)
            n824 = Subtract(x=w1441, y=w1440) -> (x-y=w1439:sgl)
            n825 = Subtract(x=w1438, y=w1440) -> (x-y=w1437:sgl)
            n826 = Index Array(array=w1388, index #1=120 ("index"), index #2=119 ("index"), index #3=127 ("index"), index #4=12 ("index"), index #5=7 ("index")) -> (element #1=w1406:string, element #2=w1404:string, element #3=w1403:string, element #4=w1400:string, element #5=w1399:string)
            n827 = Index Array(array=w1388, index #1=113 ("index"), index #2=112 ("index"), index #3=103 ("index")) -> (element #1=w1415:string, element #2=w1414:string, element #3=w1413:string, element #4=w1412:string, element #5=w1408:string)  [unwired: 2 in]
            n828 = Format Into String(w1434) -> (resulting string=w1433:string)  [unwired: 3 in, 1 out]
            n829 = Format Into String(w1439) -> (resulting string=w1432:string)  [unwired: 3 in, 1 out]
            n830 = Format Into String(w1435) -> (resulting string=w1431:string)  [unwired: 3 in, 1 out]
            n831 = Format Into String(w1437) -> (resulting string=w1430:string)  [unwired: 3 in, 1 out]
            n832 = Format Into String(w1438) -> (resulting string=w1429:string)  [unwired: 3 in, 1 out]
            n833 = Index Array(array=w1388, index #1=w1389, index #2=w1386, index #3=147 ("index"), index #5=148 ("index")) -> (element #1=w1387:string, element #2=w1384:string, element #3=w1383:string, element #5=w1380:string)  [unwired: 1 in, 1 out]
            n834 = Build Array(w1406, w1404, w1403, "", w1400, w1399) -> (w1405:string[])
            n835 = Build Array(w1433, w1432, w1431, w1430, w1429, w1415, w1414, w1413, w1412, w1408) -> (w1428:string[])
            n836 = Index Array(array=w1388, index #1=4 ("index"), index #2=111 ("index")) -> (element #1=w1395:string, element #2=w1392:string)
            n837 = Index Array(array=w1388, index=107) -> (element=w1444:string)
            n838 = Build Array(w1387, w1384, w1383, "", w1380) -> (w1385:string[])
            n839 = Index Array(array=w1388, index=2) -> (element=w1390:string)
            n840 = call "Get Model Construction.vi"("panel record"=w1388) -> ("Fabric Array"=w1442:string[][])
            n841 = Build Array(w1425) -> (w1445:string[][])
          }
        }
        n842 = To Variant(anything=w864) -> (Variant=w858:variant)
        n843 = To Variant(anything=w863) -> (Variant=w857:variant)
        n844 = To Variant(anything=w862) -> (Variant=w856:variant)
        n845 = To Variant(anything=w861) -> (Variant=w855:variant)
        n846 = To Variant(anything=w860) -> (Variant=w854:variant)
        n847 = To Variant(anything=w859) -> (Variant=w853:variant)
        n848 = To Variant(anything=w846) -> (Variant=w852:variant)
        n849 = To Variant(anything=w845) -> (Variant=w851:variant)
        n850 = To Variant(anything=w844) -> (Variant=w850:variant)
        n851 = To Variant(anything=w843) -> (Variant=w847:variant)
        n852 = To Variant(anything=w842) -> (Variant=w848:variant)
        n853 = To Variant(anything=w835) -> (Variant=w849:variant)
        n854 = To Variant(anything=w833) -> (Variant=w834:variant)
        n855 = call "TestReport_XL.vi"("Enable"=TRUE, "blockFabric"=w858, "blockRange"=w857, "blockResults"=w856, "blockSample"=w855, "blockShotTbl"=w854, "error in (no error)"=w838, "blockThreat"=w853, "testDate"=w834, "method"=w852, "projName"=w851, "projNum"=w850, "recNum"=w847, "remark"=w848, "standard"=w849) -> ("error out"=w865:errorcluster)  [unwired: 4 in, 8 out]
        n856 = call <vilib>:"Simple Error Handler.vi"("error in (no error)"=w865) -> ("error out"=w867:errorcluster)  [unwired: 1 in, 7 out]
        n857 = case shown="No Error" w867 {
          selector: w867 -> [w1467 w1469]
          tunnel: [w1467 w1469] -> w836
          frame No Error {
            n858 = One Button Dialog(message=" V50 Ballistic Test Report is ready") -> ()  [unwired: 2 out]
          }
          frame Error {
          }
        }
      }
      frame "VsVr Report" {
        w1499 = TRUE  # Enable
        # "case # 3"
        # "The custom Excel template file is \nexpected in the C:\\Ballistics folder."
        n859 = stacked-sequence {
          tunnel: [_ _ _ _ _ w1690] -> w1492
          tunnel: [_ w1563 _ _ _ _] -> w1496
          tunnel: [_ _ _ _ w1647 _] -> w1493
          tunnel: [_ _ _ w1614 _ _] -> w1494
          tunnel: [_ _ w1585 _ _ _] -> w1495
          tunnel: [w1507 _ _ _ _ _] -> w1497
          tunnel: [_ _ _ _ _ w1711] -> w1479
          tunnel: [_ _ _ _ _ "" ("projNum")] -> w1478
          tunnel: [_ _ _ _ _ w1706] -> w1477
          tunnel: [_ _ _ _ _ w1710] -> w1476
          tunnel: [_ _ _ _ _ w1709] -> w1475
          tunnel: [_ _ _ _ _ w1708] -> w1474
          tunnel: w1473 -> [_ _ w1584 _ w1640 _]
          frame #0 {
            # "FABRIC"
            n860 = local read "fab1_totalWt"() -> (w1510:sgl)
            n861 = local read "fab3_totalWt"() -> (w1512:sgl)
            n862 = local read "fab5_totalWt"() -> (w1514:sgl)
            n863 = global read "BIMS_Collector Globals.vi" "LayerStitchTypeRefs"() -> (w1502:refnum<vi>[])
            n864 = global read "BIMS_Collector Globals.vi" "SampleAttribs"() -> (w1503:T21)
            n865 = global read "BIMS_Collector Globals.vi" "SampleStyles"() -> (w1505:refnum<vi>[])
            n866 = local read "fab2_totalWt"() -> (w1511:sgl)
            n867 = local read "fab4_totalWt"() -> (w1513:sgl)
            n868 = local read "fab6_totalWt"() -> (w1515:sgl)
            n869 = global read "BIMS_Collector Globals.vi" "LayerSpecs"() -> (w1504:T31)
            n870 = global read "BIMS_Collector Globals.vi" "Mfrs"() -> (w1506:refnum<vi>[])
            n871 = Build Array(w1510, w1511, w1512, w1513, w1514, w1515) -> (w1509:sgl[])
            n872 = for {
              tunnel: w1509 -> [w1517] mode=indexing
              tunnel: [w1523] -> w1508 mode=indexing
              tunnel: w1503 -> [w1521] mode=indexing
              tunnel: w1504 -> [w1520] mode=indexing
              tunnel: w1506 -> [w1519] mode=indexing
              tunnel: w1505 -> [w1518] mode=indexing
              tunnel: w1502 -> [w1516] mode=indexing
              n873 = Less Or Equal To 0?(x=w1517) -> (x <= 0?=w1522:bool)
              n874 = case shown="False" w1522 {
                tunnel: [w1545 w1547] -> w1523
                tunnel: w1521 -> [w1544 _]
                tunnel: w1520 -> [w1529 _]
                tunnel: w1519 -> [w1538 _]
                tunnel: w1518 -> [w1535 _]
                tunnel: w1517 -> [w1528 _]
                tunnel: w1516 -> [w1524 _]
                frame False {
                  n875 = Unbundle By Name(w1529) -> ("numOfPlies"=w1527:i32, "LotNum"=w1541:string, "RollNum"=w1542:string)
                  n876 = Unbundle By Name(w1544) -> ("internal_ID"=w1532:string, "fiber"=w1533:string, "denier"=w1540:string, "pick"=w1539:string, "weave"=w1530:string, "finish"=w1531:string, "ozPerYd2"=w1543:string)
                  n877 = Format Into String(w1527) -> (resulting string=w1537:string)  [unwired: 3 in, 1 out]
                  n878 = call "Dropdown Selection (SubVI).vi"("reference"=w1538) -> ("element"=w1536:string)
                  n879 = call "Dropdown Selection (SubVI).vi"("reference"=w1535) -> ("element"=w1534:string)
                  n880 = call "Dropdown Selection (SubVI).vi"("reference"=w1524) -> ("element"=w1525:string)
                  n881 = Format Into String(w1528) -> (resulting string=w1526:string)  [unwired: 3 in, 1 out]
                  n882 = Build Array(w1537, w1536, w1534, w1532, w1533, w1540, w1539, w1530, w1531, w1541, w1542, w1543, w1526, w1525) -> (w1545:string[])
                }
                frame True {
                  n883 = call <vilib>:"Space Constant.vi"() -> ("String"=w1548:string)
                  n884 = Initialize Array(w1548, 12 ("dimension size")) -> (w1547:string[])
                }
              }
            }
            n885 = Transpose 2D Array(2D array=w1508) -> (transposed array=w1507:string[][])
          }
          frame #1 {
            w1549 = "%.1f" ("format string")
            # "muzzel / midpoint"
            # "muzzle / scr#1"
            # "muzzle / target"
            # "scr#2 / target"
            # "RANGE"
            n886 = local read "Set#1 Separation"() -> (w1556:sgl)
            n887 = local read "mid_to_targ_dist"() -> (w1553:sgl)
            n888 = local read "Barrel to Screen"() -> (w1550:sgl)
            n889 = local read "clayAverage"() -> (w1571:sgl)
            n890 = Divide(x=w1556, y=sgl 2.0) -> (x/y=w1551:sgl)
            n891 = local read "RoomHum"() -> (w1566:sgl)
            n892 = local read "clayTemp"() -> (w1569:sgl)
            n893 = local read "clayCalib"() -> (w1572:string)
            n894 = local read "RoomT"() -> (w1567:sgl)
            n895 = Add(x=w1550, y=w1553) -> (x+y=w1557:sgl)
            n896 = Subtract(x=w1550, y=w1551) -> (x-y=w1552:sgl)
            n897 = Subtract(x=w1553, y=w1551) -> (x-y=w1554:sgl)
            n898 = Format Into String(w1557) -> (resulting string=w1558:string)  [unwired: 3 in, 1 out]
            n899 = Format Into String(w1552) -> (resulting string=w1559:string)  [unwired: 3 in, 1 out]
            n900 = Format Into String(w1556) -> (resulting string=w1560:string)  [unwired: 3 in, 1 out]
            n901 = Format Into String(w1554) -> (resulting string=w1561:string)  [unwired: 3 in, 1 out]
            n902 = Format Into String(w1553) -> (resulting string=w1562:string)  [unwired: 3 in, 1 out]
            n903 = Format Into String(w1566) -> (resulting string=w1564:string)  [unwired: 3 in, 1 out]
            n904 = Format Into String(format string=w1549, w1567) -> (resulting string=w1565:string)  [unwired: 2 in, 1 out]
            n905 = Format Into String(format string=w1549, w1569) -> (resulting string=w1568:string)  [unwired: 2 in, 1 out]
            n906 = Format Into String(format string=w1549, w1571) -> (resulting string=w1570:string)  [unwired: 2 in, 1 out]
            n907 = Bundle(w1558, w1559, w1560, w1561, w1562, w1564, w1565, w1568, "clayCalib"=w1572, w1570) -> (w1573:T32)  [unwired: 1 out]
            n908 = Cluster To Array(cluster=w1573) -> (array=w1563:string[])
          }
          frame #2 {
            # "RESULTS"
            n909 = control-ref of="Methods"() -> (w1574:refnum<vi>)
            n910 = call "Dropdown Selection (SubVI).vi"("reference"=w1574) -> ("element"=w1575:string)
            n911 = for {
              tunnel: w1584 -> [w1612] mode=indexing
              tunnel: [w1611] -> w1583 mode=indexing
              tunnel: [w1610] -> w1582
              i -> [w1610]
              n912 = Unbundle By Name(w1612) -> ("BackFace\nDepth"=w1611:sgl)
            }
            n913 = Increment(x=w1582) -> (x+1=w1580:i32)
            n914 = Add Array Elements(numeric array=w1583) -> (sum=w1581:sgl)
            n915 = To Single Precision Float(number=w1580) -> (single precision float=w1579:sgl)
            n916 = Divide(x=w1581, y=w1579) -> (x/y=w1578:sgl)
            n917 = Format Into String(format string="%1.1f", w1578) -> (resulting string=w1577:string)  [unwired: 2 in, 1 out]
            n918 = case shown="\"V50\"" w1575 {
              tunnel: [w1600 w1609] -> w1587
              tunnel: w1577 -> [w1588 w1608]
              frame "V50" {
                w1594 = "%1d" ("format string")
                n919 = local read "Z.M.R."() -> (w1592:sgl)
                n920 = Less Than 0?(x=w1592) -> (x < 0?=w1593:bool)
                n921 = local read "rangeOfResults"() -> (w1596:i32)
                n922 = local read "computed_V50"() -> (w1599:sgl)
                n923 = local read "lowComplete"() -> (w1597:i32)
                n924 = local read "highPartial"() -> (w1598:i32)
                n925 = case shown="True" w1593 {
                  tunnel: w1592 -> [w1605 _]
                  tunnel: [w1605 sgl 0.0 ("Z.M.R.")] -> w1591
                  frame False {
                  }
                  frame True {
                  }
                }
                n926 = Format Into String(format string="%1.1f", w1599) -> (resulting string=w1603:string)  [unwired: 2 in, 1 out]
                n927 = Format Into String(format string=w1594, w1598) -> (resulting string=w1602:string)  [unwired: 2 in, 1 out]
                n928 = Format Into String(format string=w1594, w1597) -> (resulting string=w1601:string)  [unwired: 2 in, 1 out]
                n929 = Format Into String(format string=w1594, w1596) -> (resulting string=w1604:string)  [unwired: 2 in, 1 out]
                n930 = Format Into String(format string="%1.1f", w1591) -> (resulting string=w1590:string)  [unwired: 2 in, 1 out]
                n931 = Bundle(w1603, w1602, w1601, w1604, w1590, w1588, w1588) -> (w1600:T33)  [unwired: 1 out]
              }
              frame Default {
                w1607 = "" ("Empty String Constant")
                n932 = Bundle(w1607, w1607, w1607, w1607, w1607, w1608, w1608) -> (w1609:T33)  [unwired: 1 out]
              }
            }
            n933 = Cluster To Array(cluster=w1587) -> (array=w1586:string[])
            n934 = Build Array(w1586) -> (w1585:string[][])
          }
          frame #3 {
            # "PB Req"
            # "SAMPLE"
            n935 = control-ref of="Methods"() -> (w1615:refnum<vi>)
            n936 = call "Dropdown Selection (SubVI).vi"("reference"=w1615) -> ("element"=w1617:string)
            n937 = Equal?(x=w1617, y="V50") -> (x = y?=w1616:bool)
            n938 = local read "totalSampleWt"() -> (w1627:sgl)
            n939 = case shown="True" w1616 {
              tunnel: ["n/a" w1637] -> w1621
              frame False {
              }
              frame True {
                n940 = local read "minV50"() -> (w1636:i32)
                n941 = Format Into String(w1636) -> (resulting string=w1637:string)  [unwired: 3 in, 1 out]
              }
            }
            n942 = local read "Type of work"() -> (w1613:string)
            n943 = control-ref of="SampleDimensions"() -> (w1633:refnum<vi>)
            n944 = control-ref of="SampleCoverings"() -> (w1634:refnum<vi>)
            n945 = control-ref of="Models"() -> (w1620:refnum<vi>)
            n946 = local read "serialNum"() -> (w1629:string)
            n947 = local read "SampleID"() -> (w1631:string)
            n948 = local read "Thickness"() -> (w1624:dbl)
            n949 = local read "totalBAW"() -> (w1623:sgl)
            n950 = call "Dropdown Selection (SubVI).vi"("reference"=w1633) -> ("element"=w1630:string)
            n951 = call "Dropdown Selection (SubVI).vi"("reference"=w1620) -> ("element"=w1619:string)
            n952 = call "Dropdown Selection (SubVI).vi"("reference"=w1634) -> ("element"=w1628:string)
            n953 = Format Into String(w1627) -> (resulting string=w1626:string)  [unwired: 3 in, 1 out]
            n954 = Format Into String(w1624) -> (resulting string=w1625:string)  [unwired: 3 in, 1 out]
            n955 = Format Into String(w1623) -> (resulting string=w1622:string)  [unwired: 3 in, 1 out]
            n956 = Bundle("SampleID"=w1631, "element"=w1630, "Type of work"=w1613, "serialNum"=w1629, "element"=w1619, w1626, w1625, w1622, "element"=w1628, w1621) -> (w1632:T34)  [unwired: 1 out]
            n957 = Cluster To Array(cluster=w1632) -> (array=w1614:string[])
          }
          frame #4 {
            # "SHOT TABLE"
            n958 = control-ref of="Methods"() -> (w1639:refnum<vi>)
            n959 = call "Dropdown Selection (SubVI).vi"("reference"=w1639) -> ("element"=w1638:string)
            n960 = for {
              tunnel: w1640 -> [w1679] mode=indexing
              shift-right: [w1656] -> _
              shift-left: T25 [] -> [w1658]
              tunnel: [w1656] -> w1643
              tunnel: w1638 -> [w1652]
              n961 = Unbundle By Name(w1679) -> ("shot order"=w1678:i32, "Powder Loading"=w1677:sgl, "Uncorrected Impact"=w1676:sgl, "UncorrectedRed_PB"=w1675:sgl, "UncorrectedAvgVel_PB"=w1674:sgl, "velLoss_PB"=w1673:sgl, "strikeVel_PB"=w1672:sgl, "SHOT STATUS"=w1661:u16, "usedv50"=w1671:bool, "Shot Angle"=w1653:u16, "BackFace\nDepth"=w1654:sgl)
              n962 = case shown="\"V50\"" w1652 {
                tunnel: w1671 -> [w1681 _]
                tunnel: [w1680 w1685] -> w1670
                tunnel: w1653 -> [_ w1684]
                frame "V50" {
                  n963 = case shown="True" w1681 {
                    tunnel: ["" ("Empty String Constant") "*"] -> w1680
                    frame False {
                    }
                    frame True {
                    }
                  }
                }
                frame Default {
                  n964 = Format Into String(w1684) -> (resulting string=w1685:string)  [unwired: 3 in, 1 out]
                }
              }
              n965 = case shown="1" w1661 {
                tunnel: ["P" "C"] -> w1660
                frame 0, Default {
                }
                frame 1 {
                }
              }
              n966 = Format Into String(format string="%2d", w1678) -> (resulting string=w1663:string)  [unwired: 2 in, 1 out]
              n967 = Format Into String(w1677) -> (resulting string=w1664:string)  [unwired: 3 in, 1 out]
              n968 = Format Into String(w1676) -> (resulting string=w1665:string)  [unwired: 3 in, 1 out]
              n969 = Format Into String(w1675) -> (resulting string=w1666:string)  [unwired: 3 in, 1 out]
              n970 = Format Into String(w1674) -> (resulting string=w1667:string)  [unwired: 3 in, 1 out]
              n971 = Format Into String(w1673) -> (resulting string=w1668:string)  [unwired: 3 in, 1 out]
              n972 = Format Into String(w1672) -> (resulting string=w1669:string)  [unwired: 3 in, 1 out]
              n973 = Format Into String(w1654) -> (resulting string=w1662:string)  [unwired: 3 in, 1 out]
              n974 = Build Array(w1663, w1664, w1665, w1666, w1667, w1668, w1669, w1660, w1670, w1662) -> (w1657:string[])
              n975 = Array To Cluster(array=w1657) -> (cluster=w1659:T36)
              n976 = Build Array (concatenate)(w1658, w1659) -> (w1656:T25)
            }
            n977 = Array Size(array=w1643) -> (size(s)=w1645:i32)
            n978 = Equal To 0?(x=w1645) -> (x = 0?=w1641:bool)
            n979 = case shown="True" w1641 {
              tunnel: [w1648 T25 [{"[0]"="", "[1]"="", "[2]"="", "[3]"="", "[4]"="", "[5]"="", "[6]"="", "[7]"="", "[8]"="", "[9]"=""}]] -> w1642
              tunnel: w1643 -> [w1648 _]
              frame False {
              }
              frame True {
              }
            }
            n980 = Sort 1D Array(array=w1642) -> (sorted array=w1644:T25)
            n981 = for {
              tunnel: w1644 -> [w1651] mode=indexing
              tunnel: [w1650] -> w1647 mode=indexing
              n982 = Cluster To Array(cluster=w1651) -> (array=w1650:string[])
            }
          }
          frame #5 {
            # "THREAT"
            # "Range # (supports a PB reporting requirement)"
            # "Project Name goes here.\nSupports a PB reporting requirement."
            # "GENERAL"
            n983 = local read "threatDetails"() -> (w1689:T1)
            n984 = Unbundle By Name(w1689) -> ("barrelLength"=w1693:string)
            n985 = Unbundle By Name(w1689) -> ("grainSize"=w1688:string)
            n986 = local read "Shot Angle"() -> (w1694:u16)
            n987 = control-ref of="WeaponTypes"() -> (w1703:refnum<vi>)
            n988 = control-ref of="ThreatGroups"() -> (w1702:refnum<vi>)
            n989 = control-ref of="PowderTypes"() -> (w1701:refnum<vi>)
            n990 = control-ref of="Recorders"() -> (w1704:refnum<vi>)
            n991 = control-ref of="Shooters"() -> (w1705:refnum<vi>)
            n992 = Format Into String(w1694) -> (resulting string=w1695:string)  [unwired: 3 in, 1 out]
            n993 = call "Dropdown Selection (SubVI).vi"("reference"=w1703) -> ("element"=w1699:string)
            n994 = call "Dropdown Selection (SubVI).vi"("reference"=w1702) -> ("element"=w1698:string)
            n995 = call "Dropdown Selection (SubVI).vi"("reference"=w1701) -> ("element"=w1697:string)
            n996 = call "Dropdown Selection (SubVI).vi"("reference"=w1704) -> ("element"=w1696:string)
            n997 = call "Dropdown Selection (SubVI).vi"("reference"=w1705) -> ("element"=w1692:string)
            n998 = Bundle("element"=w1699, "element"=w1698, "grainSize"=w1688, "element"=w1697, "barrelLength"=w1693, w1695, "element"="1", "element"=w1692, "element"=w1696) -> (w1700:T38)  [unwired: 1 out]
            n999 = Cluster To Array(cluster=w1700) -> (array=w1690:string[])
            n1000 = local read "Comments"() -> (w1709:string)
            n1001 = local read "ProjectID"() -> (w1706:string)
            n1002 = local read "lastSamp"() -> (w1714:i32)
            n1003 = control-ref of="TestStandards"() -> (w1713:refnum<vi>)
            n1004 = control-ref of="Methods"() -> (w1712:refnum<vi>)
            n1005 = call "Dropdown Selection (SubVI).vi"("reference"=w1713) -> ("element"=w1708:string)
            n1006 = call "Dropdown Selection (SubVI).vi"("reference"=w1712) -> ("element"=w1711:string)
            n1007 = Increment(x=w1714) -> (x+1=w1710:i32)
          }
        }
        n1008 = To Variant(anything=w1497) -> (Variant=w1491:variant)
        n1009 = To Variant(anything=w1496) -> (Variant=w1490:variant)
        n1010 = To Variant(anything=w1495) -> (Variant=w1489:variant)
        n1011 = To Variant(anything=w1494) -> (Variant=w1488:variant)
        n1012 = To Variant(anything=w1493) -> (Variant=w1487:variant)
        n1013 = To Variant(anything=w1492) -> (Variant=w1486:variant)
        n1014 = To Variant(anything=w1479) -> (Variant=w1485:variant)
        n1015 = To Variant(anything=w1478) -> (Variant=w1484:variant)
        n1016 = To Variant(anything=w1477) -> (Variant=w1483:variant)
        n1017 = To Variant(anything=w1476) -> (Variant=w1480:variant)
        n1018 = To Variant(anything=w1475) -> (Variant=w1481:variant)
        n1019 = To Variant(anything=w1474) -> (Variant=w1482:variant)
        n1020 = call "TestReport_XL.vi"("Enable"=w1499, "blockFabric"=w1491, "blockRange"=w1490, "blockResults"=w1489, "blockSample"=w1488, "blockShotTbl"=w1487, "error in (no error)"=w1471, "blockThreat"=w1486, "method"=w1485, "projName"=w1484, "projNum"=w1483, "recNum"=w1480, "remark"=w1481, "standard"=w1482) -> ("error out"=w1498:errorcluster)  [unwired: 5 in, 8 out]
        n1021 = call <vilib>:"Simple Error Handler.vi"("error in (no error)"=w1498) -> ("error out"=w1500:errorcluster)  [unwired: 1 in, 7 out]
        n1022 = case shown="No Error" w1500 {
          selector: w1500 -> [w1715 w1717]
          tunnel: [w1715 w1717] -> w1470
          frame No Error {
            n1023 = One Button Dialog(message=" VsVr Ballistic Test Report is ready") -> ()  [unwired: 2 out]
          }
          frame Error {
          }
        }
      }
      frame "SAVE SHOTS" {
        # "case # 4"
        # "This section saves the shots to the data base"
        n1024 = stacked-sequence {
          seq-local: [w1760 _ _] -> [_ w1846 _]
          seq-local: [w1762 _ _] -> [_ w1843 _]
          seq-local: [_ w1831 _] -> [_ _ w1860]
          seq-local: [_ w1833 _] -> [_ _ w1859]
          seq-local: [w1758 _ _] -> [_ _ w1852]
          seq-local: [w1732 _ _] -> [_ w1789 _]
          tunnel: [_ _ w1854] -> w1722
          tunnel: [_ _ w1857] -> w1723
          tunnel: w1719 -> [_ w1798 w1851]
          tunnel: w1721 -> [w1734 _ _]
          frame #0 {
            # "Legacy requirements:"
            # "Shared requirements:"
            n1025 = local read "fab1_totalWt"() -> (w1770:sgl)
            n1026 = local read "fab2_totalWt"() -> (w1769:sgl)
            n1027 = local read "fab3_totalWt"() -> (w1768:sgl)
            n1028 = local read "fab4_totalWt"() -> (w1767:sgl)
            n1029 = local read "fab5_totalWt"() -> (w1766:sgl)
            n1030 = local read "fab6_totalWt"() -> (w1765:sgl)
            n1031 = Build Array(w1770, w1769, w1768, w1767, w1766, w1765) -> (w1764:sgl[])
            n1032 = call "SQL Statement for Sample Descritpion.vi"("error IN"=w1734, "Layer Weight Array"=w1764, "VALUES clause IN"=" VALUES (%d " ("SQL statement IN"), "INSERT clause IN"="INSERT INTO Experiments " ("SQL statement IN")) -> ("error OUT"=w1733:errorcluster, "VALUES clause OUT"=w1763:string, "INSERT clause OUT"=w1761:string)  [unwired: 1 out]
            n1033 = local read "lastSamp"() -> (w1759:i32)
            n1034 = Increment(x=w1759) -> (x+1=w1758:i32)
            n1035 = local read "rangeOfResults"() -> (w1736:i32)
            n1036 = local read "lowComplete"() -> (w1737:i32)
            n1037 = local read "clayAverage"() -> (w1739:sgl)
            n1038 = local read "highPartial"() -> (w1738:i32)
            n1039 = control-ref of="SampleClamping"() -> (w1731:refnum<vi>)
            n1040 = control-ref of="BackLayer"() -> (w1729:refnum<vi>)
            n1041 = control-ref of="FrontLayer"() -> (w1728:refnum<vi>)
            n1042 = control-ref of="Ballisticians"() -> (w1753:refnum<vi>)
            n1043 = control-ref of="Shooters"() -> (w1749:refnum<vi>)
            n1044 = control-ref of="Recorders"() -> (w1748:refnum<vi>)
            n1045 = control-ref of="Submitters"() -> (w1752:refnum<vi>)
            n1046 = control-ref of="SampleCoverings"() -> (w1745:refnum<vi>)
            n1047 = control-ref of="ThreatGroups"() -> (w1744:refnum<vi>)
            n1048 = call "Dropdown Selection (SubVI).vi"("reference"=w1753) -> ("element"=w1751:string)
            n1049 = call "Dropdown Selection (SubVI).vi"("reference"=w1749) -> ("element"=w1747:string)
            n1050 = call "Dropdown Selection (SubVI).vi"("reference"=w1748) -> ("element"=w1746:string)
            n1051 = call "Dropdown Selection (SubVI).vi"("reference"=w1752) -> ("element"=w1750:string)
            n1052 = call "Dropdown Selection (SubVI).vi"("reference"=w1745) -> ("element"=w1743:string)
            n1053 = call "Dropdown Selection (SubVI).vi"("reference"=w1744) -> ("element"=w1742:string)
            n1054 = call "Dropdown Selection (SubVI).vi"("reference"=w1731) -> ("element"=w1730:string)
            n1055 = call "Dropdown Selection (SubVI).vi"("reference"=w1729) -> ("element"=w1727:string)
            n1056 = call "Dropdown Selection (SubVI).vi"("reference"=w1728) -> ("element"=w1726:string)
            n1057 = Format Into String(format string=", %d, #%s#, '%s', '%s', '%s', '%s', '%s', '%s', %.1f, '%s', %.1f, %d, %d, %d, '%s', '%s', '%s'" ("Format String"), initial string=w1763, error in=w1733, w1758, "shotTimestamp", w1751, w1747, w1746, w1750, w1743, w1742, "clayTemp", "clayCalib", w1739, w1738, w1737, w1736, w1730, w1727, w1726) -> (resulting string=w1762:string, error out=w1732:errorcluster)
            n1058 = Concatenate Strings(w1761, ", expt, [date], Ballistician1, Ballistician2, Ballistician3, Submitter1, SampleCovering, ProjectileType, ClayTemp, ClayCalibration, ClayAvgThickness, highPartial, lowComplete, rangeOfResults, clamping, FrontPly, BackPly," ("Substring")) -> (w1760:string)
            n1059 = flat-sequence {
              tunnel: ["TestStandards"] -> _
              tunnel: ["Shooters"] -> _
              tunnel: ["Recorders"] -> _
              tunnel: ["WeaponTypes"] -> _
              tunnel: ["Models"] -> _
              tunnel: ["serialNum"] -> _
              tunnel: ["layerStitch_1"] -> _
              tunnel: ["layerStitch_2"] -> _
              tunnel: ["layerStitch_3"] -> _
              tunnel: ["layerStitch_4"] -> _
              tunnel: ["layerStitch_5"] -> _
              tunnel: ["layerStitch_6"] -> _
              tunnel: ["minV50"] -> _
              frame #0 {
                # "PB-only requirements:"
              }
            }
          }
          frame #1 {
            w1845 = " Angle, Conditions, SampleType, ThreatGrain, ThreatDetail, V50dc, V50, maker, thickness, powder, numshots, backing, totalnumberplys, testcomments, NIJ1, method, temperature, humidity, Dimensions, zmr, ProjectID, SampleID, panelmaker, panelWeight, totalBAW)"  # INSERT clause continued
            # "Although shot angle is defined for the overall\nexperiment, it is also recorded for each shot."
            n1060 = local read "computed_V50"() -> (w1841:sgl)
            n1061 = local read "Drag Corrected"() -> (w1836:bool)
            n1062 = local read "Impact factor"() -> (w1838:sgl)
            n1063 = Array Size(array=w1798) -> (size(s)=w1829:i32)
            n1064 = Select(t=w1838, s=w1836, f=sgl 1.0) -> (s? t:f=w1837:sgl)
            n1065 = Divide(x=w1841, y=w1837) -> (x/y=w1840:sgl)
            n1066 = control-ref of="ModelMfrs"() -> (w1824:refnum<vi>)
            n1067 = control-ref of="PowderTypes"() -> (w1822:refnum<vi>)
            n1068 = call "Dropdown Selection (SubVI).vi"("reference"=w1824) -> ("element"=w1823:string)
            n1069 = call "Dropdown Selection (SubVI).vi"("reference"=w1822) -> ("element"=w1806:string)
            n1070 = local read "GrainSize"() -> (w1787:u16)
            n1071 = local read "Z.M.R."() -> (w1812:sgl)
            n1072 = local read "Shot Angle"() -> (w1800:u16)
            n1073 = Less Than 0?(x=w1812) -> (x < 0?=w1811:bool)
            n1074 = local read "totalNumLayers"() -> (w1828:i32)
            n1075 = control-ref of="ThreatDetails"() -> (w1784:refnum<vi>)
            n1076 = control-ref of="SampleTypes"() -> (w1794:refnum<vi>)
            n1077 = control-ref of="TestConditions"() -> (w1813:refnum<vi>)
            n1078 = control-ref of="SampleBackings"() -> (w1821:refnum<vi>)
            n1079 = Format Into String(w1787) -> (resulting string=w1786:string)  [unwired: 3 in, 1 out]
            n1080 = local read "totalBAW"() -> (w1814:sgl)
            n1081 = case shown="True" w1811 {
              tunnel: w1812 -> [w1849 _]
              tunnel: [w1849 sgl 0.0 ("Z.M.R.")] -> w1810
              frame False {
              }
              frame True {
              }
            }
            n1082 = control-ref of="SampleDimensions"() -> (w1817:refnum<vi>)
            n1083 = control-ref of="N.I.J"() -> (w1819:refnum<vi>)
            n1084 = control-ref of="Methods"() -> (w1804:refnum<vi>)
            n1085 = control-ref of="Assemblers"() -> (w1815:refnum<vi>)
            n1086 = call "Dropdown Selection (SubVI).vi"("reference"=w1784) -> ("element"=w1785:string)
            n1087 = call "Dropdown Selection (SubVI).vi"("reference"=w1794) -> ("element"=w1793:string)
            n1088 = call "Dropdown Selection (SubVI).vi"("reference"=w1813) -> ("element"=w1799:string)
            n1089 = call "Dropdown Selection (SubVI).vi"("reference"=w1821) -> ("element"=w1820:string)
            n1090 = Equal?(x=w1786, y="") -> (x = y?=w1808:bool)
            n1091 = call "Dropdown Selection (SubVI).vi"("reference"=w1819) -> ("element"=w1818:string)
            n1092 = call "Dropdown Selection (SubVI).vi"("reference"=w1804) -> ("element"=w1803:string)
            n1093 = call "Dropdown Selection (SubVI).vi"("reference"=w1817) -> ("element"=w1816:string)
            n1094 = call "Dropdown Selection (SubVI).vi"("reference"=w1815) -> ("element"=w1805:string)
            n1095 = case shown="False" w1808 {
              tunnel: [w1847 "0" ("element")] -> w1807
              tunnel: w1786 -> [w1847 _]
              frame False {
              }
              frame True {
              }
            }
            n1096 = call "Prepare DB Connect Path (SubVI).vi"("connectString"=path "BIMS_Collector.udl", "error in"=w1789) -> ("appended path"=w1788:path, "error out"=w1790:errorcluster)  [unwired: 1 out]
            n1097 = Format Into String(format string=", %d, '%s', '%s', '%s', '%s', %.4f, %.1f, '%s', %.4f, '%s', %d, '%s', %d, '%s', '%s', '%s', %.1f, %.1f, '%s', %.1f, '%s', '%s', '%s', %.1f, %.1f);" ("Format String"), initial string=w1843, error in=w1790, w1800, w1799, w1793, w1807, w1785, w1841, w1840, w1823, "Thickness", w1806, w1829, w1820, w1828, "Comments", w1818, w1803, "RoomT", "RoomHum", w1816, w1810, "ProjectID", "SampleID", w1805, "totalSampleWt", w1814) -> (resulting string=w1842:string, error out=w1792:errorcluster)
            n1098 = call-poly <vilib>:"DB Tools Open Connection.vi"("error in (no error)"=w1792, "connection information"=w1788) -> ("error out"=w1801:errorcluster, "connection reference"=w1802:T40)  [unwired: 3 in, 3 out]
            n1099 = Concatenate Strings(w1846, w1845, w1842) -> (w1835:string)
            n1100 = call-poly <vilib>:"DB Tools Execute Query.vi"("error in (no error)"=w1801, "SQL query"=w1835, "connection reference"=w1802) -> ("error out"=w1834:errorcluster, "recordset reference"=w1832:T41)  [unwired: 1 in, 4 out]
            n1101 = call-poly <vilib>:"DB Tools Free Object.vi"("error in (no error)"=w1834, "recordset reference"=w1832) -> ("error out"=w1833:errorcluster, "connection reference"=w1831:T40)  [unwired: 8 out]
          }
          frame #2 {
            # "Experiment.expt"
            n1102 = local read "lastShot"() -> (w1858:i32)
            n1103 = Increment(x=w1858) -> (x+1=w1856:i32)
            n1104 = for {
              tunnel: w1851 -> [w1904] mode=indexing
              tunnel: w1860 -> [w1879]
              tunnel: w1859 -> [w1863]
              tunnel: [w1877] -> w1853
              tunnel: [w1878] -> w1855
              tunnel: w1856 -> [w1884]
              tunnel: [w1876] -> w1857
              tunnel: w1852 -> [w1872]
              i -> [w1876]
              w1864 = sgl 1.0 ("f")
              # "Shot.id"
              n1105 = Add(x=w1884, y=w1876) -> (x+y=w1883:i32)
              n1106 = Unbundle By Name(w1904) -> ("IMPACT VELOCITY"=w1890:sgl, "Redundant_Velocity"=w1869:sgl, "RESIDUAL  VELOCITY"=w1868:sgl, "Shot Description"=w1870:string, "Powder Loading"=w1894:sgl, "Barrel Temperature"=w1895:sgl, "TIME / DATE"=w1896:string, "shot order"=w1897:i32, "Shot Angle"=w1898:u16, "BackFace\nDepth"=w1899:sgl, "BackFace\nDiameter"=w1900:sgl, "SHOT STATUS"=w1902:u16, "Projectile Mass"=w1893:sgl, "usedv50"=w1892:bool, "Energy Loss (J)"=w1891:sgl, "avgVel_PB"=w1875:sgl, "velLoss_PB"=w1874:sgl, "strikeVel_PB"=w1873:sgl, "Frag Rod"=w1861:sgl)
              n1107 = local read "Drag Corrected"() -> (w1866:bool)
              n1108 = local read "Residual factor"() -> (w1888:sgl)
              n1109 = local read "Impact factor"() -> (w1865:sgl)
              n1110 = Select(t=w1865, s=w1866, f=w1864) -> (s? t:f=w1886:sgl)
              n1111 = Select(t=w1865, s=w1866, f=w1864) -> (s? t:f=w1871:sgl)
              n1112 = Select(t=w1888, s=w1866, f=w1864) -> (s? t:f=w1887:sgl)
              n1113 = Divide(x=w1890, y=w1886) -> (x/y=w1885:sgl)
              n1114 = Divide(x=w1869, y=w1871) -> (x/y=w1867:sgl)
              n1115 = Divide(x=w1868, y=w1887) -> (x/y=w1889:sgl)
              n1116 = Greater Than 0?(x=w1902) -> (x > 0?=w1901:bool)
              n1117 = Format Into String(format string="INSERT INTO shots (impactdc, redundantdc, residualdc,  comment, loading, barreltemp, [date], [order], shotangle, bfdepth, bfdiameter, [complete], expt, id, weight,usedv50, loss, residual, impact, redundant, avgVel_PB, velLoss_PB, strikeVel_PB, fragRod)  VALUES (%.1f, %.1f, %.1f, '%s', %.4f, %.1f, #%s#, %d, %d, %.3f, %.3f, %d, %d, %d, %.4f, %d, %.4f, %.1f, %.1f, %.1f, %.1f, %.1f, %.1f, %.1f)" ("Substring"), error in=w1863, w1890, w1869, w1868, w1870, w1894, w1895, w1896, w1897, w1898, w1899, w1900, w1901, w1872, w1883, w1893, w1892, w1891, w1889, w1885, w1867, w1875, w1874, w1873, w1861) -> (resulting string=w1880:string, error out=w1862:errorcluster)  [unwired: 1 in]
              n1118 = call-poly <vilib>:"DB Tools Execute Query.vi"("error in (no error)"=w1862, "SQL query"=w1880, "connection reference"=w1879) -> ("error out"=w1882:errorcluster, "recordset reference"=w1881:T41)  [unwired: 1 in, 4 out]
              n1119 = call-poly <vilib>:"DB Tools Free Object.vi"("error in (no error)"=w1882, "recordset reference"=w1881) -> ("error out"=w1877:errorcluster, "connection reference"=w1878:T40)  [unwired: 8 out]
            }
            n1120 = call <vilib>:"DB Tools Close Connection.vi"("error in (no error)"=w1853, "connection reference"=w1855) -> ("error out"=w1854:errorcluster)  [unwired: 5 out]
          }
        }
        n1121 = case shown="No Error" w1722 {
          selector: w1722 -> [w1916 w1935]
          tunnel: [-1 -1] -> w1724
          tunnel: [Collector_State."POLL" ("progState") Collector_State."POLL" ("progState")] -> w1725
          tunnel: w1723 -> [w1919 _]
          tunnel: [w1912 w1933] -> w1720
          tunnel: w1719 -> [w1911 w1932]
          tunnel: [w1909 w1932] -> w1718
          frame No Error {
            n1122 = local read "lastSamp"() -> (w1918:i32)
            n1123 = local read "configPath"() -> (w1906:path)
            n1124 = local read "lastShot"() -> (w1920:i32)
            n1125 = flat-sequence {
              tunnel: w1912 -> [_]
              tunnel: w1908 -> [w1930]
              tunnel: [w1930] -> w1909
              frame #0 {
                w1923 = T15."Disabled and Grayed Out" ("Disabled")
                n1126 = property on="saveReq" class="Str"("Visible"=TRUE) -> ()  [unwired: 2 in, 2 out]
                n1127 = local write "SampleID"("") -> ()
                n1128 = property on="clearShots" class="Bool"("Disabled"=T15."Enabled") -> ()  [unwired: 2 in, 2 out]
                n1129 = property on="addShot" class="Bool"("Disabled"=w1923) -> ()  [unwired: 2 in, 2 out]
                n1130 = property on="undoLastShot" class="Bool"("Disabled"=w1923) -> ()  [unwired: 2 in, 2 out]
                n1131 = property on="saveShots" class="Bool"("Disabled"=w1923) -> ()  [unwired: 2 in, 2 out]
                n1132 = property on="mainTabCntrl" class="TabCtl (strict)"("Val(Sgnl)"=enum32{"Setup", "Measure", "History", "System"}."Setup" ("mainTabCntrl")) -> ()  [unwired: 2 in, 2 out]
                n1133 = One Button Dialog(message="Data Saved. Enter new Sample ID.") -> ()  [unwired: 1 in, 1 out]
                n1134 = property on="SampleEntryTabCntrl" class="TabCtl (strict)"("Value"=enum32{"Environment", "Sample"}."Sample" ("SampleEntryTabCntrl")) -> ()  [unwired: 2 in, 2 out]
                n1135 = property on="Sample SubTabCntrl" class="TabCtl (strict)"("Value"=T2."General Specification" ("Sample SubTabCntrl")) -> ()  [unwired: 2 in, 2 out]
              }
            }
            n1136 = Array Size(array=w1911) -> (size(s)=w1910:i32)
            n1137 = Increment(x=w1920) -> (x+1=w1917:i32)
            n1138 = for {
              N: w1910 -> [_]
              shift-right: [w1921] -> w1908
              shift-left: w1911 -> [w1922]
              n1139 = Delete From Array(array=w1922) -> (array with subset deleted=w1921:T6)  [unwired: 2 in, 1 out]
            }
            n1140 = Add(x=w1917, y=w1919) -> (x+y=w1907:i32)
            n1141 = Increment(x=w1918) -> (x+1=w1905:i32)
            n1142 = local write "lastShot"(w1907) -> ()
            n1143 = call "save stats to INI (SubVI).vi"("lastSamp"=w1905, "errIN"=w1916, "lastShot"=w1907, "configPath"=w1906) -> ("errOUT"=w1912:errorcluster, "recordNum"=w1915:dbl)  [unwired: 6 in]
            n1144 = property on="Record #" class="DigNum (strict)"("Maximum"=w1915) -> ()  [unwired: 2 in, 2 out]
            n1145 = local write "lastSamp"(w1905) -> ()
            n1146 = property on="shotsArr" class="Arr (strict)"("Val(Sgnl)"=w1908) -> ()  [unwired: 2 in, 2 out]
          }
          frame Error {
            n1147 = One Button Dialog(message="Error saving Data. ") -> ()  [unwired: 2 out]
            n1148 = call <vilib>:"General Error Handler.vi"("error in (no error)"=w1935) -> ("error out"=w1933:errorcluster)  [unwired: 2 in, 12 out]
          }
        }
      }
      frame "ADD SHOT" {
        # "case # 5"
        # "Shot Order"
        # "This section accepts new data to the shot table."
        n1149 = local read "Impact/speed"() -> (w1975:sgl)
        n1150 = local read "residual/speed"() -> (w1971:sgl)
        n1151 = property on="undoLastShot" class="Bool"(error in=w1950, "Disabled"=T15."Enabled") -> (error out=w1949:errorcluster)  [unwired: 1 in, 1 out]
        n1152 = local read "Current/residual/speed"() -> (w1960:sgl)
        n1153 = local read "CorrectedVelScrnSet1"() -> (w1961:sgl)
        n1154 = local read "CorrectedVelScrnSet2"() -> (w1980:sgl)
        n1155 = local read "Current/avg/speed"() -> (w1982:sgl)
        n1156 = local read "Corrected Residual"() -> (w1959:sgl)
        n1157 = local read "Redundant/speed"() -> (w1979:sgl)
        n1158 = local read "conversion factor"() -> (w1969:sgl)
        n1159 = local read "MeasVelScrnSet1"() -> (w1978:sgl)
        n1160 = local read "MeasVelScrnSet2"() -> (w1977:sgl)
        n1161 = local read "Projectile Mass"() -> (w1951:sgl)
        n1162 = case shown="\"grains\"" "loadingUnits" {
          tunnel: [w1988 w1989] -> w1945
          tunnel: "Powder Loading" -> [w1988 w1990]
          frame "grams", Default {
            # "Always save in grams."
          }
          frame "grains" {
            # "Always save in grams."
            n1163 = Multiply(x=w1990, y=sgl 0.06479891) -> (x*y=w1989:sgl)
          }
        }
        n1164 = local read "Avg/speed"() -> (w1981:sgl)
        n1165 = Array Size(array=w1954) -> (size(s)=w1957:i32)
        n1166 = Multiply(x=w1975, y=w1969) -> (x*y=w1967:sgl)
        n1167 = Multiply(x=w1969, y=w1971) -> (x*y=w1968:sgl)
        n1168 = Increment(x=w1957) -> (x+1=w1976:i32)
        n1169 = Multiply(x=w1967, y=w1967) -> (x*y=w1963:sgl)
        n1170 = Multiply(x=w1968, y=w1968) -> (x*y=w1964:sgl)
        n1171 = Subtract(x=w1963, y=w1964) -> (x-y=w1965:sgl)
        n1172 = Compound Arithmetic op=MULTIPLY(w1951, w1965, sgl 0.0005 ("Input")) -> (w1970:sgl)
        n1173 = Format Date/Time String(time format string (%c)="%x   %H:%M:%S") -> (date/time string=w1972:string)  [unwired: 2 out]
        "SUBMIT DATE/TIME" <- w1972
        n1174 = Index Array(array=w1954) -> (element=w1956:T7)  [unwired: 1 in]
        n1175 = Bundle By Name(cluster=w1956, "TIME / DATE"=w1972, "shot order"=w1976, "IMPACT VELOCITY"=w1975, "RESIDUAL  VELOCITY"=w1971, "Shot Description"="Shot Description", "Powder Loading"=w1945, "Barrel Temperature"="Barrel Temp", "SHOT STATUS"="Current/shotstatus", "BackFace\nDepth"="backdepth", "Shot Angle"="Shot Angle", "Uncorrected Impact"=w1978, "Corrected Impact"=w1961, "Uncorrected Residual"=w1960, "Corrected residual"=w1959, "Projectile Mass"=w1951, "Energy Loss (J)"=w1970, "UncorrectedRed_PB"=w1977, "Redundant_Velocity"=w1979, "CorrectedRed_PB"=w1980, "UncorrectedAvgVel_PB"=w1982, "avgVel_PB"=w1981, "Frag Rod"="Frag Rod", "V50userExcl"=FALSE) -> (w1958:T7)
        n1176 = Build Array (concatenate)(w1954, w1958) -> (w1941:T6)
        n1177 = flat-sequence {
          tunnel: w1949 -> [w1986]
          tunnel: [w1985] -> w1948
          tunnel: w1941 -> [w1983]
          tunnel: [w1983] -> w1940
          frame #0 {
            n1178 = local write "backdepth"(sgl 0.0 ("BACKFACE DEPTH")) -> ()
            n1179 = property on="shotsTabCntrl" class="TabCtl (strict)"(error in=w1986, "Value"=T5."Shots Table" ("shotsTabCntrl")) -> (error out=w1985:errorcluster)  [unwired: 1 in, 1 out]
          }
        }
      }
      frame "CLEAR SHOTS" {
        # "case # 6"
        # "This section will clear the shot table and re-enable the \"ADD SHOT\" button to get ready for a new test panel."
        n1180 = Two Button Dialog(message="Shot table cleared even if not saved. Are you sure?", 1:"NO" ("F button name (\"Cancel\")"), 2:"YES" ("T button name (\"OK\")")) -> (T button?=w1995:bool)
        n1181 = case shown="True" w1995 {
          tunnel: [w2001 T6 [{"Uncorrected Impact"=0.0, "Uncorrected Residual"=0.0, "avgVel_PB"=0.0, "IMPACT VELOCITY"=0.0, "RESIDUAL  VELOCITY "=0.0, "Shot Description"="", "Powder Loading "=0.0, "Barrel Temperature"=0.0, "TIME / DATE"="", "shot order"=1, "SHOT STATUS"=1, "Shot Angle"=0, "Corrected Impact"=0.0, "Corrected residual"=0.0, "Projectile Mass"=0.0, "usedv50"=FALSE, "Energy Loss (J)"=0.0, "BackFace\nDepth"=0.0, "BackFace\nDiameter"=0.0, "Redundant_Velocity"=0.0, "velLoss_PB"=0.0, "strikeVel_PB"=0.0, "UncorrectedRed_PB"=0.0, "CorrectedRed_PB"=0.0, "UncorrectedAvgVel_PB"=0.0, "V50userExcl"=FALSE, "Frag Rod"=0.0}] ("shotsArr")] -> w2000
          tunnel: w1996 -> [w2001 _]
          frame False {
          }
          frame True {
            w2003 = T15."Disabled and Grayed Out" ("Disabled")
            n1182 = invoke on="Table of Shots" class="Tbl (strict)" method="Reinit To Default"() -> ()  [unwired: 3 in, 3 out]
            n1183 = property on="addShot" class="Bool"("Disabled"=T15."Enabled") -> ()  [unwired: 2 in, 2 out]
            n1184 = invoke on="shotsArr" class="Arr (strict)" method="Reinit To Default"() -> ()  [unwired: 3 in, 3 out]
            n1185 = property on="saveReq" class="Str"("Visible"=TRUE) -> ()  [unwired: 2 in, 2 out]
            n1186 = property on="clearShots" class="Bool"("Disabled"=w2003) -> ()  [unwired: 2 in, 2 out]
            n1187 = property on="undoLastShot" class="Bool"("Disabled"=w2003) -> ()  [unwired: 2 in, 2 out]
            n1188 = property on="saveShots" class="Bool"("Disabled"=w2003) -> ()  [unwired: 2 in, 2 out]
          }
        }
      }
      frame "NEXT SHOT" {
        # "case # 7"
        n1189 = property on="shotsArr" class="Arr (strict)"(error in=w2009) -> (error out=w2008:errorcluster, "Index Values"=w2013:u32[])  [unwired: 1 in, 1 out]
        n1190 = Array Size(array=w2006) -> (size(s)=w2016:i32)
        n1191 = Index Array "Index Array"(array=w2013) -> (element=w2018:u32)  [unwired: 1 in]
        n1192 = To Unsigned Long Integer(number=w2016) -> (unsigned 32bit integer=w2012:u32)
        n1193 = Increment(x=w2018) -> (x+1=w2017:u32)
        n1194 = Quotient & Remainder(x=w2017, y=w2012) -> (x-y*floor(x/y)=w2015:u32)  [unwired: 1 out]
        n1195 = Replace Array Subset "Replace Array Subset"(array=w2013, new element=w2015) -> (w2014:u32[])  [unwired: 1 in]
        n1196 = property on="shotsArr" class="Arr (strict)"(error in=w2008, "Index Values"=w2014) -> (error out=w2007:errorcluster)  [unwired: 1 in, 1 out]
      }
      frame "DELETE SHOT" {
        # "case # 8"
        # "This section undoes new shot data OR deletes the currently accessed previous shot"
        n1197 = local read "deleteShot"() -> (w2025:bool)
        n1198 = case shown="False" w2025 {
          tunnel: w2024 -> [w2029 w2040]
          tunnel: [w2030 w2041] -> w2021
          frame False {
            n1199 = Array Size(array=w2029) -> (size(s)=w2027:i32)
            n1200 = while {
              tunnel: [w2031] -> w2028
              tunnel: w2027 -> [w2033]
              tunnel: w2029 -> [w2035] mode=indexing
              i -> [w2031]
              stop <- w2034 stop-if-true
              n1201 = Unbundle By Name(w2035) -> ("shot order"=w2032:i32)
              n1202 = Equal?(x=w2032, y=w2033) -> (x = y?=w2034:bool)
            }
            n1203 = Delete From Array "Delete From Array"(array=w2029, index=w2028) -> (array with subset deleted=w2030:T6)  [unwired: 1 in, 1 out]
            n1204 = property on="undoLastShot" class="Bool"("Disabled"=T15."Disabled and Grayed Out") -> ()  [unwired: 2 in, 2 out]
          }
          frame True {
            n1205 = property on="shotsArr" class="Arr (strict)"() -> ("Index Values"=w2049:u32[])  [unwired: 2 in, 2 out]
            n1206 = local write "deleteShot"(FALSE) -> ()
            n1207 = Index Array(array=w2049, index=0 ("Index")) -> (element=w2039:u32)
            n1208 = To Long Integer(number=w2039) -> (32bit integer=w2036:i32)
            n1209 = Index Array(array=w2040, index=w2036) -> (element=w2038:T7)
            n1210 = Unbundle By Name(w2038) -> ("shot order"=w2037:i32)
            n1211 = Format Into String(format string="The currently displayed Shot, #%d", w2037) -> (resulting string=w2046:string)  [unwired: 2 in, 1 out]
            n1212 = Concatenate Strings(w2046, ", will be deleted.  IT CANNOT RECOVERED!  Do you want to DELETE the shot?" ("message")) -> (w2045:string)
            n1213 = Two Button Dialog(message=w2045, 1:"NO I do NOT want to delete.  Cancel Request" ("F button name (\"Cancel\")"), 2:"YES I want to delete the shot" ("T button name (\"OK\")")) -> (T button?=w2052:bool)
            n1214 = case shown="True" w2052 {
              tunnel: w2040 -> [w2065 w2068]
              tunnel: [w2065 w2070] -> w2043
              tunnel: w2036 -> [_ w2067]
              tunnel: [10000 ("shot order") w2069] -> w2042
              frame False {
              }
              frame True {
                n1215 = Index Array(array=w2068, index=w2067) -> (element=w2066:T7)
                n1216 = Unbundle By Name(w2066) -> ("shot order"=w2069:i32)
                n1217 = Delete From Array(array=w2068, index=w2067) -> (array with subset deleted=w2070:T6)  [unwired: 1 in, 1 out]
              }
            }
            n1218 = for {
              tunnel: [w2059] -> w2041 mode=indexing
              tunnel: w2043 -> [w2054] mode=indexing
              tunnel: w2042 -> [w2058]
              n1219 = Unbundle By Name(w2054) -> ("shot order"=w2056:i32)
              n1220 = Decrement(x=w2056) -> (x-1=w2055:i32)
              n1221 = Greater?(x=w2056, y=w2058) -> (0:w2057:bool)
              n1222 = case shown="True" w2057 {
                tunnel: w2055 -> [_ w2062]
                tunnel: w2054 -> [w2060 w2063]
                tunnel: [w2060 w2061] -> w2059
                frame False {
                }
                frame True {
                  n1223 = Bundle By Name(cluster=w2063, "shot order"=w2062) -> (w2061:T7)
                }
              }
            }
          }
        }
        n1224 = property on="shotsArr" class="Arr (strict)"(error in=w2020, "Val(Sgnl)"=w2021) -> (error out=w2019:errorcluster)  [unwired: 1 in, 1 out]
      }
      frame "READY CLOCK" {
        # "case # 9"
        n1225 = case shown="\"Screens\"" "MeasSrc" {
          tunnel: w2072 -> [w2079 w2084 w2086]
          tunnel: [w2077 w2084 w2086] -> w2071
          frame "Simulated", Default {
            n1226 = flat-sequence {
              tunnel: w2079 -> [w2080]
              tunnel: [w2080] -> w2078
              tunnel: [w2082] -> w2077
              tunnel: w2078 -> [w2082]
              frame #0 {
                n1227 = local write "readyClock"(FALSE ("RANGE RESET")) -> ()
              }
              frame #1 {
                n1228 = Wait (ms)(milliseconds to wait=u32 100) -> ()  [unwired: 1 out]
              }
            }
          }
          frame "Radar" {
          }
          frame "Screens" {
            n1229 = local write "readyClock"(FALSE ("RANGE RESET")) -> ()
          }
        }
      }
      frame "PROC SHOTS" {
        # "case # 10"
        n1230 = local write "processShots"(FALSE ("ProcessShots")) -> ()
        n1231 = local read "Drag Corrected"() -> (w2092:bool)
        n1232 = stacked-sequence {
          seq-local: [_ w2150 _ _] -> [_ _ w2183 w2233]
          seq-local: [w2095 _ _ _] -> [_ w2146 _ _]
          seq-local: [w2113 _ _ _] -> [_ w2147 _ _]
          seq-local: [w2114 _ _ _] -> [_ w2148 _ _]
          tunnel: [_ _ _ w2226] -> w2093
          tunnel: w2092 -> [w2116 w2149 _ _]
          tunnel: w2089 -> [_ w2145 _ _]
          tunnel: w2088 -> [w2112 _ _ _]
          tunnel: [w2112 _ _ _] -> w2087
          frame #0 {
            n1233 = disable-structure "Diagram Disable Structure" shown="Enabled" {
              disable-tunnel: [w2133 w2140] -> w2121
              frame Disabled {
                n1234 = local read "factor array"() -> (w2135:sgl[])
                n1235 = local read "Threat"() -> (w2132:u16)
                n1236 = To Long Integer(number=w2132) -> (32bit integer=w2134:i32)
                n1237 = Index Array(array=w2135, index=w2134) -> (element=w2133:sgl)
              }
              frame Enabled {
                n1238 = local read "threatDetails"() -> (w2139:T1)
                n1239 = Unbundle By Name(w2139) -> ("dragCorrection"=w2137:string)
                n1240 = Not Equal?(x=w2137, y="") -> (x != y?=w2138:bool)
                n1241 = case shown="True" w2138 {
                  tunnel: [sgl 1.0 ("default value 1") w2143] -> w2140
                  tunnel: w2137 -> [_ w2142]
                  frame False {
                  }
                  frame True {
                    n1242 = Scan From String(input string=w2142, default 1=sgl 0.0 ("default value 1")) -> (output 1=w2143:sgl)  [unwired: 3 in, 3 out]
                  }
                }
              }
            }
            "correction coefficient" <- w2121
            n1243 = local read "Current/avg/speed"() -> (w2117:sgl)
            n1244 = local read "mid_to_targ_dist"() -> (w2118:sgl)
            n1245 = local read "lengthUnits"() -> (w2115:string)
            n1246 = call "Compute Strike Velocity.vi"("drag coefficient"=w2121, "decay distance"=w2118, "raw velocity"=w2117, "distance units"=w2115) -> ("correction factor"=w2095:sgl, "strike velocity"=w2119:sgl)  [unwired: 1 out]
            "DC_ factor" <- w2095
            "Corrected Average" <- w2119
            n1247 = call "Velocity Correction.vi"("raw impact"="MeasVelScrnSet1", "distance units"=w2115, "raw redundant"="MeasVelScrnSet2", "raw residual"="Current/residual/speed", "screen set midpt to target"="Set#1_to_Target", "residual screen to target"="Residual/Target Dist", "correction coefficient"=w2121) -> ("corrected impact"=w2126:sgl, "corrected redundant"=w2122:sgl, "corrected residual"=w2124:sgl, "impact factor"=w2113:sgl, "conversion factor"=→"conversion factor":sgl, "residual factor"=w2114:sgl)  [unwired: 3 out]
            "Residual factor" <- w2114
            "Impact factor" <- w2113
            "CorrectedVelScrnSet1" <- w2126
            "Corrected Residual" <- w2124
            "CorrectedVelScrnSet2" <- w2122
            n1248 = Select(t=w2122, s=w2116, f="MeasVelScrnSet2") -> (s? t:f=→"Redundant/speed":sgl)
            n1249 = Select(t=w2119, s=w2116, f=w2117) -> (s? t:f=→"Avg/speed":sgl)
            n1250 = Select(t=w2126, s=w2116, f="MeasVelScrnSet1") -> (s? t:f=→"Impact/speed":sgl)
            n1251 = Select(t=w2124, s=w2116, f="Current/residual/speed") -> (s? t:f=→"residual/speed":sgl)
            n1252 = Add(x="MeasVelScrnSet2", y="MeasVelScrnSet1") -> (x+y=w2099:sgl)
            n1253 = Subtract(x="MeasVelScrnSet2", y="MeasVelScrnSet1") -> (x-y=w2098:sgl)
            n1254 = Divide(x=w2099, y=sgl 200.0) -> (x/y=w2100:sgl)
            n1255 = Divide(x=w2098, y=w2100) -> (x/y=w2104:sgl)
            "%_Difference" <- w2104
            n1256 = Absolute Value(x=w2104) -> (abs(x)=w2106:sgl)
            n1257 = Less?(x=w2106, y="percent warning") -> (x < y?=w2111:bool)
            n1258 = Select(t=u32 65343, s=w2111, f=u32 15668992) -> (s? t:f=w2107:u32)
            n1259 = Select(t=u32 0, s=w2111, f=u32 16777226) -> (s? t:f=w2110:u32)
            n1260 = property on="%_Difference" class="DigNum (strict)"("Numeric Text.Text Colors:BG Color"=w2107, "NumText.TextColor"=w2110) -> ()  [unwired: 2 in, 2 out]
          }
          frame #1 {
            # "<-- DC_factor (for Average of impact and redundant)"
            # "IF drag corrected THEN apply factors"
            # "Residual factor"
            # "Impact factor\n(also applies to\nredundant velocity)"
            n1261 = for {
              tunnel: w2145 -> [w2161] mode=indexing
              tunnel: w2148 -> [w2170]
              tunnel: w2147 -> [w2165]
              tunnel: w2149 -> [w2159]
              tunnel: [w2172] -> w2150 mode=indexing
              tunnel: w2146 -> [w2155]
              n1262 = Unbundle By Name(w2161) -> ("UncorrectedAvgVel_PB"=w2160:sgl)
              n1263 = Unbundle By Name(w2161) -> ("UncorrectedRed_PB"=w2167:sgl)
              n1264 = Unbundle By Name(w2161) -> ("Uncorrected Impact"=w2164:sgl)
              n1265 = Unbundle By Name(w2161) -> ("Uncorrected Residual"=w2169:sgl)
              n1266 = Multiply(x=w2155, y=w2160) -> (x*y=w2157:sgl)
              n1267 = Multiply(x=w2165, y=w2167) -> (x*y=w2166:sgl)
              n1268 = Multiply(x=w2165, y=w2164) -> (x*y=w2156:sgl)
              n1269 = Multiply(x=w2170, y=w2169) -> (x*y=w2162:sgl)
              n1270 = Select(t=w2157, s=w2159, f=w2160) -> (s? t:f=w2158:sgl)
              n1271 = Select(t=w2166, s=w2159, f=w2167) -> (s? t:f=w2168:sgl)
              n1272 = Select(t=w2162, s=w2159, f=w2169) -> (s? t:f=w2171:sgl)
              n1273 = Select(t=w2156, s=w2159, f=w2164) -> (s? t:f=w2163:sgl)
              n1274 = Subtract(x=w2158, y=w2157) -> (x-y=w2152:sgl)
              n1275 = Not A Number/Path/Refnum?(number/path/refnum=w2152) -> (NaN/Path/Refnum?=w2154:bool)
              n1276 = Select(t=sgl 0.0, s=w2154, f=w2152) -> (s? t:f=w2151:sgl)
              n1277 = Bundle By Name(cluster=w2161, "velLoss_PB"=w2151, "strikeVel_PB"=w2157, "avgVel_PB"=w2158, "CorrectedRed_PB"=w2166, "Redundant_Velocity"=w2168, "Corrected Impact"=w2156, "IMPACT VELOCITY"=w2163, "Corrected residual"=w2162, "RESIDUAL  VELOCITY"=w2171) -> (w2172:T7)
            }
          }
          frame #2 {
            w2184 = sgl[] [] ("Partial")
            # "June 2012\n- Lucas Louriero requested \nstdev of velocities used in V50"
            # "This section calculates the V50"
            n1278 = for {
              shift-right: [w2208] -> w2186
              shift-left: w2184 -> [w2209]
              shift-right: [w2206] -> w2185
              shift-left: w2184 -> [w2207]
              tunnel: w2183 -> [w2200] mode=indexing
              n1279 = Unbundle By Name(w2200) -> ("SHOT STATUS"=w2205:u16)
              n1280 = Unbundle By Name(w2200) -> ("V50userExcl"=w2199:bool)
              n1281 = Unbundle By Name(w2200) -> ("IMPACT VELOCITY"=w2204:sgl)
              n1282 = Unbundle By Name(w2200) -> ("strikeVel_PB"=w2203:sgl)
              n1283 = Select(t=w2203, s="ScreenSetAvgg", f=w2204) -> (s? t:f=w2202:sgl)
              n1284 = case shown="False" w2199 {
                tunnel: w2209 -> [w2215 w2225]
                tunnel: [w2214 w2225] -> w2208
                tunnel: w2207 -> [w2213 w2224]
                tunnel: [w2212 w2224] -> w2206
                tunnel: w2205 -> [w2211 _]
                tunnel: w2202 -> [w2210 _]
                frame False {
                  n1285 = case shown="1" w2211 {
                    tunnel: w2210 -> [w2216 w2220]
                    tunnel: [w2219 w2221] -> w2214
                    tunnel: w2215 -> [w2218 w2221]
                    tunnel: w2213 -> [w2217 w2223]
                    tunnel: [w2217 w2222] -> w2212
                    frame 0, Default {
                      n1286 = Build Array (concatenate)(w2218, w2216) -> (w2219:sgl[])
                    }
                    frame 1 {
                      n1287 = Build Array (concatenate)(w2223, w2220) -> (w2222:sgl[])
                    }
                  }
                }
                frame True {
                }
              }
            }
            n1288 = Sort 1D Array(array=w2186) -> (sorted array=w2198:sgl[])
            n1289 = Sort 1D Array(array=w2185) -> (sorted array=w2191:sgl[])
            "Complete" <- w2191
            n1290 = Reverse 1D Array(array=w2198) -> (reversed array=w2189:sgl[])
            "Partial" <- w2189
            n1291 = Array Size(array=w2191) -> (size(s)=→"#_completes":i32)
            n1292 = Array Size(array=w2189) -> (size(s)=→"#_partials":i32)
            n1293 = Array Max & Min(array=w2189) -> (max value=w2195:sgl)  [unwired: 3 out]
            n1294 = Array Max & Min(array=w2191) -> (min value=w2193:sgl)  [unwired: 3 out]
            n1295 = call "Compute V50.vi"("Partial"=w2189, "Maximum Deviation"="maxDev", "Complete"=w2191) -> ("velSTDEV"=→"velSTDEV":sgl, "Pairs"=→"Pairs":i16, "zmr"=w2174:sgl, "V50"=→"computed_V50":sgl)  [unwired: 1 out]
            "Z.M.R." <- w2174
            n1296 = To Long Integer(number=w2195) -> (32bit integer=→"highPartial":i32)
            n1297 = To Long Integer(number=w2193) -> (32bit integer=→"lowComplete":i32)
            n1298 = Absolute Value(x=w2174) -> (abs(x)=→"zmr 2":sgl)
            n1299 = Less Than 0?(x=w2174) -> (x < 0?=w2177:bool)
            n1300 = Select(t="Low C minus High P", s=w2177, f="ZMR") -> (s? t:f=w2180:string)
            n1301 = Select(t=u32 65336, s=w2177, f=u32 16755266) -> (s? t:f=w2181:u32)
            n1302 = property on="zmr 2" class="DigNum (strict)"("Caption.Text"=w2180, "Numeric Text.Text Colors:BG Color"=w2181) -> ()  [unwired: 2 in, 2 out]
          }
          frame #3 {
            n1303 = local read "Pairs"() -> (w2238:i16)
            n1304 = Sort 1D Array(array=w2233) -> (sorted array=w2236:T7[])
            n1305 = for {
              tunnel: w2236 -> [w2286] mode=indexing
              tunnel: w2238 -> [w2296]
              shift-right: [w2295] -> _
              shift-left: i16 0 -> [w2294]
              tunnel: [w2288] -> w2234 mode=indexing
              # "this section marks the lowest completes that are used in V50"
              n1306 = Unbundle By Name(w2286) -> ("SHOT STATUS"=w2292:u16, "Projectile Mass"=w2290:sgl, "avgVel_PB"=w2289:sgl, "RESIDUAL  VELOCITY"=w2291:sgl)
              n1307 = Unbundle By Name(w2286) -> ("V50userExcl"=w2287:bool)
              n1308 = local read "conversion factor"() -> (w2297:sgl)
              n1309 = case shown="False" w2287 {
                tunnel: w2296 -> [w2308 _]
                tunnel: [w2307 w2317] -> w2295
                tunnel: w2294 -> [w2306 w2317]
                tunnel: [w2305 FALSE] -> w2293
                tunnel: w2292 -> [w2304 _]
                frame False {
                  n1310 = case shown="1" w2304 {
                    tunnel: w2308 -> [_ w2315]
                    tunnel: [FALSE w2314] -> w2305
                    tunnel: [w2310 w2313] -> w2307
                    tunnel: w2306 -> [w2310 w2311]
                    frame 0, Default {
                    }
                    frame 1 {
                      n1311 = Less?(x=w2311, y=w2315) -> (x < y?=w2314:bool)
                      n1312 = Add(x=w2311, y=i16 1 ("t")) -> (x+y=w2313:i16)
                    }
                  }
                }
                frame True {
                }
              }
              n1313 = Multiply(x=w2297, y=w2291) -> (x*y=w2298:sgl)
              n1314 = Multiply(x=w2289, y=w2297) -> (x*y=w2299:sgl)
              n1315 = Multiply(x=w2299, y=w2299) -> (x*y=w2303:sgl)
              n1316 = Multiply(x=w2298, y=w2298) -> (x*y=w2302:sgl)
              n1317 = Subtract(x=w2303, y=w2302) -> (x-y=w2301:sgl)
              n1318 = Compound Arithmetic op=MULTIPLY(w2290, w2301, sgl 0.0005 ("Input")) -> (w2284:sgl)
              n1319 = Not A Number/Path/Refnum?(number/path/refnum=w2284) -> (NaN/Path/Refnum?=w2285:bool)
              n1320 = Select(t=sgl 0.0, s=w2285, f=w2284) -> (s? t:f=w2282:sgl)
              n1321 = Bundle By Name(cluster=w2286, "usedv50"=w2293, "Energy Loss (J)"=w2282) -> (w2288:T7)
            }
            n1322 = Reverse 1D Array(array=w2234) -> (reversed array=w2235:T7[])
            n1323 = for {
              tunnel: w2235 -> [w2258] mode=indexing
              tunnel: w2238 -> [w2265]
              shift-right: [w2263] -> _
              shift-left: i16 0 -> [w2264]
              tunnel: [w2261] -> w2226 mode=indexing
              # "chooses highest partials used in v50"
              n1324 = Unbundle By Name(w2258) -> ("SHOT STATUS"=w2266:u16, "usedv50"=w2260:bool)
              n1325 = Unbundle By Name(w2258) -> ("V50userExcl"=w2259:bool)
              n1326 = case shown="False" w2259 {
                tunnel: w2266 -> [w2272 _]
                tunnel: w2265 -> [w2271 _]
                tunnel: w2264 -> [w2270 w2281]
                tunnel: [w2269 w2281] -> w2263
                tunnel: [w2268 FALSE ("usedv50")] -> w2262
                tunnel: w2260 -> [w2267 _]
                frame False {
                  n1327 = case shown="1" w2272 {
                    tunnel: w2271 -> [w2276 _]
                    tunnel: [w2275 w2279] -> w2268
                    tunnel: w2270 -> [w2273 w2278]
                    tunnel: [w2274 w2278] -> w2269
                    tunnel: w2267 -> [_ w2279]
                    frame 0, Default {
                      n1328 = Less?(x=w2273, y=w2276) -> (x < y?=w2275:bool)
                      n1329 = Add(x=w2273, y=i16 1) -> (x+y=w2274:i16)
                    }
                    frame 1 {
                    }
                  }
                }
                frame True {
                }
              }
              n1330 = Bundle By Name(cluster=w2258, "usedv50"=w2262) -> (w2261:T7)
            }
            n1331 = for {
              shift-right: [w2244] -> w2227
              shift-left: sgl[] [] ("Partial") -> [w2241]
              tunnel: w2226 -> [w2243] mode=indexing
              n1332 = local read "ScreenSetAvgg"() -> (w2248:bool)
              n1333 = Unbundle By Name(w2243) -> ("V50userExcl"=w2242:bool, "usedv50"=w2240:bool)
              n1334 = Unbundle By Name(w2243) -> ("IMPACT VELOCITY"=w2246:sgl)
              n1335 = Unbundle By Name(w2243) -> ("strikeVel_PB"=w2247:sgl)
              n1336 = Select(t=w2247, s=w2248, f=w2246) -> (s? t:f=w2245:sgl)
              n1337 = case shown="False" w2242 {
                tunnel: w2245 -> [w2249 _]
                tunnel: [w2250 w2257] -> w2244
                tunnel: w2241 -> [w2251 w2257]
                tunnel: w2240 -> [w2252 _]
                frame False {
                  n1338 = case shown="False" w2252 {
                    tunnel: w2251 -> [w2253 w2256]
                    tunnel: [w2253 w2255] -> w2250
                    tunnel: w2249 -> [_ w2254]
                    frame False {
                    }
                    frame True {
                      n1339 = Build Array (concatenate)(w2256, w2254) -> (w2255:sgl[])
                    }
                  }
                }
                frame True {
                }
              }
            }
            n1340 = Array Max & Min(array=w2227) -> (max value=w2232:sgl, min value=w2231:sgl)  [unwired: 2 out]
            n1341 = Subtract(x=w2232, y=w2231) -> (x-y=w2230:sgl)
            n1342 = property on="shotsArr" class="Arr (strict)"("Val(Sgnl)"=w2226) -> ()  [unwired: 2 in, 2 out]
            n1343 = To Long Integer(number=w2230) -> (32bit integer=→"rangeOfResults":i32)
          }
        }
      }
      frame "CHECK DAQ" {
        w2323 = 500  # timeout in ms
        # "case # 11"
        n1344 = Dequeue Element(queue=w2318, timeout in ms (-1)=w2323, error in (no error)=w2319) -> (element=w2322:dbl[], timed out?=w2321:bool, error out=w2320:errorcluster)  [unwired: 1 out]
        n1345 = case shown="False" w2321 {
          tunnel: [Collector_State."PROC SHOTS" ("progState") Collector_State."POLL" ("progState")] -> w2326
          tunnel: [-1 -1 ("index of element")] -> w2325
          tunnel: [w2335 w2379] -> w2324
          tunnel: w2320 -> [w2332 w2379]
          tunnel: w2322 -> [w2333 _]
          frame False {
            n1346 = local read "MeasSrc"() -> (w2334:T12)
            n1347 = case shown="\"Screens\"" w2334 {
              tunnel: w2332 -> [w2340 w2359 w2370]
              tunnel: [w2340 w2359 w2375] -> w2335
              tunnel: w2333 -> [_ _ w2374]
              tunnel: [w2339 w2358 w2361] -> w2330
              tunnel: [w2338 w2357 w2360] -> w2329
              frame "Simulated", Default {
                # "Simulated"
                n1348 = local read "minV50"() -> (w2344:i32)
                n1349 = local read "Powder Loading"() -> (w2356:sgl)
                n1350 = Wait (ms)(milliseconds to wait=u32 500 ("number")) -> ()  [unwired: 1 out]
                n1351 = To Single Precision Float(number=w2344) -> (single precision float=w2343:sgl)
                n1352 = call "Get Shell Speed.vi"("loading"=w2356, "v50"=w2343) -> ("impact"=w2339:sgl, "residual"=w2351:sgl)  [unwired: 1 in, 2 out]
                n1353 = Greater Than 0?(x=w2351) -> (x > 0?=w2353:bool)
                n1354 = local write "Current/residual/speed"(w2351) -> ()
                n1355 = Select(t=u16 1, s=w2353, f=u16 0) -> (s? t:f=w2352:u16)
                n1356 = local write "Current/shotstatus"(w2352) -> ()
                n1357 = Random Number (0-1)() -> (number: 0 to 1=w2349:dbl)
                n1358 = To Single Precision Float(number=w2349) -> (single precision float=w2345:sgl)
                n1359 = Multiply(x=w2345, y=sgl 0.002) -> (x*y=w2348:sgl)
                n1360 = local write "readyClock"(TRUE ("RANGE RESET")) -> ()
                n1361 = Add(x=w2348, y=sgl 0.999) -> (x+y=w2346:sgl)
                n1362 = Multiply(x=w2339, y=w2346) -> (x*y=w2338:sgl)
              }
              frame "Radar" {
                # "Radar -- (future)"
                n1363 = local read "MeasVelScrnSet1"() -> (w2358:sgl)
                n1364 = local read "MeasVelScrnSet2"() -> (w2357:sgl)
              }
              frame "Screens" {
                # "This section checks to see if the counters have been fired.  If they have then the counter times are read"
                n1365 = To Single Precision Float(number=w2374) -> (single precision float=w2373:sgl[])
                n1366 = Index Array(array=w2373) -> (element #1=w2369:sgl, element #2=w2368:sgl)  [unwired: 2 in]
                n1367 = Equal To 0?(x=w2369) -> (x = 0?=w2367:bool)
                n1368 = Equal To 0?(x=w2368) -> (x = 0?=w2363:bool)
                n1369 = local read "Set#1 Separation"() -> (w2372:sgl)
                n1370 = local read "Set#2 Separation"() -> (w2371:sgl)
                n1371 = Divide(x=w2372, y=w2369) -> (x/y=w2365:sgl)
                n1372 = Divide(x=w2371, y=w2368) -> (x/y=w2362:sgl)
                n1373 = Select(t=sgl 0.0, s=w2367, f=w2365) -> (s? t:f=w2361:sgl)
                n1374 = Select(t=sgl 0.0, s=w2363, f=w2362) -> (s? t:f=w2360:sgl)
                n1375 = case shown="No Error" w2370 {
                  selector: w2370 -> [w2378 _]
                  frame No Error {
                    # "=false"
                    n1376 = Unbundle By Name(w2378) -> ("status"=w2377:bool)
                    n1377 = Not(x=w2377) -> (.not. x?=w2376:bool)
                    n1378 = local write "readyClock"(w2376) -> ()
                  }
                  frame Error {
                  }
                }
                n1379 = call <vilib>:"Simple Error Handler.vi"("error in (no error)"=w2370) -> ("error out"=w2375:errorcluster)  [unwired: 1 in, 7 out]
              }
            }
            n1380 = control-ref of="2ndScreen"() -> (w2331:refnum<vi>)
            n1381 = call "2nd screen effect (SubVI).vi"("MeasVelScrnSet 2"=w2329, "MeasVelScrnSet 1"=w2330, "2nd Screen ref"=w2331) -> ("MeasVelOut"=→"Current/avg/speed":sgl)
            n1382 = local write "MeasVelScrnSet1"(w2330) -> ()
            n1383 = local write "MeasVelScrnSet2"(w2329) -> ()
          }
          frame True {
            # "timeout expired"
          }
        }
      }
    }
    "SMErr" <- w550
    "progState" <- w549
    n1384 = disable-structure shown="Disabled" {
      disable-tunnel: w550 -> [w559 _]
      disable-tunnel: w549 -> [w558 _]
      frame Disabled {
        n1385 = flat-sequence {
          tunnel: w558 -> [_]
          tunnel: w559 -> [_]
          frame #0 {
            n1386 = Wait (ms)(milliseconds to wait=u32 1) -> ()  [unwired: 1 out]
          }
          frame #1 {
            n1387 = property on="progState" class="Enum (strict)"() -> ("RingText.Text"=w564:string)  [unwired: 2 in, 2 out]
            n1388 = Get Date/Time In Seconds() -> (seconds since 1Jan1904=w562:timestamp)
            n1389 = Format Date/Time String(seconds (now)=w562) -> (date/time string=w561:string)  [unwired: 2 out]
            n1390 = Build Array(w561, "," ("element"), w564) -> (w565:string[])
            n1391 = call-poly <vilib>:"Write To Spreadsheet File.vi"("append to file? (new file:F)"=TRUE, "1D data"=w565, "file path (dialog if empty)"=path "C:/state.txt") -> ()  [unwired: 5 in, 1 out]
          }
        }
      }
      frame Enabled {
      }
    }
    n1392 = Wait (ms)(milliseconds to wait=u32 50 ("millisecond timer value")) -> ()  [unwired: 1 out]
  }
  n1393 = while "Arming Loop" {
    tunnel: w3 -> [w2406]
    shift-right: [w2404] -> w20
    shift-left: w21 -> [w2405]
    shift-right: [w2398] -> w11
    shift-left: w1 -> [w2402]
    shift-right: [w2399] -> w12
    shift-left: w2 -> [w2403]
    shift-right: [w2393] -> w13
    shift-left: w10 -> [w2401]
    shift-right: [w2392] -> w14
    shift-left: w9 -> [w2400]
    stop <- "close arming loop" stop-if-true
    w2396 = 10.0  # timeout
    # "error code -200474\ntimeout expired"
    n1394 = call-poly <vilib>:"DAQmx Read.vi"("task/channels in"=w2402, "timeout"=w2396, "error in"=w2400) -> ("task out"=w2398:refnum<k21>, "data"=w2394:dbl, "error out"=w2389:errorcluster)  [unwired: 10 in]
    n1395 = call-poly <vilib>:"DAQmx Read.vi"("task/channels in"=w2403, "timeout"=w2396, "error in"=w2401) -> ("task out"=w2399:refnum<k21>, "data"=w2395:dbl, "error out"=w2387:errorcluster)  [unwired: 10 in]
    n1396 = Unbundle By Name(w2387) -> ("code"=w2384:i32)
    n1397 = Unbundle By Name(w2389) -> ("code"=w2388:i32)
    n1398 = Equal?(x=w2384, y=-200474) -> (x = y?=w2383:bool)
    n1399 = Equal?(x=w2388, y=-200474) -> (x = y?=w2391:bool)
    n1400 = Or(x=w2383, y=w2391) -> (x .or. y?=w2386:bool)
    n1401 = case shown="False" w2386 {
      tunnel: w2406 -> [w2415 _]
      tunnel: w2405 -> [w2414 w2420]
      tunnel: [w2413 w2420] -> w2404
      tunnel: w2395 -> [w2411 _]
      tunnel: w2394 -> [w2410 _]
      frame False {
        n1402 = Build Array(w2411, w2410) -> (w2412:dbl[])
        n1403 = Enqueue Element(queue=w2415, element=w2412, error in (no error)=w2414) -> (queue out=w2408:refnum<queue>, error out=w2413:errorcluster)  [unwired: 1 in, 1 out]
        n1404 = for {
          N: 10 -> [w2418]
          tunnel: w2408 -> [_]
          i -> [w2417]
          n1405 = Subtract(x=w2418, y=w2417) -> (x-y=→"cntDn":i32)
          n1406 = Wait (ms)(milliseconds to wait=u32 1000) -> ()  [unwired: 1 out]
        }
        "ARMED" <- FALSE ("ARMED")
      }
      frame True {
      }
    }
    n1407 = local write "ARMED"(TRUE ("ARMED")) -> ()
    n1408 = case shown="No Error" w2387 {
      selector: w2387 -> [w2424 w2426]
      tunnel: [w2424 errorcluster {"status"=FALSE, "code"=0, "source"=""} ("error IO")] -> w2393
      frame No Error {
      }
      frame Error {
        "errCtr0" <- w2426
      }
    }
    n1409 = case shown="Error" w2389 {
      selector: w2389 -> [w2421 w2423]
      tunnel: [w2421 errorcluster {"status"=FALSE, "code"=0, "source"=""} ("error IO")] -> w2392
      frame No Error {
      }
      frame Error {
        "errCtr1" <- w2423
      }
    }
  }
  n1410 = call <vilib>:"DAQmx Clear Task.vi"("task in"=w11, "error in"=w14) -> ("error out"=w17:errorcluster)  [unwired: 13 in]
  n1411 = call <vilib>:"DAQmx Clear Task.vi"("task in"=w12, "error in"=w13) -> ("error out"=w18:errorcluster)  [unwired: 13 in]
  n1412 = Release Queue(queue=w3, force destroy? (F)=TRUE, error in (no error)=w20) -> (error out=w15:errorcluster)  [unwired: 2 out]
  n1413 = Merge Errors(w18, w17, w15) -> (w19:errorcluster)
  n1414 = call <vilib>:"General Error Handler.vi"("type of dialog (OK msg:1)"=w16, "error in (no error)"=w19) -> ()  [unwired: 9 in, 5 out]
